vi "Algorithms.vi"(0 "Algo In":T2 {"Measurement ROI.Measurement ROI array"."Multi Threshold Data"."Replace Value" format="%.2f"; "Measurement ROI.Measurement ROI array"."Multi Threshold Data"."Upper value" format="%.2f"; "Measurement ROI.Measurement ROI array"."Multi Threshold Data"."Lower value" format="%.2f"; "Measurement ROI.Measurement ROI array"."Edge Options"."Edge Polarity" items=["All Edges", "Rising Edges", "Falling Edges"]; "Measurement ROI.Measurement ROI array"."Edge Options"."Minimum Edge Strength" format="%.2f"; "Measurement ROI.Measurement ROI array"."Edge Options"."Width" step=2; "Measurement ROI.Measurement ROI array"."Edge Options"."Kernel Size" step=2; "Measurement ROI.Measurement ROI array"."Line Options"."Min. Points (%)" min=0.0 max=100.0; "Measurement ROI.Measurement ROI array"."Line Options"."Min. SNR (db)" min=0.0; "Measurement ROI.Measurement ROI array"."Line Options"."Max. Score" min=0.0 max=1024.0; "Measurement ROI.Measurement ROI array"."Line Options"."Min. Score" min=0.0 max=1024.0 step=1.0; "Measurement ROI.Measurement ROI array"."Shape Detection Settings"."Curve Parameters"."Max Endpoint Gap" min=0; "Measurement ROI.Measurement ROI array"."Shape Detection Settings"."Curve Parameters"."Col Search Step Size" min=1 max=255 step=1; "Measurement ROI.Measurement ROI array"."Shape Detection Settings"."Curve Parameters"."Row Search Step Size" min=1 max=255 step=1; "Measurement ROI.Measurement ROI array"."Shape Detection Settings"."Curve Parameters"."Min Length" min=0; "Measurement ROI.Measurement ROI array"."Shape Detection Settings"."Curve Parameters"."Edge Filter Size" items=["Fine", "Normal", "Controur Tracing"]; "Measurement ROI.Measurement ROI array"."Shape Detection Settings"."Curve Parameters"."Edge Threshold" min=1 max=65535 step=1; "Measurement ROI.Measurement ROI array"."Shape Detection Settings"."Curve Parameters"."Extraction Mode" items=["Normal", "Uniform Regions"]; "Measurement ROI.Measurement ROI array"."Shape Detection Settings"."Match Options"."Range Settings"."Match Constraints" items=["Rotation Angle (degrees)", "Scale Factor (%)", "Occlusion (%)"]}, 5 "AlgoOut array IN":T13 {"CircleArrayOUT"."First Edges"."Distance (Real-World)" format="%.2f"; "CircleArrayOUT"."First Edges"."Location (Real-World)"."Y" format="%.2g"; "CircleArrayOUT"."First Edges"."Location (Real-World)"."X" format="%.2f"; "CircleArrayOUT"."First Edges"."Noise" format="%.2f"; "CircleArrayOUT"."First Edges"."Location (Pixel)"."Y" format="%.2g"; "CircleArrayOUT"."First Edges"."Location (Pixel)"."X" format="%.2f"; "CircleArrayOUT"."First Edges"."Strength" format="%.2f"; "CircleArrayOUT"."First Edges"."Distance (Pixel)" format="%.2f"; "Line Array"."Used Edges"."Edge Information"."Distance (Real-World)" format="%.2f"; "Line Array"."Used Edges"."Edge Information"."Location (Real-World)"."Y" format="%.2g"; "Line Array"."Used Edges"."Edge Information"."Location (Real-World)"."X" format="%.2f"; "Line Array"."Used Edges"."Edge Information"."Noise" format="%.2f"; "Line Array"."Used Edges"."Edge Information"."Location (Pixel)"."Y" format="%.2g"; "Line Array"."Used Edges"."Edge Information"."Location (Pixel)"."X" format="%.2f"; "Line Array"."Used Edges"."Edge Information"."Strength" format="%.2f"; "Line Array"."Used Edges"."Edge Information"."Distance (Pixel)" format="%.2f"; "Line Array"."Straight Edges"."Point2 (Real-World)"."Y" format="%.2f"; "Line Array"."Straight Edges"."Point2 (Real-World)"."X" format="%.2f"; "Line Array"."Straight Edges"."Point1 (Real-World)"."Y" format="%.2f"; "Line Array"."Straight Edges"."Point1 (Real-World)"."X" format="%.2f"; "Line Array"."Straight Edges"."Point2 (Pixels)"."Y" format="%.2f"; "Line Array"."Straight Edges"."Point2 (Pixels)"."X" format="%.2f"; "Line Array"."Straight Edges"."Point1 (Pixels)"."Y" format="%.2f"; "Line Array"."Straight Edges"."Point1 (Pixels)"."X" format="%.2f"; "Line Array"."Line"."Point 2"."Y" format="%.2f"; "Line Array"."Line"."Point 2"."X" format="%.2f"; "Line Array"."Line"."Point 1"."Y" format="%.2f"; "Line Array"."Line"."Point 1"."X" format="%.2f"}, 7 "Captured Image Array In":T16(array[cluster]), 9 "Measurement value":T1(array[cluster]), 11 "error in (no error)":errorcluster) -> (4 "AlgoOut Array out":T14 {"CircleArrayOUT"."First Edges"."Distance (Real-World)" format="%.2f"; "CircleArrayOUT"."First Edges"."Location (Real-World)"."Y" format="%.2g"; "CircleArrayOUT"."First Edges"."Location (Real-World)"."X" format="%.2f"; "CircleArrayOUT"."First Edges"."Noise" format="%.2f"; "CircleArrayOUT"."First Edges"."Location (Pixel)"."Y" format="%.2g"; "CircleArrayOUT"."First Edges"."Location (Pixel)"."X" format="%.2f"; "CircleArrayOUT"."First Edges"."Strength" format="%.2f"; "CircleArrayOUT"."First Edges"."Distance (Pixel)" format="%.2f"; "Line Array"."Used Edges"."Edge Information"."Distance (Real-World)" format="%.2f"; "Line Array"."Used Edges"."Edge Information"."Location (Real-World)"."Y" format="%.2g"; "Line Array"."Used Edges"."Edge Information"."Location (Real-World)"."X" format="%.2f"; "Line Array"."Used Edges"."Edge Information"."Noise" format="%.2f"; "Line Array"."Used Edges"."Edge Information"."Location (Pixel)"."Y" format="%.2g"; "Line Array"."Used Edges"."Edge Information"."Location (Pixel)"."X" format="%.2f"; "Line Array"."Used Edges"."Edge Information"."Strength" format="%.2f"; "Line Array"."Used Edges"."Edge Information"."Distance (Pixel)" format="%.2f"; "Line Array"."Straight Edges"."Point2 (Real-World)"."Y" format="%.2f"; "Line Array"."Straight Edges"."Point2 (Real-World)"."X" format="%.2f"; "Line Array"."Straight Edges"."Point1 (Real-World)"."Y" format="%.2f"; "Line Array"."Straight Edges"."Point1 (Real-World)"."X" format="%.2f"; "Line Array"."Straight Edges"."Point2 (Pixels)"."Y" format="%.2f"; "Line Array"."Straight Edges"."Point2 (Pixels)"."X" format="%.2f"; "Line Array"."Straight Edges"."Point1 (Pixels)"."Y" format="%.2f"; "Line Array"."Straight Edges"."Point1 (Pixels)"."X" format="%.2f"; "Line Array"."Line"."Point 2"."Y" format="%.2f"; "Line Array"."Line"."Point 2"."X" format="%.2f"; "Line Array"."Line"."Point 1"."Y" format="%.2f"; "Line Array"."Line"."Point 1"."X" format="%.2f"}, 6 "overlayDetails Out":T12={"Measurment Name"="", "Measurment Type"="", "Measurment Subtype"="", "Angle of rotation"=0.0, "Color"=16860, "Inspect Overlay Coordinate"=[], "Result"=[], "PointForOverlays"={"Line"=[], "Angle"=[], "Circle"=[], "Points"={"Points"=[]}, "Coordinate System"={"Origin"={"X"=0.0, "Y"=0.0}, "Angle (deg)"=0.0, "Axis Reference"=0}, "True position"={"Measurement details"=[], "XY?"=FALSE}}} {"Inspect Overlay Coordinate"."Y" format="%.2f"; "Inspect Overlay Coordinate"."X" format="%.2f"; "PointForOverlays"."Coordinate System"."Axis Reference" items=["Direct", "Indirect"]; "PointForOverlays"."Coordinate System"."Angle (deg)" format="%.2f"; "PointForOverlays"."Coordinate System"."Origin"."Y" format="%.2f"; "PointForOverlays"."Coordinate System"."Origin"."X" format="%.2f"; "PointForOverlays"."Points"."Points"."Y" format="%.2f"; "PointForOverlays"."Points"."Points"."X" format="%.2f"; "PointForOverlays"."Circle"."Point 2"."Y" format="%.2f"; "PointForOverlays"."Circle"."Point 2"."X" format="%.2f"; "PointForOverlays"."Circle"."Point 1"."Y" format="%.2f"; "PointForOverlays"."Circle"."Point 1"."X" format="%.2f"; "PointForOverlays"."Angle"."line2Point2"."Y" format="%.2f"; "PointForOverlays"."Angle"."line2Point2"."X" format="%.2f"; "PointForOverlays"."Angle"."line2Point1"."Y" format="%.2f"; "PointForOverlays"."Angle"."line2Point1"."X" format="%.2f"; "PointForOverlays"."Angle"."line1Point2"."Y" format="%.2f"; "PointForOverlays"."Angle"."line1Point2"."X" format="%.2f"; "PointForOverlays"."Angle"."line1Point1"."Y" format="%.2f"; "PointForOverlays"."Angle"."line1Point1"."X" format="%.2f"; "PointForOverlays"."Angle"."Point 2a"."Y" format="%.2f"; "PointForOverlays"."Angle"."Point 2a"."X" format="%.2f"; "PointForOverlays"."Angle"."Point 1a"."Y" format="%.2f"; "PointForOverlays"."Angle"."Point 1a"."X" format="%.2f"; "PointForOverlays"."Angle"."vertex"."Y" format="%.2f"; "PointForOverlays"."Angle"."vertex"."X" format="%.2f"; "PointForOverlays"."Angle"."Point 2"."Y" format="%.2f"; "PointForOverlays"."Angle"."Point 2"."X" format="%.2f"; "PointForOverlays"."Angle"."Point 1"."Y" format="%.2f"; "PointForOverlays"."Angle"."Point 1"."X" format="%.2f"; "PointForOverlays"."Line"."Point 2"."Y" format="%.2f"; "PointForOverlays"."Line"."Point 2"."X" format="%.2f"; "PointForOverlays"."Line"."Point 1"."Y" format="%.2f"; "PointForOverlays"."Line"."Point 1"."X" format="%.2f"}, 15 "error out":errorcluster)   [LabVIEW 2018]
uses:
  Controls/AlgoOut.ctl
  <vilib>/vision/Measure.llb/Edge New.ctl
  <vilib>/vision/Image Controls.llb/IMAQ Image.ctl
  Controls/AlgoOutArray.ctl
  Overlays/Controls/overlayWithDetails.ctl
  Controls/Algo In.ctl
  Inspection/Controls/Measurement ROI.ctl
  <vilib>/vision/Measure.llb/Edge Options.ctl
  <vilib>/vision/Measure.llb/Edge Polarity.ctl
  <vilib>/vision/Measure.llb/Straight Edge Options.ctl
  <vilib>/vision/Measure.llb/Straight Edge Process.ctl
  <vilib>/vision/Pattern Matching.llb/IMAQ Curve Parameters.ctl
  <vilib>/vision/Shape Detection.llb/ShapeDetectionMatchOptions.ctl
  <vilib>/vision/Pattern Matching.llb/IMAQ Match Range Setting.ctl
  <vilib>/vision/NI_Vision_Development_Module.lvlib
panel:
  # "Range"
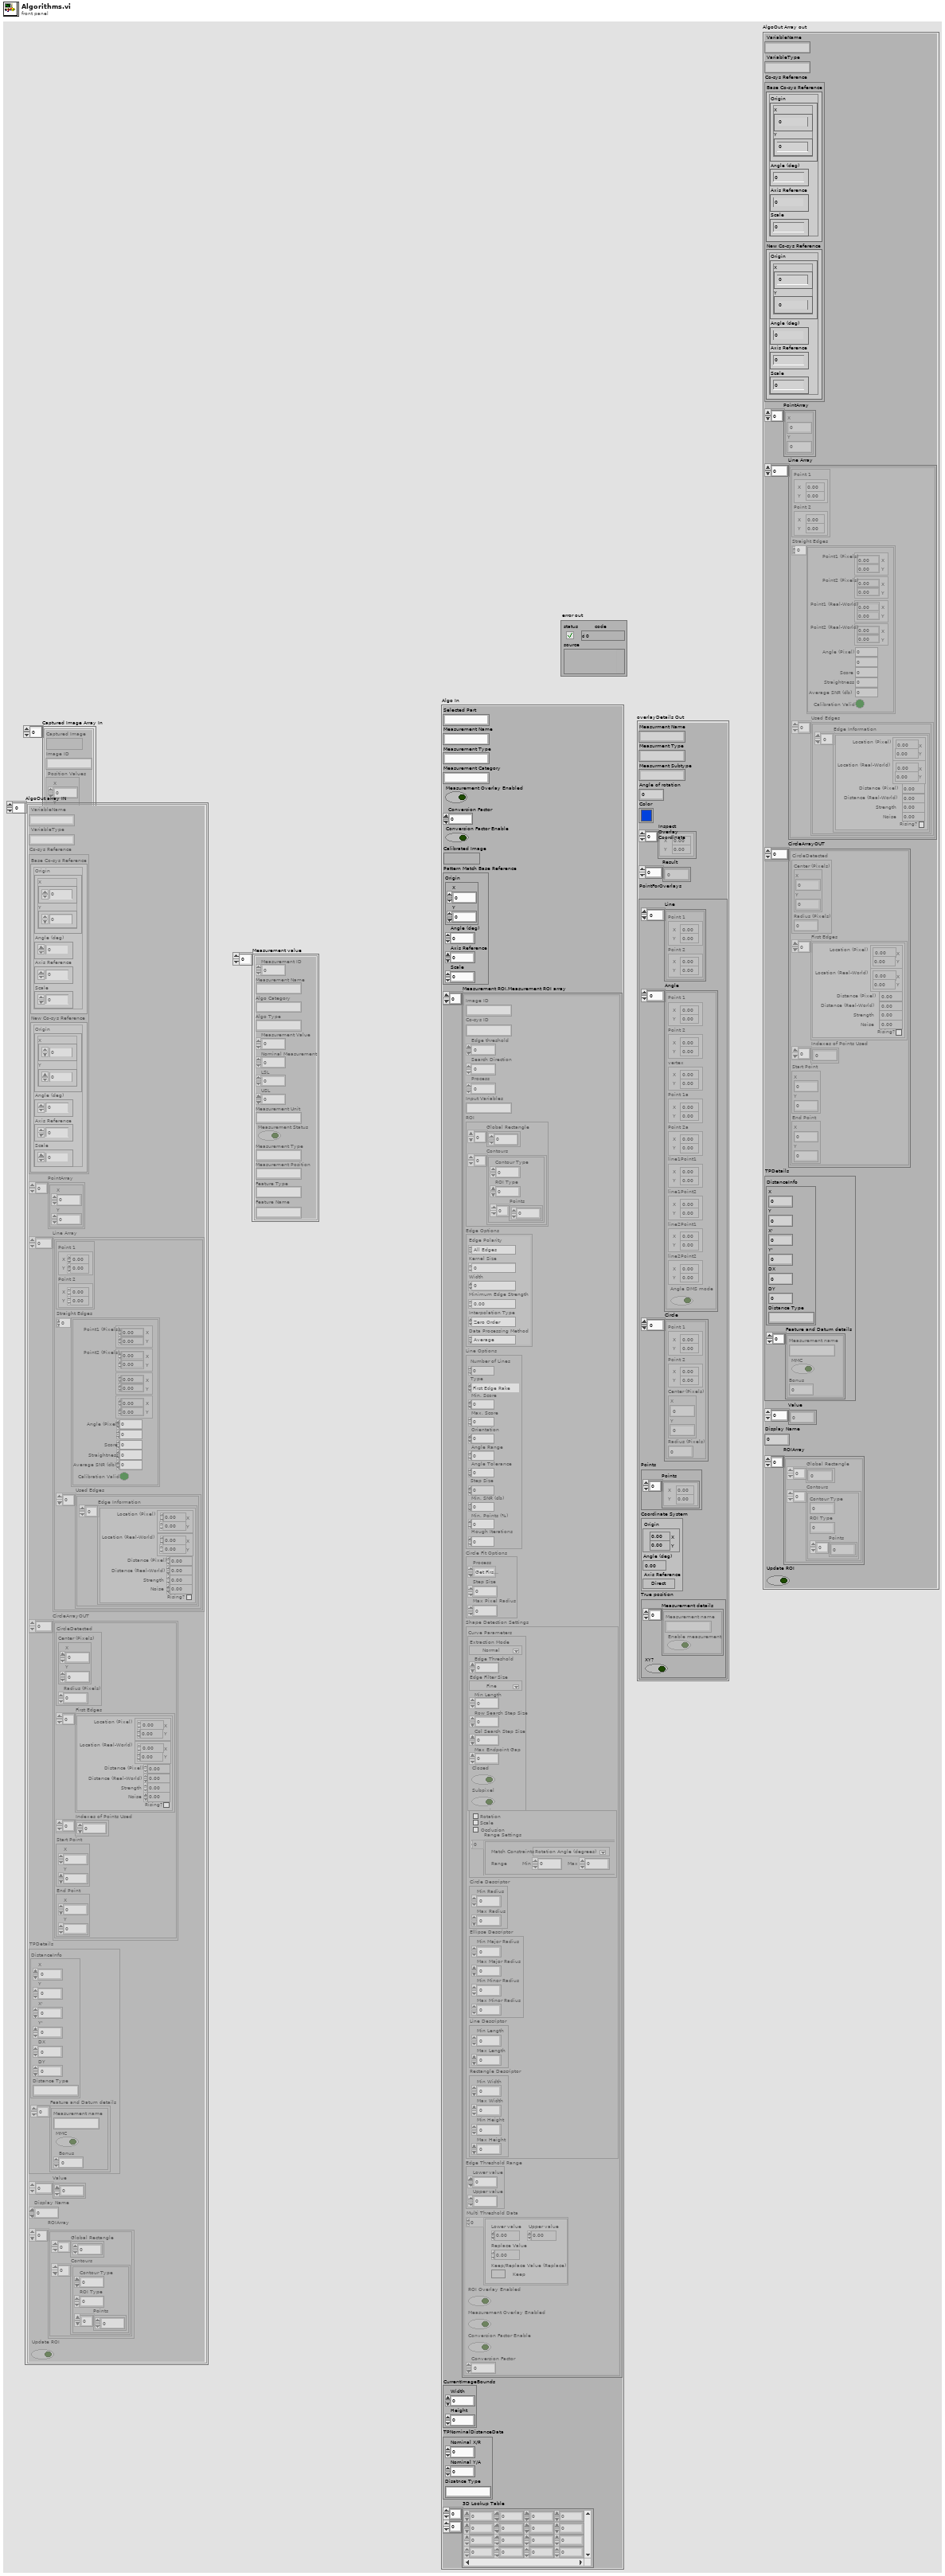
[diagram p1: front panel]
types:
  T1 = cluster{"Measurement ID":u32, "Measurement Name":string, "Algo Category":string, "Algo Type":string, "Measurement Value":dbl, "Nominal Measurement":dbl, "LSL":dbl, "USL":dbl, "Measurement Unit":string, "Measurement Status":bool, "Measurement Type":string, "Measurement Position":string, "Feature Type":string, "Feature Name":string}[]
  T2 = typedef "Algo Sequencer.lvclass/Algo In.ctl" = cluster{"Selected Part":string, "Measurement Name":string, "Measurement Type":string, "Measurement Category":string, "Measurement Overlay Enabled":bool, "Conversion Factor":dbl, "Conversion Factor Enable":bool, "Calibrated Image":T3, "Pattern Match Base Reference":cluster{"Origin":cluster{"X":dbl, "Y":dbl}, "Angle (deg)":dbl, "Axis Reference":dbl, "Scale":dbl}, "Measurement ROI.Measurement ROI array":T4[], "CurrentImageBounds":cluster{"Width":i32, "Height":i32}, "TPNominalDistanceData":cluster{"Nominal X/R":dbl, "Nominal Y/A":dbl, "Disatnce Type":string}, "3D Lookup Table":dbl[][]}
  T3 = typedef "IMAQ Image.ctl" = refnum<image>
  T4 = typedef "Inspection.lvclass/Measurement ROI.ctl" = cluster{"Image ID":string, "Co-sys ID":string, "Edge threshold":dbl, "Search Direction ":u16, "Process":u16, "Input Variables":string, "ROI":cluster{"Global Rectangle":i32[], "Contours":cluster{"Contour Type":u32, "ROI Type":u32, "Points":i32[]}[]}, "Edge Options":T5, "Line Options":T7, "Circle Fit Options ":cluster{"Process":enum16{"Get First Edge", "Get First + Last Edge", "Get All Edges", "Get Best Edge"}, "Step Size":dbl, "Max Pixel Radius":i32}, "Shape Detection Settings":cluster{"Curve Parameters":T9, "Match Options":T10, "Circle Descriptor":cluster{"Min Radius":dbl, "Max Radius":dbl}, "Ellipse Descriptor":cluster{"Min Major Radius":dbl, "Max Major Radius":dbl, "Min Minor Radius":dbl, "Max Minor Radius":dbl}, "Line Descriptor":cluster{"Min Length":dbl, "Max Length":dbl}, "Rectangle Descriptor":cluster{"Min Width":dbl, "Max Width":dbl, "Min Height":dbl, "Max Height":dbl}}, "Edge Threshold Range":cluster{"Lower value":sgl, "Upper value":sgl}, "Multi Threshold Data":cluster{"Lower value":sgl, "Upper value":sgl, "Replace Value":sgl, "Keep/Replace Value (Replace)":bool}[], "ROI Overlay Enabled":bool, "Measurement Overlay Enabled":bool, "Conversion Factor Enable":bool, "Conversion Factor":dbl}
  T5 = typedef "Edge Options.ctl" = cluster{"Edge Polarity":T6, "Kernel Size":u32, "Width":u32, "Minimum Edge Strength":sgl, "Interpolation Type":enum32{"Zero Order", "Bilinear", "Quadratic", "Cubic", "Bilinear Fixed"}, "Data Processing Method":enum32{"Average", "Median"}}
  T6 = typedef "Edge Polarity.ctl" = u32
  T7 = typedef "Straight Edge Options.ctl" = cluster{"Number of Lines":i32, "Type":T8, "Min. Score":dbl, "Max. Score":dbl, "Orientation":dbl, "Angle Range":dbl, "Angle Tolerance":dbl, "Step Size":u32, "Min. SNR (db)":dbl, "Min. Points (%)":dbl, "Hough Iterations":i32}
  T8 = typedef "Straight Edge Process.ctl" = enum32{"First Edge Rake", "Best Edge Rake", "Hough Edge Rake", "First Edge Projection", "Best Edge Projection"}
  T9 = typedef "IMAQ Curve Parameters.ctl" = cluster{"Extraction Mode":u32, "Edge Threshold":i32, "Edge Filter Size":u32, "Min Length":i32, "Row Search Step Size":i32, "Col Search Step Size":i32, "Max Endpoint Gap":i32, "Closed":bool, "Subpixel":bool}
  T10 = typedef "ShapeDetectionMatchOptions.ctl" = cluster{"Rotation":bool, "Scale":bool, "Occlusion":bool, "Range Settings":T11[]}
  T11 = typedef "IMAQ Match Range Setting.ctl" = cluster{"Match Constraints":u32, "Min":dbl, "Max":dbl}
  T12 = typedef "overlayWithDetails.ctl" = cluster{"Measurment Name":string, "Measurment Type":string, "Measurment Subtype":string, "Angle of rotation":dbl, "Color":u32, "Inspect Overlay Coordinate":cluster{"X":sgl, "Y":sgl}[], "Result":sgl[], "PointForOverlays":cluster{"Line":cluster{"Point 1":cluster{"X":sgl, "Y":sgl}, "Point 2":cluster{"X":sgl, "Y":sgl}}[], "Angle":cluster{"Point 1":cluster{"X":sgl, "Y":sgl}, "Point 2":cluster{"X":sgl, "Y":sgl}, "vertex":cluster{"X":sgl, "Y":sgl}, "Point 1a":cluster{"X":sgl, "Y":sgl}, "Point 2a":cluster{"X":sgl, "Y":sgl}, "line1Point1":cluster{"X":sgl, "Y":sgl}, "line1Point2":cluster{"X":sgl, "Y":sgl}, "line2Point1":cluster{"X":sgl, "Y":sgl}, "line2Point2":cluster{"X":sgl, "Y":sgl}, "Angle DMS mode":bool}[], "Circle":cluster{"Point 1":cluster{"X":sgl, "Y":sgl}, "Point 2":cluster{"X":sgl, "Y":sgl}, "Center (Pixels)":cluster{"X":sgl, "Y":sgl}, "Radius (Pixels)":dbl}[], "Points":cluster{"Points":cluster{"X":sgl, "Y":sgl}[]}, "Coordinate System":cluster{"Origin":cluster{"X":sgl, "Y":sgl}, "Angle (deg)":sgl, "Axis Reference":u32}, "True position":cluster{"Measurement details":cluster{"Measurement name":string, "Enable measurement":bool}[], "XY?":bool}}}
  T13 = typedef "Algo Sequencer.lvclass/AlgoOutArray.ctl" = T14[]
  T14 = typedef "Algo Sequencer.lvclass/AlgoOut.ctl" = cluster{"VariableName":string, "VariableType":string, "Co-sys Reference":cluster{"Base Co-sys Reference":cluster{"Origin":cluster{"X":sgl, "Y":sgl}, "Angle (deg)":sgl, "Axis Reference":u32, "Scale":sgl}, "New Co-sys Reference":cluster{"Origin":cluster{"X":sgl, "Y":sgl}, "Angle (deg)":sgl, "Axis Reference":u32, "Scale":sgl}}, "PointArray":cluster{"X":sgl, "Y":sgl}[], "Line Array":cluster{"Line":cluster{"Point 1":cluster{"X":sgl, "Y":sgl}, "Point 2":cluster{"X":sgl, "Y":sgl}}, "Straight Edges":cluster{"Point1 (Pixels)":cluster{"X":sgl, "Y":sgl}, "Point2 (Pixels)":cluster{"X":sgl, "Y":sgl}, "Point1 (Real-World)":cluster{"X":sgl, "Y":sgl}, "Point2 (Real-World)":cluster{"X":sgl, "Y":sgl}, "Angle (Pixel)":dbl, "Angle (Real-World)":dbl, "Score":dbl, "Straightness":dbl, "Average SNR (db)":dbl, "Calibration Valid":bool}[], "Used Edges":cluster{"Edge Information":T15[]}[]}[], "CircleArrayOUT":cluster{"CircleDetected":cluster{"Center (Pixels)":cluster{"X":sgl, "Y":sgl}, "Radius (Pixels)":dbl}, "First Edges":T15[], "Indexes of Points Used":i32[], "Start Point":cluster{"X":sgl, "Y":sgl}, "End Point":cluster{"X":sgl, "Y":sgl}}[], "TPDetails":cluster{"DistanceInfo":cluster{"X":dbl, "Y":dbl, "X'":dbl, "Y'":dbl, "DX":dbl, "DY":dbl, "Distance Type":string}, "Feature and Datum details":cluster{"Measurement name":string, "MMC":bool, "Bonus":dbl}[]}, "Value":sgl[], "Display Name":sgl, "ROIArray":cluster{"Global Rectangle":i32[], "Contours":cluster{"Contour Type":u32, "ROI Type":u32, "Points":i32[]}[]}[], "Update ROI ":bool}
  T15 = typedef "Edge New.ctl" = cluster{"Location (Pixel)":cluster{"X":sgl, "Y":sgl}, "Location (Real-World)":cluster{"X":sgl, "Y":sgl}, "Distance (Pixel)":dbl, "Distance (Real-World)":dbl, "Strength":dbl, "Noise":dbl, "Rising?":bool}
  T16 = cluster{"Captured Image":T3, "Image ID":string, " Position Values":cluster{"X":sgl, "Y":sgl, "Z":sgl}}[]
  T17 = cluster{"Global Rectangle":i32[], "Contours":cluster{"Contour Type":u32, "ROI Type":u32, "Points":i32[]}[]}[]
  T18 = cluster{"Line":cluster{"Point 1":cluster{"X":sgl, "Y":sgl}, "Point 2":cluster{"X":sgl, "Y":sgl}}, "Straight Edges":cluster{"Point1 (Pixels)":cluster{"X":sgl, "Y":sgl}, "Point2 (Pixels)":cluster{"X":sgl, "Y":sgl}, "Point1 (Real-World)":cluster{"X":sgl, "Y":sgl}, "Point2 (Real-World)":cluster{"X":sgl, "Y":sgl}, "Angle (Pixel)":dbl, "Angle (Real-World)":dbl, "Score":dbl, "Straightness":dbl, "Average SNR (db)":dbl, "Calibration Valid":bool}[], "Used Edges":cluster{"Edge Information":T15[]}[]}[]
  T19 = cluster{"CircleDetected":cluster{"Center (Pixels)":cluster{"X":sgl, "Y":sgl}, "Radius (Pixels)":dbl}, "First Edges":T15[], "Indexes of Points Used":i32[], "Start Point":cluster{"X":sgl, "Y":sgl}, "End Point":cluster{"X":sgl, "Y":sgl}}[]
  T20 = cluster{"Base Co-sys Reference":cluster{"Origin":cluster{"X":sgl, "Y":sgl}, "Angle (deg)":sgl, "Axis Reference":u32, "Scale":sgl}, "New Co-sys Reference":cluster{"Origin":cluster{"X":sgl, "Y":sgl}, "Angle (deg)":sgl, "Axis Reference":u32, "Scale":sgl}}
  T21 = cluster{"Origin":cluster{"X":dbl, "Y":dbl}, "Angle (deg)":dbl, "Axis Reference":dbl, "Scale":dbl}
  T22 = cluster{"Nominal X/R":dbl, "Nominal Y/A":dbl, "Disatnce Type":string}
  T23 = cluster{"Line":cluster{"Point 1":cluster{"X":sgl, "Y":sgl}, "Point 2":cluster{"X":sgl, "Y":sgl}}, "Straight Edges":cluster{"Point1 (Pixels)":cluster{"X":sgl, "Y":sgl}, "Point2 (Pixels)":cluster{"X":sgl, "Y":sgl}, "Point1 (Real-World)":cluster{"X":sgl, "Y":sgl}, "Point2 (Real-World)":cluster{"X":sgl, "Y":sgl}, "Angle (Pixel)":dbl, "Angle (Real-World)":dbl, "Score":dbl, "Straightness":dbl, "Average SNR (db)":dbl, "Calibration Valid":bool}[], "Used Edges":cluster{"Edge Information":T15[]}[]}
  T24 = cluster{"Point 1":cluster{"X":sgl, "Y":sgl}, "Point 2":cluster{"X":sgl, "Y":sgl}}
  T25 = cluster{"Point 1":cluster{"Start X":dbl, "Start Y":dbl}, "Point 2":cluster{"End X":dbl, "End Y":dbl}}
  T26 = cluster{"CircleDetected":cluster{"Center (Pixels)":cluster{"X":sgl, "Y":sgl}, "Radius (Pixels)":dbl}, "First Edges":T15[], "Indexes of Points Used":i32[], "Start Point":cluster{"X":sgl, "Y":sgl}, "End Point":cluster{"X":sgl, "Y":sgl}}
  T27 = cluster{"CircleDetected":cluster{"Center (Pixels)":cluster{"X":dbl, "Y":dbl}, "Radius (Pixels)":dbl}, "First Edges":T15[], "Indexes of Points Used":i32[], "Start Point":cluster{"X":sgl, "Y":sgl}, "End Point":cluster{"X":sgl, "Y":sgl}}[]
  T28 = cluster{"Point 1":cluster{"X":sgl, "Y":sgl}, "Point 2":cluster{"X":sgl, "Y":sgl}, "Center (Pixels)":cluster{"X":sgl, "Y":sgl}, "Radius (Pixels)":dbl}[]
  T29 = cluster{"Center":cluster{"X":sgl, "Y":sgl}, "Radius":dbl}
  T30 = cluster{"CircleDetected":cluster{"Center (Pixels)":cluster{"X":dbl, "Y":dbl}, "Radius (Pixels)":dbl}, "First Edges":T15[], "Indexes of Points Used":i32[], "Start Point":cluster{"X":sgl, "Y":sgl}, "End Point":cluster{"X":sgl, "Y":sgl}}
  T31 = cluster{"Point 1":cluster{"X":sgl, "Y":sgl}, "Point 2":cluster{"X":sgl, "Y":sgl}}[]
  T32 = cluster{"Point1 (Pixels)":cluster{"X":sgl, "Y":sgl}, "Point2 (Pixels)":cluster{"X":sgl, "Y":sgl}}
  T33 = cluster{"Point 1 (Pixel)":cluster{"X":sgl, "Y":sgl}, "Point 2 (Pixel)":cluster{"X":sgl, "Y":sgl}}
  T34 = cluster{"Point 1":cluster{"X":sgl, "Y":sgl}, "Point 2":cluster{"X":sgl, "Y":sgl}, "vertex":cluster{"X":sgl, "Y":sgl}, "Point 1a":cluster{"X":sgl, "Y":sgl}, "Point 2a":cluster{"X":sgl, "Y":sgl}, "line1Point1":cluster{"X":sgl, "Y":sgl}, "line1Point2":cluster{"X":sgl, "Y":sgl}, "line2Point1":cluster{"X":sgl, "Y":sgl}, "line2Point2":cluster{"X":sgl, "Y":sgl}, "Angle DMS mode":bool}
  T35 = cluster{"Point 1":cluster{"X":sgl, "Y":sgl}, "Point 2":cluster{"X":sgl, "Y":sgl}, "Center (Pixels)":cluster{"X":sgl, "Y":sgl}, "Radius (Pixels)":dbl}
  T36 = typedef "IMAQ Line" = cluster{"Start X":i32, "Start Y":i32, "End X":i32, "End Y":i32}
  T37 = cluster{"Search Direction":u32, "Edge Options":T5, "Line Options":T7}
  T38 = typedef "IMAQ Rectangle" = cluster{"Left":i32, "Top":i32, "Right":i32, "Bottom":i32, "Rotation":dbl}
  T39 = cluster{"Options":cluster{"Search Direction":u32, "Edge Options":T5, "Show Search Area":bool, "Show Search Lines":bool, "Show Edges Found":bool, "Show Result":bool, "Search Area Color":u32, "Search Lines Color":u32, "Edge Locations Color":u32, "Result Color":u32, "Overlay Group Name":string}, "Line Fit Options":T7}
  T40 = cluster{"Measurement name":string, "MMC":bool, "Bonus":dbl}
  T41 = cluster{"Measurement name":string, "Enable measurement":bool}
  T42 = cluster{"Captured Image":T3, "Image ID":string, " Position Values":cluster{"X":sgl, "Y":sgl, "Z":sgl}}
  T43 = cluster{"Origin":cluster{"X":sgl, "Y":sgl}, "Angle (deg)":sgl, "Axis Reference":u32}
  T44 = cluster{"Origin":cluster{"X":sgl, "Y":sgl}, "Angle (deg)":sgl, "Axis Reference":u32, "Angle (deg) 2":sgl}
  T45 = cluster{"Origin":cluster{"X":sgl, "Y":sgl}, "Angle (deg)":sgl, "Axis Reference":u32, "Scale":sgl}
  T46 = cluster{"Edge Options":T5, "Process":enum16{"Get First Edge", "Get First + Last Edge", "Get All Edges", "Get Best Edge"}}
  T47 = cluster{"Global Rectangle":i32[], "Contours":cluster{"Contour Type":u32, "ROI Type":u32, "Points":i32[]}[]}
  T48 = cluster{"Center (Pixels)":cluster{"X":sgl, "Y":sgl}, "Radius (Pixels)":dbl}
  T49 = cluster{"Point 1":cluster{"X":bool, "Y":bool}, "Point 2":cluster{"X":bool, "Y":bool}}
  T50 = cluster{"Center (Pixels)":cluster{"X":bool, "Y":bool}, "Radius (Pixels)":bool}
  T51 = typedef "ROI Descriptor" = cluster{"Global Rectangle":i32[], "Contours":cluster{"ID":enum32{"External", "Internal"}, "Type":u32, "Coordinates":i32[]}[]}
  T52 = cluster{"Point1 (Pixels)":cluster{"X":sgl, "Y":sgl}, "Point2 (Pixels)":cluster{"X":sgl, "Y":sgl}, "Point1 (Real-World)":cluster{"X":sgl, "Y":sgl}, "Point2 (Real-World)":cluster{"X":sgl, "Y":sgl}, "Angle (Pixel)":dbl, "Angle (Real-World)":dbl, "Score":dbl, "Straightness":dbl, "Average SNR (db)":dbl, "Calibration Valid":bool}[]
  T53 = cluster{"s? t:f":cluster{"X":dbl, "Y":dbl}, "s? t:f":cluster{"X":dbl, "Y":dbl}}
  T54 = cluster{cluster{"s? t:f":cluster{"X":dbl, "Y":dbl}, "s? t:f":cluster{"X":dbl, "Y":dbl}}, "Straight Edges":cluster{"Point1 (Pixels)":cluster{"X":sgl, "Y":sgl}, "Point2 (Pixels)":cluster{"X":sgl, "Y":sgl}, "Point1 (Real-World)":cluster{"X":sgl, "Y":sgl}, "Point2 (Real-World)":cluster{"X":sgl, "Y":sgl}, "Angle (Pixel)":dbl, "Angle (Real-World)":dbl, "Score":dbl, "Straightness":dbl, "Average SNR (db)":dbl, "Calibration Valid":bool}[], "Used Edges":cluster{"Edge Information":T15[]}[]}
  T55 = cluster{cluster{"s? t:f":cluster{"X":dbl, "Y":dbl}, "s? t:f":cluster{"X":dbl, "Y":dbl}}, "Straight Edges":cluster{"Point1 (Pixels)":cluster{"X":sgl, "Y":sgl}, "Point2 (Pixels)":cluster{"X":sgl, "Y":sgl}, "Point1 (Real-World)":cluster{"X":sgl, "Y":sgl}, "Point2 (Real-World)":cluster{"X":sgl, "Y":sgl}, "Angle (Pixel)":dbl, "Angle (Real-World)":dbl, "Score":dbl, "Straightness":dbl, "Average SNR (db)":dbl, "Calibration Valid":bool}[], "Used Edges":cluster{"Edge Information":T15[]}[]}[]
  T56 = cluster{"s? t:f":cluster{"X":dbl, "Y":dbl}, "s? t:f":cluster{"X":dbl, "Y":dbl}}[]
  T57 = cluster{"Point 1":cluster{"Start X":i32, "Start Y":i32}, "Point 2":cluster{"End X":i32, "End Y":i32}}
  T58 = cluster{"Point 1":cluster{"Start X":dbl, "Start Y":dbl}, "Point 2":cluster{"End X":dbl, "End Y":dbl}}[]
  T59 = cluster{"Options":cluster{"Search  Direction":u32, "Edge Options":T5, "Show Search Area":bool, "Show Search Lines":bool, "Show Edges Found":bool, "Show Result":bool, "Search Area Color":u32, "Search Lines Color":u32, "Edge Locations Color":u32, "Result Color":u32, "Overlay Group Name":string}, "Circle Fit Options":cluster{"Process":enum16{"Get First Edge", "Get First + Last Edge", "Get All Edges", "Get Best Edge"}, "Step Size":dbl, "Max Pixel Radius":i32}}
  T60 = cluster{"Process":enum16{"Get First Edge", "Get First + Last Edge", "Get All Edges", "Get Best Edge"}, "Step Size":dbl, "Max Pixel Radius":i32}
  T61 = cluster{"CircleDetected":cluster{"Center (Pixels)":cluster{"X":sgl, "Y":sgl}, "Radius (Pixels)":dbl}, "First Edges":T15[], "Indexes of Points Used":i32[]}[]
  T62 = cluster{"Edge Options":T5, "Scan Direction":u16, "Process":enum16{"Get First Edge", "Get First + Last Edge", "Get All Edges", "Get Best Edge"}, "Step Size":dbl}
  T63 = cluster{"Curve Parameters":T9, "Match Options":T10, "Circle Descriptor":cluster{"Min Radius":dbl, "Max Radius":dbl}, "Ellipse Descriptor":cluster{"Min Major Radius":dbl, "Max Major Radius":dbl, "Min Minor Radius":dbl, "Max Minor Radius":dbl}, "Line Descriptor":cluster{"Min Length":dbl, "Max Length":dbl}, "Rectangle Descriptor":cluster{"Min Width":dbl, "Max Width":dbl, "Min Height":dbl, "Max Height":dbl}}
  T64 = cluster{"Point1 (Pixels)":cluster{"X":sgl, "Y":sgl}, "Point2 (Pixels)":cluster{"X":sgl, "Y":sgl}}[]
  T65 = cluster{"Point 1":cluster{"X":sgl, "Y":sgl}, "Point 2":cluster{"X":sgl, "Y":sgl}, "vertex":cluster{"X":sgl, "Y":sgl}, "Point 1a":cluster{"X":sgl, "Y":sgl}, "Point 2a":cluster{"X":sgl, "Y":sgl}, "line1Point1":cluster{"X":sgl, "Y":sgl}, "line1Point2":cluster{"X":sgl, "Y":sgl}, "line2Point1":cluster{"X":sgl, "Y":sgl}, "line2Point2":cluster{"X":sgl, "Y":sgl}, "Angle DMS mode":bool}[]
  T66 = cluster{"XL":dbl, "YL":dbl, "Xmi":dbl, "Ymi":dbl}
  T67 = cluster{"Line":cluster{"Point 1":cluster{"X":bool, "Y":bool}, "Point 2":cluster{"X":bool, "Y":bool}}, "Straight Edges":cluster{"Point1 (Pixels)":cluster{"X":bool, "Y":bool}, "Point2 (Pixels)":cluster{"X":bool, "Y":bool}, "Point1 (Real-World)":cluster{"X":bool, "Y":bool}, "Point2 (Real-World)":cluster{"X":bool, "Y":bool}, "Angle (Pixel)":bool, "Angle (Real-World)":bool, "Score":bool, "Straightness":bool, "Average SNR (db)":bool, "Calibration Valid":bool}[], "Used Edges":cluster{"Edge Information":cluster{"Location (Pixel)":cluster{"X":bool, "Y":bool}, "Location (Real-World)":cluster{"X":bool, "Y":bool}, "Distance (Pixel)":bool, "Distance (Real-World)":bool, "Strength":bool, "Noise":bool, "Rising?":bool}[]}[]}
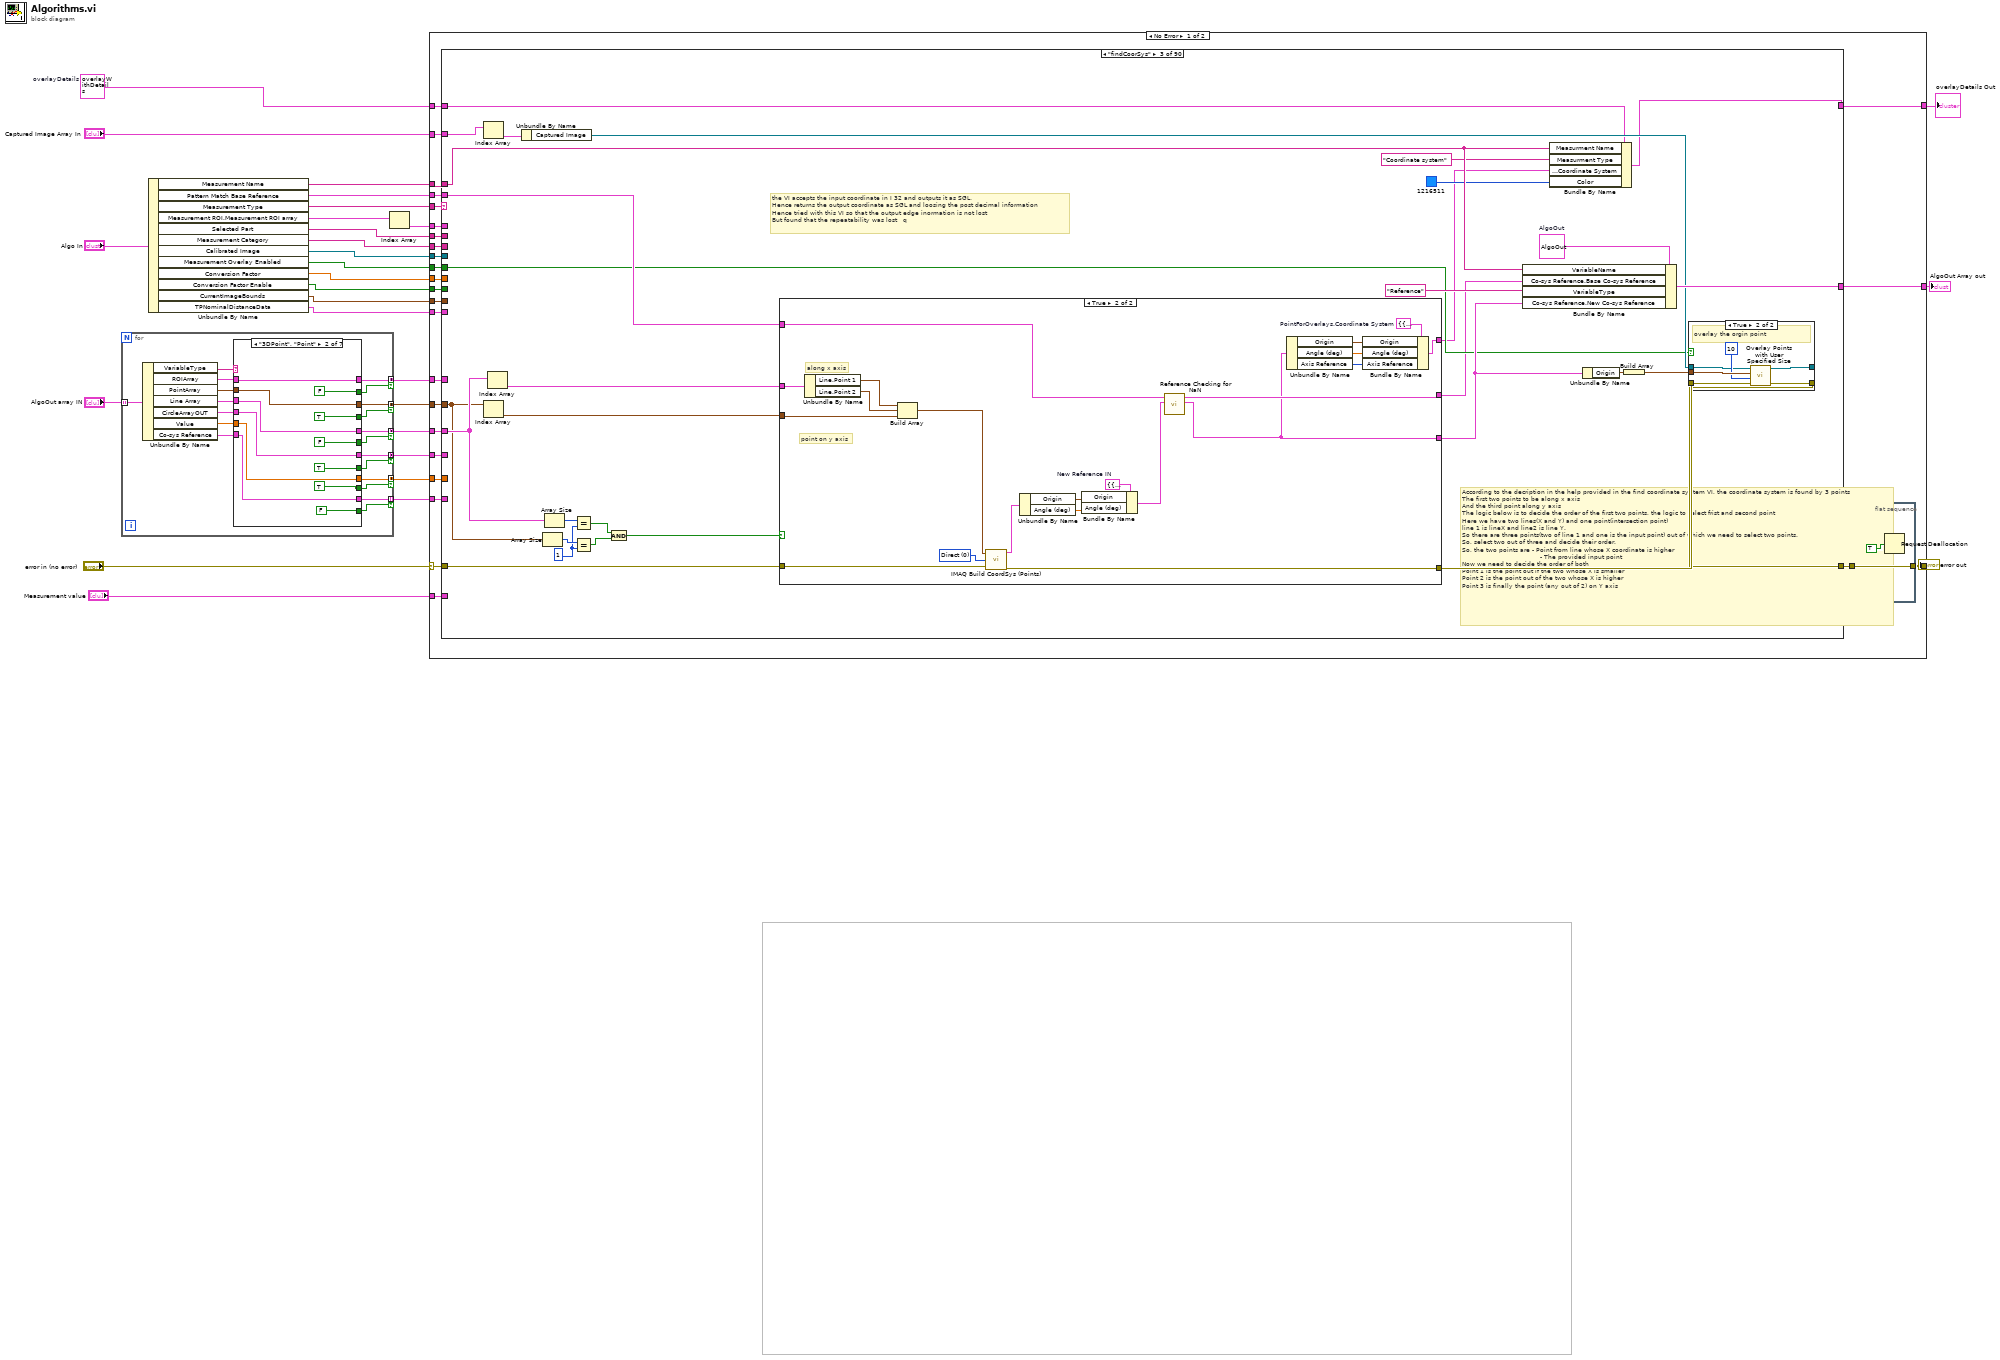
[diagram p0: block diagram]
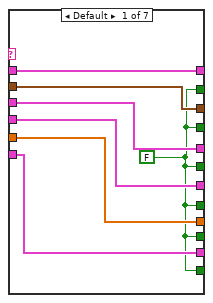
[diagram p2: hidden frame]
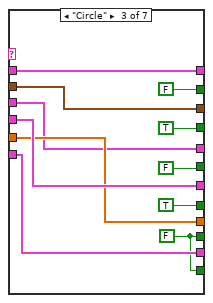
[diagram p3: hidden frame]
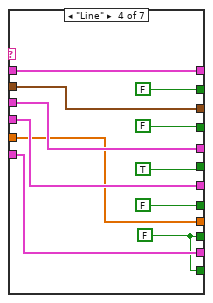
[diagram p4: hidden frame]
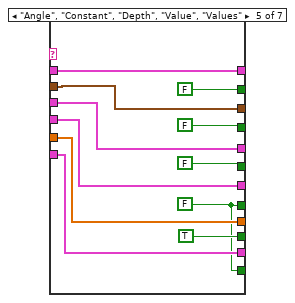
[diagram p5: hidden frame]
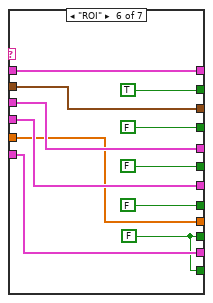
[diagram p6: hidden frame]
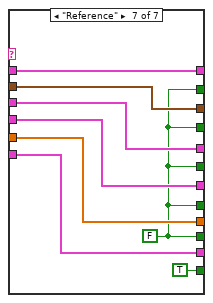
[diagram p7: hidden frame]
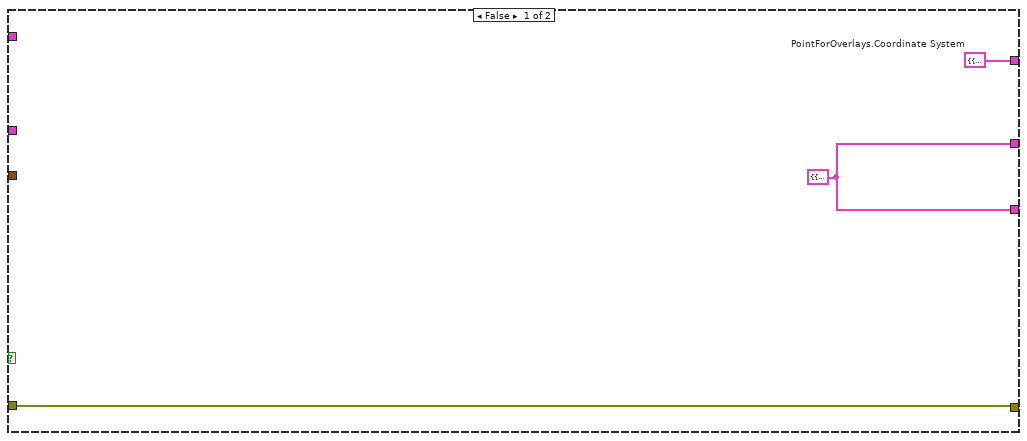
[diagram p10: hidden frame]
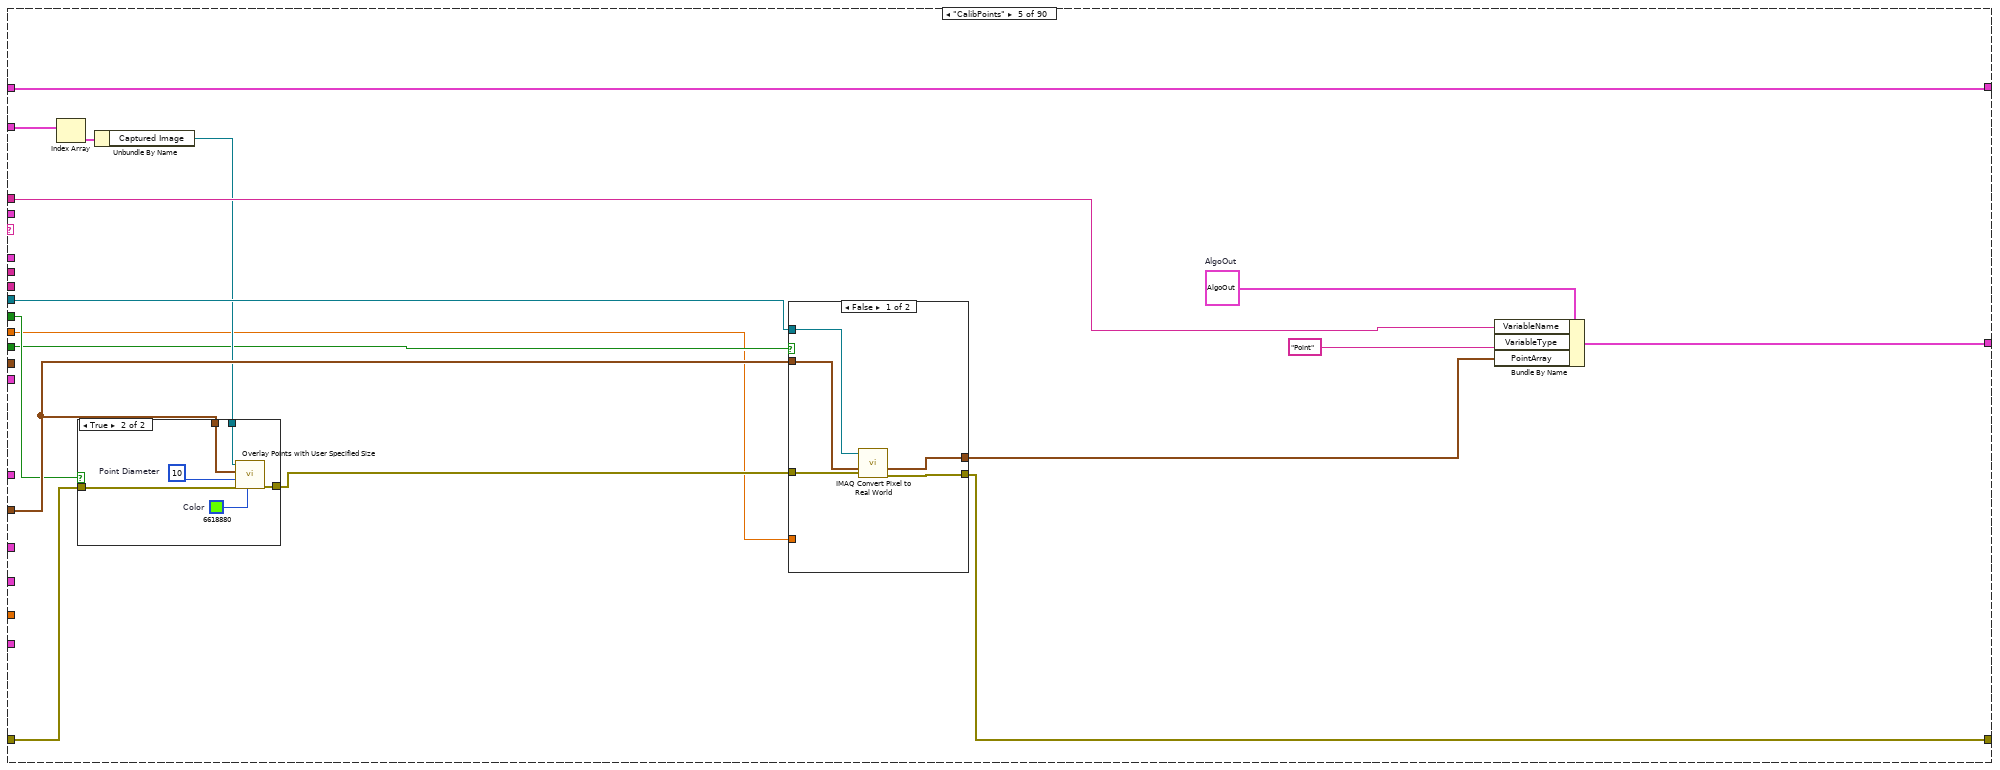
[diagram p13: hidden frame]
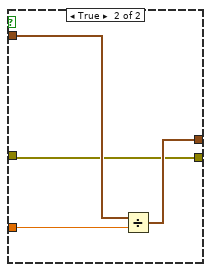
[diagram p14: hidden frame]
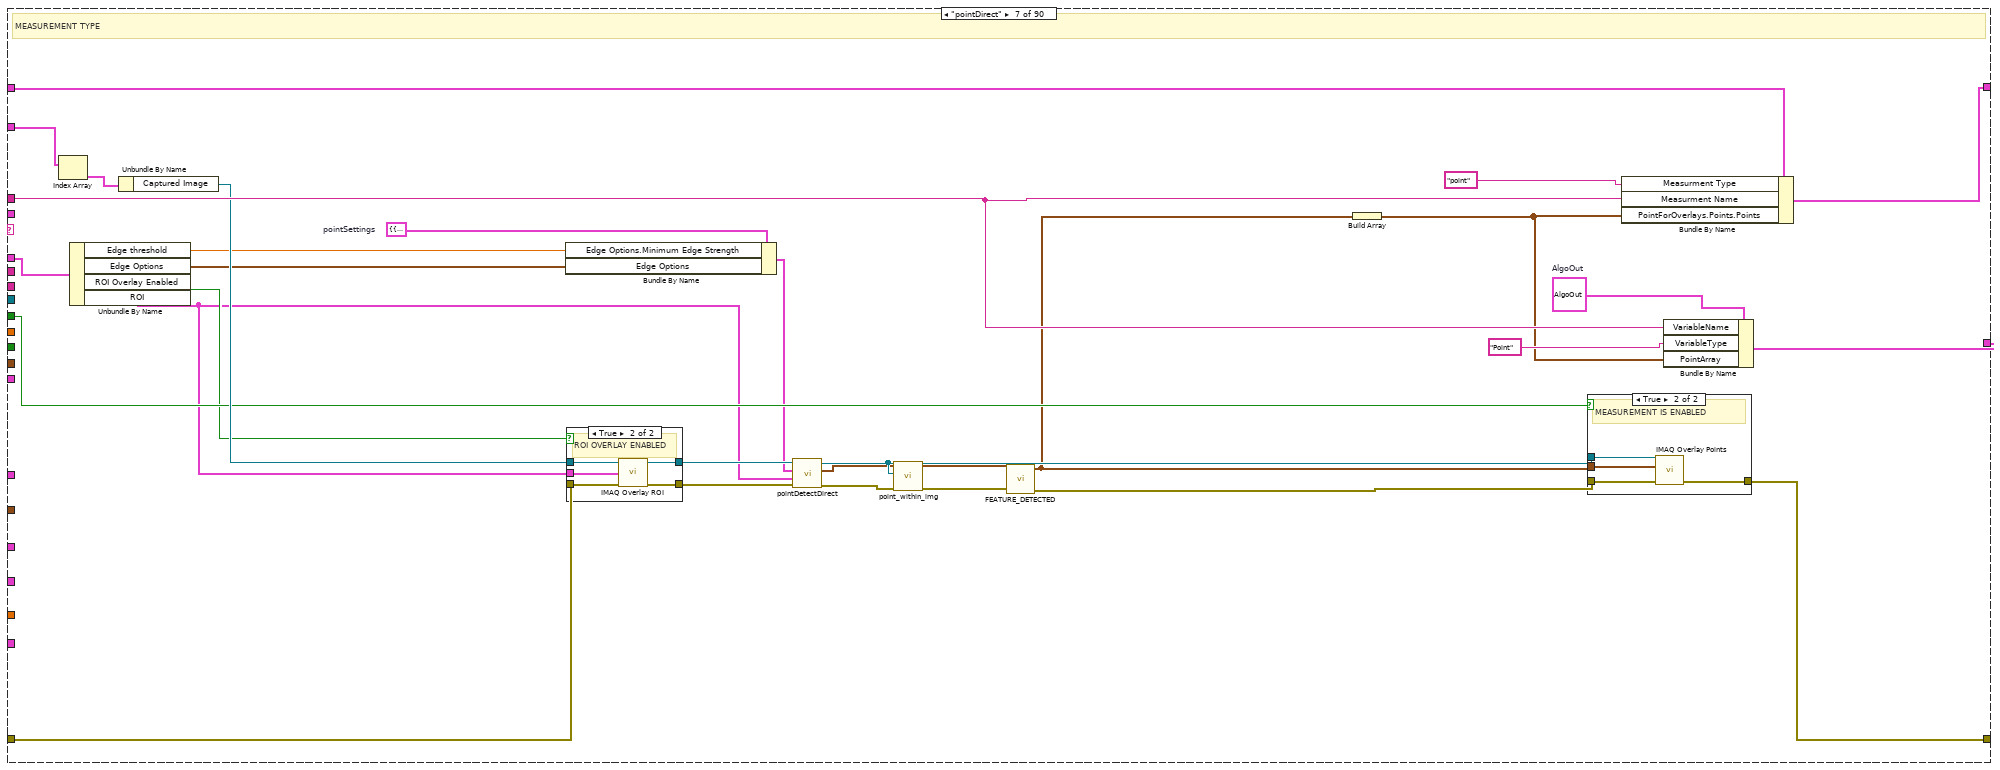
[diagram p17: hidden frame]
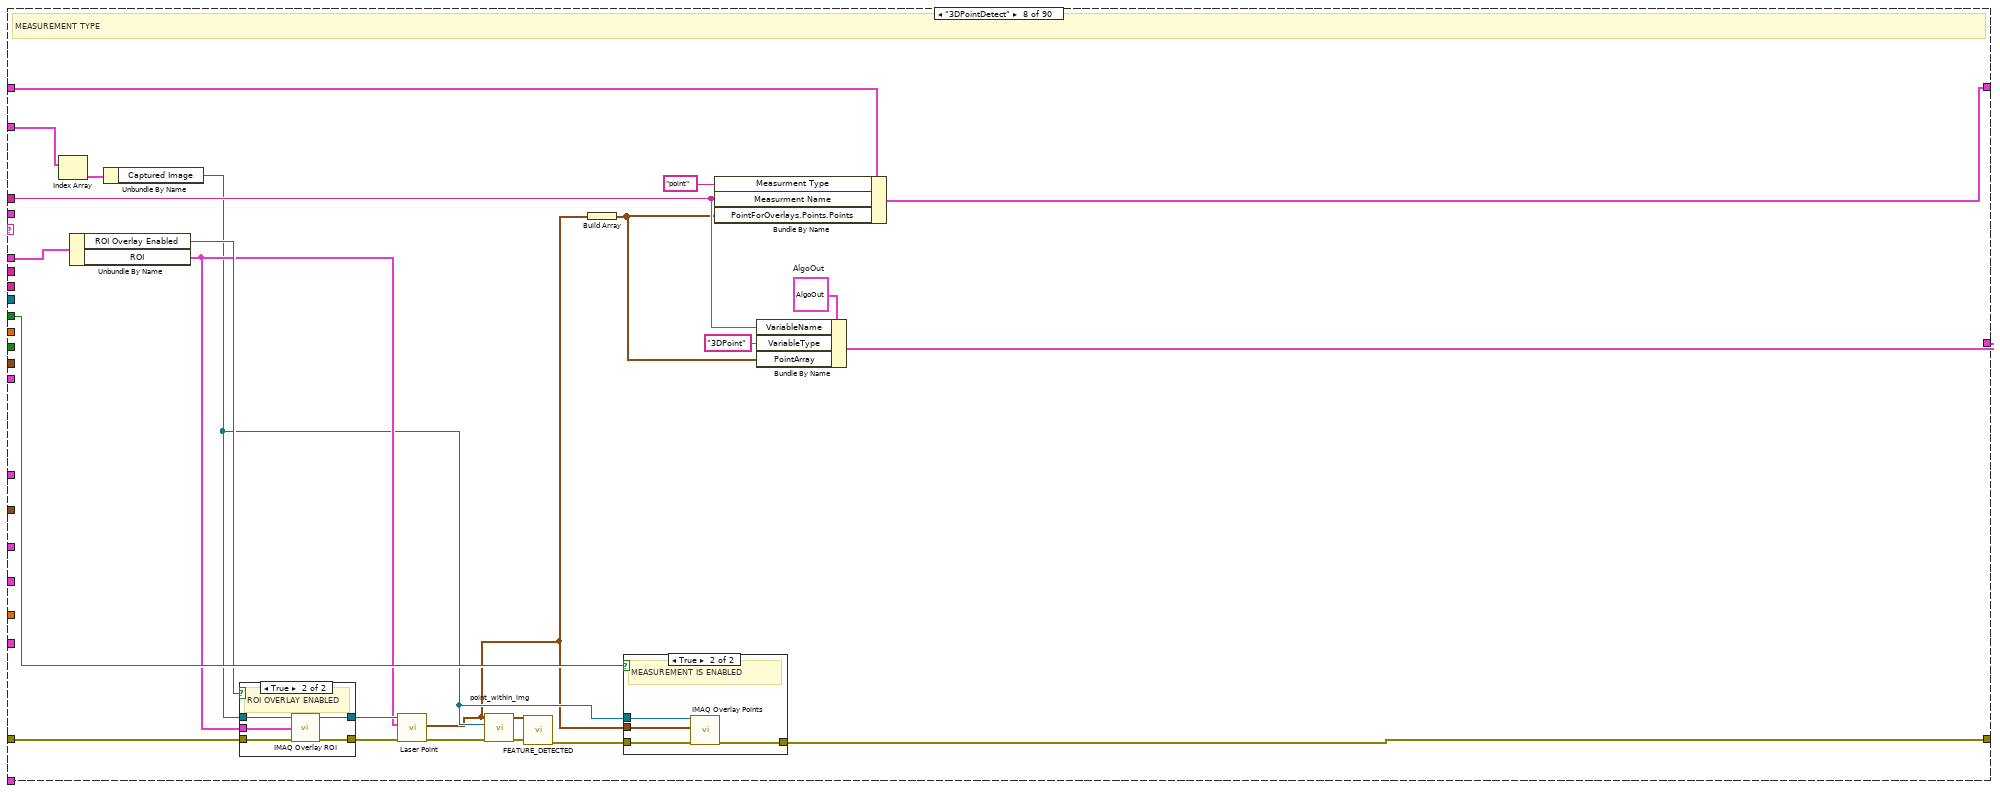
[diagram p20: hidden frame]
diagram:
  w17 = T12 {"Measurment Name"="", "Measurment Type"="", "Measurment Subtype"="", "Angle of rotation"=0.0, "Color"=16748288, "Inspect Overlay Coordinate"=[], "Result"=[], "PointForOverlays"={"Line"=[], "Angle"=[], "Circle"=[], "Points"={"Points"=[]}, "Coordinate System"={"Origin"={"X"=0.0, "Y"=0.0}, "Angle (deg)"=0.0, "Axis Reference"=0}, "True position"={"Measurement details"=[], "XY?"=FALSE}}}  # overlayDetails
  n1 = for {
    tunnel: "AlgoOut array IN" -> [w48] mode=indexing
    tunnel: [w45] -> w21 mode=concatenating if=w41
    tunnel: [w44] -> w20 mode=concatenating if=w42
    tunnel: [w35] -> w19 mode=concatenating if=w43
    tunnel: [w39] -> w22 mode=concatenating if=w38
    tunnel: [w33] -> w18 mode=concatenating if=w32
    tunnel: [w31] -> w15 mode=indexing if=w29
    n2 = Unbundle By Name(w48) -> ("VariableType"=w37:string, "ROIArray"=w40:T17, "PointArray"=w47:cluster{"X":sgl, "Y":sgl}[], "Line Array"=w36:T18, "CircleArrayOUT"=w46:T19, "Value"=w34:sgl[], "Co-sys Reference"=w30:T20)
    n3 = case shown="\"3DPoint\", \"Point\"" w37 {
      tunnel: w47 -> [w54 w56 w78 w82 w99 w108 w118]
      tunnel: w36 -> [w53 w67 w70 w86 w98 w107 w117]
      tunnel: w46 -> [w52 w66 w72 w85 w97 w106 w116]
      tunnel: [w54 w56 w78 w82 w99 w108 w118] -> w45
      tunnel: [w53 w67 w70 w86 w98 w107 w117] -> w44
      tunnel: [w52 w66 w72 w85 w97 w106 w116] -> w35
      tunnel: [w49 TRUE TRUE FALSE w90 FALSE w112] -> w43
      tunnel: [w49 FALSE FALSE TRUE FALSE FALSE w112] -> w42
      tunnel: [w49 TRUE TRUE FALSE FALSE FALSE w112] -> w41
      tunnel: [w51 w60 w71 w81 w93 w103 w115] -> w33
      tunnel: w40 -> [w55 w61 w73 w83 w96 w105 w119]
      tunnel: [w55 w61 w73 w83 w96 w105 w119] -> w39
      tunnel: [w49 FALSE FALSE FALSE FALSE TRUE w112] -> w38
      tunnel: w34 -> [w51 w60 w71 w81 w93 w103 w115]
      tunnel: [w49 TRUE w68 w79 TRUE w101 w112] -> w32
      tunnel: [w50 w58 w69 w80 w91 w102 w114] -> w31
      tunnel: w30 -> [w50 w58 w69 w80 w91 w102 w114]
      tunnel: [w49 FALSE w68 w79 w90 w101 TRUE] -> w29
      frame Default {
        w49 = FALSE
      }
      frame "3DPoint", "Point" {
      }
      frame "Circle" {
        w68 = FALSE
      }
      frame "Line" {
        w79 = FALSE
      }
      frame "Angle", "Constant", "Depth", "Value", "Values" {
        w90 = FALSE
      }
      frame "ROI" {
        w101 = FALSE
      }
      frame "Reference" {
        w112 = FALSE
      }
    }
  }
  n4 = Unbundle By Name("Algo In") -> ("Measurement Name"=w13:string, "Pattern Match Base Reference"=w12:T21, "Measurement Type"=w8:string, "Measurement ROI.Measurement ROI array"=w11:T4[], "Selected Part"=w9:string, "Measurement Category"=w7:string, "Calibrated Image"=w10:T3, "Measurement Overlay Enabled"=w6:bool, "Conversion Factor"=w5:dbl, "Conversion Factor Enable"=w4:bool, "CurrentImageBounds"=w3:cluster{"Width":i32, "Height":i32}, "TPNominalDistanceData"=w2:T22)
  n5 = Index Array(array=w11) -> (element=w25:T4)  [unwired: 1 in]
  n6 = case shown="No Error" "error in (no error)" {
    selector: "error in (no error)" -> [w144 w3440]
    tunnel: w8 -> [w145 _]
    tunnel: [w124 w3440] -> w27
    tunnel: w20 -> [w143 _]
    tunnel: w21 -> [w142 _]
    tunnel: w19 -> [w141 _]
    tunnel: w18 -> [w140 _]
    tunnel: [w139 _] -> w26
    tunnel: w17 -> [w137 w3439]
    tunnel: w13 -> [w138 _]
    tunnel: [w136 w3439] -> w16
    tunnel: w25 -> [w135 _]
    tunnel: w10 -> [w134 _]
    tunnel: "Captured Image Array In" -> [w133 w3437]
    tunnel: w12 -> [w132 _]
    tunnel: w6 -> [w131 _]
    tunnel: w22 -> [w130 _]
    tunnel: w4 -> [w129 _]
    tunnel: w5 -> [w128 _]
    tunnel: w7 -> [w127 _]
    tunnel: w9 -> [w126 _]
    tunnel: w15 -> [w125 _]
    tunnel: w3 -> [w122 _]
    tunnel: w2 -> [w121 _]
    tunnel: "Measurement value" -> [w120 _]
    frame No Error {
      n7 = case shown="\"findCoorSys\"" w145 {
        selector: w145 -> [_ _ _ _ _ _ _ _ _ _ _ _ _ _ _ _ _ _ _ _ _ _ _ _ _ _ _ _ _ _ _ _ _ _ _ w1301 w1378 _ _ _ _ _ _ _ _ _ _ _ _ _ _ _ _ _ _ _ _ _ _ _ _ _ _ _ _ _ _ _ _ _ _ _ _ _ _ _ _ _ _ _ _ _ _ _ _ _ _ _ _ _]
        tunnel: w144 -> [w149 w151 w172 w216 w223 w250 w274 w313 w361 w404 w441 w493 w534 w570 w603 w620 w648 w667 w685 w711 w748 w785 w835 w867 w906 w951 w988 w1026 w1059 w1105 w1146 w1181 w1185 w1226 w1269 w1337 w1374 w1419 w1448 w1486 w1530 w1538 w1582 w1611 w1646 w1674 w1759 w1859 w1963 w2050 w2083 w2225 w2316 w2378 w2406 w2428 w2440 w2462 w2487 w2517 w2551 w2613 w2635 w2670 w2720 w2735 w2744 w2757 w2771 w2808 w2846 w2882 w2939 w2942 w2957 w2977 w3000 w3012 w3026 w3035 w3042 w3051 w3121 w3156 w3210 w3265 w3307 w3377 w3422 w3435]
        tunnel: [w149 w151 w179 w216 w227 w250 w269 w309 w356 w393 w437 w484 w510 w542 w578 w625 w645 w666 w692 w711 w721 w766 w827 w861 w898 w942 w967 w998 w1039 w1074 w1131 w1163 w1185 w1186 w1265 w1322 w1373 w1413 w1444 w1479 w1515 w1539 w1581 w1608 w1646 w1651 w1785 w1851 w1953 w2038 w2117 w2199 w2290 w2365 w2405 w2427 w2437 w2462 w2473 w2517 w2544 w2604 w2635 w2663 w2711 w2735 w2746 w2755 w2775 w2810 w2849 w2887 w2923 w2942 w2960 w2976 w2994 w3002 w3026 w3035 w3042 w3071 w3120 w3157 w3211 w3264 w3309 w3355 w3422 w3434] -> w123
        tunnel: w143 -> [_ _ w169 _ _ _ _ _ _ _ w447 _ w524 w559 _ _ _ _ _ _ _ _ w819 w852 _ w926 _ w1011 w1047 _ _ w1180 _ _ _ _ _ _ _ _ _ _ w1586 _ _ _ _ w1841 w1936 w2020 _ w2206 w2297 _ _ _ _ _ _ _ w2539 _ _ _ _ _ w2736 _ _ _ _ _ _ _ _ _ _ _ _ _ _ _ w3114 w3139 _ w3257 w3306 _ _ _]
        tunnel: w142 -> [_ _ w168 _ w224 _ _ _ _ _ _ w475 _ _ _ _ _ _ _ _ _ _ _ w866 w885 w927 _ _ w1048 w1092 w1144 _ _ _ _ w1300 _ _ _ _ w1513 _ _ _ _ w1659 w1774 _ _ w2025 _ w2205 w2296 _ _ _ _ _ _ _ _ w2601 _ _ _ _ _ _ _ _ _ _ _ _ w2950 w2983 w3001 w3006 _ _ _ _ _ _ _ _ _ _ _ w3436]
        tunnel: w141 -> [_ _ _ _ _ _ _ _ _ _ _ _ w523 _ w593 _ _ _ _ _ _ _ _ _ _ _ w977 _ _ w1091 _ _ _ _ _ w1299 w1385 _ _ w1469 _ w1553 _ w1630 _ _ w1773 _ w1935 _ w2106 w2197 w2288 w2377 _ _ w2449 _ _ _ _ _ _ w2653 w2694 _ _ w2758 _ _ _ _ _ _ _ _ _ _ _ _ _ w3061 _ _ w3181 _ _ w3366 _ _]
        tunnel: w140 -> [_ _ _ _ _ _ _ _ _ _ _ w472 _ _ _ _ _ _ _ _ _ _ _ w855 _ _ _ _ w1038 _ w1143 w1162 _ _ _ _ _ _ _ _ w1506 w1535 _ w1605 _ _ w1757 _ w1925 _ w2091 w2196 w2286 _ _ _ _ _ _ _ w2526 w2576 _ _ _ _ _ _ _ _ _ _ _ _ _ w2986 w2992 w3016 w3025 w3034 _ _ _ _ _ _ _ _ _ _]
        tunnel: [_ _ w181 _ w230 _ w279 w315 w364 w398 w455 w491 w531 w567 w600 w633 w656 w674 w698 _ w754 w786 w832 w853 w903 w947 w985 w1023 w1063 w1102 w1129 w1165 _ w1234 w1257 w1336 w1394 w1424 w1454 w1492 w1516 w1568 w1596 w1637 _ w1673 w1782 w1856 w1960 w2047 w2121 w2218 w2309 w2359 w2407 w2429 w2455 _ w2490 _ w2548 w2610 _ w2667 w2717 _ w2751 w2763 w2794 w2832 w2870 w2908 w2918 _ w2966 w2988 w2995 w3008 w3028 w3037 _ w3066 w3115 w3160 w3203 w3259 w3311 w3339 _ w3423] -> w139
        tunnel: w138 -> [_ _ w161 _ w229 _ w273 w312 w360 w390 w451 w478 w528 w561 w594 w617 w651 w669 w693 _ w738 w770 w831 w862 w902 w946 w978 w1013 w1050 w1097 w1127 w1166 _ w1203 w1273 w1313 w1362 w1407 w1436 w1489 w1503 w1564 w1592 w1633 _ w1661 w1767 w1844 w1945 w2030 w2109 w2216 w2307 w2369 w2409 w2431 w2457 _ w2492 _ w2546 w2608 _ w2659 w2703 _ w2752 w2764 w2795 w2833 w2871 w2909 w2919 _ w2964 w2989 w2993 w3004 w3027 w3036 _ w3052 w3098 w3140 w3184 w3244 w3293 w3336 _ w3425]
        tunnel: w137 -> [w148 w150 w159 w215 w228 w251 w260 w304 w350 w387 w449 w479 w530 w565 w598 w632 w655 w673 w697 w712 w740 w780 w821 w860 w891 w936 w983 w1020 w1057 w1101 w1133 w1169 w1184 w1217 w1259 w1326 w1389 w1406 w1438 w1477 w1531 w1567 w1595 w1636 w1647 w1667 w1778 w1845 w1946 w2031 w2111 w2217 w2308 w2371 w2410 w2432 w2458 w2463 w2479 w2518 w2542 w2602 w2634 w2654 w2697 w2734 w2750 w2762 w2793 w2831 w2869 w2907 w2917 w2941 w2943 w2987 w2996 w3007 w3029 w3038 w3041 w3057 w3100 w3144 w3183 w3243 w3292 w3381 w3421 w3430]
        tunnel: [w148 w150 w158 w215 w228 w251 w259 w303 w349 w386 w450 w480 w529 w564 w597 w629 w652 w670 w694 w712 w739 w779 w820 w860 w892 w935 w982 w1019 w1056 w1099 w1130 w1164 w1184 w1218 w1258 w1327 w1390 w1406 w1437 w1476 w1532 w1565 w1593 w1634 w1647 w1666 w1777 w1846 w1947 w2032 w2110 w2213 w2304 w2360 w2408 w2430 w2456 w2463 w2480 w2518 w2543 w2603 w2634 w2655 w2698 w2734 w2750 w2762 w2793 w2831 w2869 w2907 w2917 w2941 w2944 w2987 w2996 w3007 w3029 w3038 w3041 w3056 w3099 w3143 w3182 w3242 w3291 w3370 w3421 w3424] -> w136
        tunnel: w135 -> [_ _ _ _ _ _ w277 w314 w363 w405 _ _ _ _ _ w638 w661 w679 w703 _ w744 w781 _ _ _ _ _ _ _ _ _ _ _ w1230 w1270 _ _ w1417 w1449 _ _ w1572 w1600 w1641 _ _ _ _ _ _ _ _ _ _ w2401 w2423 w2452 _ w2489 _ _ _ _ _ _ _ _ _ w2765 w2826 w2864 w2902 w2940 _ w2959 _ _ _ _ _ _ _ _ _ _ _ _ _ _ _]
        tunnel: w134 -> [_ _ _ _ w221 _ _ _ _ _ _ _ _ _ _ _ _ _ w688 _ _ _ _ _ _ _ _ _ _ _ _ _ _ _ _ _ w1388 _ _ _ _ w1555 _ _ _ w1671 w1789 w1855 w1957 w2042 w2120 w2221 w2312 _ _ _ w2442 _ w2478 _ _ _ _ w2664 w2712 _ _ _ _ _ _ _ _ _ _ _ _ _ _ _ _ w3070 w3109 w3159 w3209 w3263 w3308 w3367 _ _]
        tunnel: w133 -> [_ _ w176 _ w225 _ w271 w310 w358 w396 _ w486 _ _ _ w637 w660 w678 w702 _ w746 w783 w829 _ w900 w944 _ _ _ _ _ _ _ w1223 w1271 w1334 _ w1422 w1452 w1487 _ w1571 w1599 w1640 _ _ w1787 w1852 w1955 w2040 w2118 _ _ _ w2404 w2426 w2454 _ w2495 _ _ w2606 _ _ _ _ _ _ w2791 w2829 w2867 w2905 w2937 _ w2961 _ _ _ _ _ _ _ w3111 w3142 w3208 w3254 w3303 _ _ _]
        tunnel: w132 -> [_ _ w155 _ _ _ _ _ _ _ _ _ _ _ _ _ _ _ _ _ _ _ _ _ _ _ _ _ _ _ _ _ _ _ _ _ _ _ _ _ _ _ _ _ _ _ _ _ _ _ _ _ _ _ _ _ _ _ _ _ _ _ _ _ _ _ _ _ _ _ _ _ _ _ _ _ _ _ _ _ _ _ _ _ _ _ _ w3376 _ _]
        tunnel: w131 -> [_ _ w154 _ w219 _ w267 w307 w354 w388 _ w483 _ _ _ w615 _ _ w680 _ w725 w768 w826 _ w897 w939 _ _ _ _ _ _ _ w1205 w1261 w1330 _ _ _ w1483 _ w1562 w1590 w1631 _ _ w1784 w1854 w1951 w2014 w2116 _ _ _ _ _ _ _ _ _ _ _ _ _ _ _ _ _ _ _ _ _ _ _ w2963 _ _ _ _ _ _ _ _ _ _ _ _ _ _ _]
        tunnel: w130 -> [_ _ _ _ _ _ _ _ _ w395 _ _ _ _ _ _ _ _ _ _ _ _ _ _ _ _ _ _ _ _ _ _ _ _ _ _ _ _ _ _ _ _ _ _ _ _ _ _ _ _ _ _ _ _ _ _ _ _ _ _ _ _ _ _ _ _ _ _ _ _ _ _ _ _ _ _ _ _ _ _ _ _ _ _ _ _ _ _ _ _]
        tunnel: w129 -> [_ _ _ _ w218 _ _ _ _ _ _ _ _ _ _ _ _ _ w686 _ _ _ _ _ _ _ _ _ _ _ _ _ _ _ _ _ w1380 _ _ _ _ w1556 _ _ _ w1669 w1780 w1848 w1948 w2034 w2113 w2223 w2287 _ _ _ w2436 _ _ _ _ _ _ w2657 w2700 _ _ _ _ _ _ _ _ _ _ _ _ _ _ _ _ w3062 w3108 w3151 w3197 w3252 w3300 w3368 _ _]
        tunnel: w128 -> [_ _ _ _ w217 _ _ _ _ _ _ _ _ _ _ _ w647 _ w687 _ _ _ _ _ _ _ _ _ _ _ _ w1176 _ _ _ _ w1381 _ _ _ w1529 w1557 _ w1612 _ w1668 w1779 w1847 w1949 w2033 w2112 w2222 w2313 w2361 w2397 w2414 w2441 _ _ _ _ _ _ w2656 w2699 _ _ _ _ _ _ _ _ _ _ _ _ _ _ _ _ w3063 w3107 w3152 w3196 w3251 w3301 w3375 _ _]
        tunnel: w127 -> [_ _ _ _ _ _ _ _ _ _ _ _ _ _ _ _ _ _ _ _ _ _ _ _ _ _ _ _ _ _ _ _ _ _ _ _ _ _ _ _ _ _ _ _ _ w1665 _ _ _ _ _ _ _ _ _ _ _ _ _ _ _ _ _ _ _ _ _ _ _ _ _ _ _ _ _ _ _ _ _ _ _ _ _ _ _ _ _ _ _ _]
        tunnel: w126 -> [_ _ _ _ _ _ _ _ _ _ _ _ _ _ _ _ _ _ _ _ _ _ _ _ _ _ _ _ _ _ _ _ _ _ _ _ _ _ _ _ _ _ _ _ _ _ _ _ _ _ _ _ _ _ _ _ _ _ _ _ _ _ _ _ _ _ _ _ _ _ _ _ _ _ _ _ _ _ _ _ _ _ _ _ _ _ _ _ _ _]
        tunnel: w125 -> [_ _ _ _ _ _ _ _ w337 _ _ _ _ _ _ _ _ _ _ _ _ _ _ _ _ _ _ _ _ _ _ _ _ _ _ _ _ _ _ _ _ _ _ _ _ _ _ _ _ _ _ _ _ _ _ _ _ _ _ _ _ _ _ _ _ _ _ _ _ _ _ _ _ _ _ _ _ _ _ _ _ _ _ _ _ _ _ _ _ _]
        tunnel: w122 -> [_ _ _ _ _ _ _ _ _ _ _ _ _ _ _ _ _ _ _ _ _ _ _ _ _ _ _ _ _ _ _ w1175 _ _ _ _ _ _ _ _ w1527 _ _ _ _ _ _ _ _ _ _ _ _ _ _ _ _ _ _ _ _ _ _ _ _ _ _ _ _ _ _ _ _ _ _ _ _ _ _ _ _ _ _ _ _ _ _ _ _ _]
        tunnel: w121 -> [_ _ _ _ _ _ _ _ _ _ _ _ _ _ _ _ _ _ _ _ _ _ _ _ _ _ _ _ _ _ _ _ _ _ _ _ _ _ _ _ _ _ _ _ _ _ _ _ _ _ _ _ _ _ _ _ _ _ _ _ _ _ _ _ _ _ _ _ _ _ _ _ _ _ _ _ _ _ _ _ _ _ _ _ _ _ _ w3380 _ _]
        tunnel: w120 -> [_ _ _ _ _ _ _ _ _ _ _ _ _ _ _ _ _ _ _ _ _ _ _ _ _ _ _ _ _ _ _ _ _ _ _ _ _ _ _ _ _ _ _ _ _ _ _ _ _ _ _ _ _ _ _ _ _ _ _ _ _ _ _ _ _ _ _ _ _ _ _ _ _ _ _ _ _ _ _ _ _ _ _ _ _ _ _ w3327 _ _]
        frame Default {
        }
        frame "----coordinate system----" {
        }
        frame "findCoorSys" {
          w165 = 1
          w182 = T14 {"VariableName"="", "VariableType"="", "Co-sys Reference"={"Base Co-sys Reference"={"Origin"={"X"=0.0, "Y"=0.0}, "Angle (deg)"=0.0, "Axis Reference"=0, "Scale"=0.0}, "New Co-sys Reference"={"Origin"={"X"=0.0, "Y"=0.0}, "Angle (deg)"=0.0, "Axis Reference"=0, "Scale"=0.0}}, "PointArray"=[], "Line Array"=[], "CircleArrayOUT"=[], "TPDetails"={"DistanceInfo"={"X"=0.0, "Y"=0.0, "X'"=0.0, "Y'"=0.0, "DX"=0.0, "DY"=0.0, "Distance Type"=""}, "Feature and Datum details"=[]}, "Value"=[], "Display Name"=0.0, "ROIArray"=[], "Update ROI "=FALSE}  # AlgoOut
          # "According to the decription in the help provided in the find coordinate syatem VI, the coordinate system is found by 3 points\nThe first two points to be along x axis\nAnd the third point along y axis\nThe logic below is to decide the order of the first two points, the logic to select frist and second point\nHere we have two lines(X and Y) and one point(intersection point)\nline 1 is lineX and line2 is line Y.\nSo there are three points(two of line 1 and one is the input point) out of which we need to select two points.\nSo, select two out of three and decide their order.\nSo, the two points are - Point from line whose X coordinate is higher\n                                       - The provided input point\nNow we need to decide the order of both\nPoint 1 is the point out if the two whose X is smaller\nPoint 2 is the point out of the two whose X is higher\nPoint 3 is finally the point (any out of 2) on Y axis"
          # "the VI accepts the input coordinate in I 32 and outputs it as SGL. \nHence returns the output coordinate as SGL and loosing the post decimal information\nHence tried with this VI so that the output edge inormation is not lost\nBut found that the repeatability was lost   q"
          n8 = Index Array(array=w176) -> (element=w177:T42)  [unwired: 1 in]
          n9 = Index Array(array=w168) -> (element=w170:cluster{"X":sgl, "Y":sgl})  [unwired: 1 in]
          n10 = Index Array(array=w169) -> (element=w174:T23)  [unwired: 1 in]
          n11 = Unbundle By Name(w177) -> ("Captured Image"=w175:T3)
          n12 = Array Size(array=w168) -> (size(s)=w167:i32)
          n13 = Array Size(array=w169) -> (size(s)=w166:i32)
          n14 = Equal?(x=w166, y=w165) -> (x = y?=w164:bool)
          n15 = Equal?(x=w167, y=w165) -> (x = y?=w163:bool)
          n16 = And(x=w164, y=w163) -> (x .and. y?=w162:bool)
          n17 = case shown="True" w162 {
            tunnel: [w185 w205] -> w180
            tunnel: w174 -> [_ w204]
            tunnel: w172 -> [w185 w202]
            tunnel: w170 -> [_ w201]
            tunnel: w155 -> [_ w198]
            tunnel: [w184 w190] -> w160
            tunnel: [w184 w197] -> w153
            tunnel: [w183 w186] -> w152
            frame False {
              w183 = T43 {"Origin"={"X"=nan, "Y"=nan}, "Angle (deg)"=nan, "Axis Reference"=0}  # PointForOverlays.Coordinate System
              w184 = T44 {"Origin"={"X"=nan, "Y"=nan}, "Angle (deg)"=nan, "Axis Reference"=0, "Angle (deg) 2"=nan} ("Coordinate System")
            }
            frame True {
              w191 = T43 {"Origin"={"X"=0.0, "Y"=0.0}, "Angle (deg)"=0.0, "Axis Reference"=0}  # PointForOverlays.Coordinate System
              w196 = T45 {"Origin"={"X"=0.0, "Y"=0.0}, "Angle (deg)"=0.0, "Axis Reference"=0, "Scale"=1.0}  # New Reference IN
              w206 = u32 0 items=["Direct", "Indirect"] ("Axis Reference")
              # "point on y axis"
              # "along x axis"
              n18 = Unbundle By Name(w204) -> ("Line.Point 1"=w200:cluster{"X":sgl, "Y":sgl}, "Line.Point 2"=w199:cluster{"X":sgl, "Y":sgl})
              n19 = Build Array(w200, w199, w201) -> (w203:cluster{"X":sgl, "Y":sgl}[])
              n20 = call "IMAQ Build CoordSys (Points)"("Reference Points"=w203, "Axis Reference"=w206, "error in (no error)"=w202) -> ("Coordinate System"=w195:T43, "error out"=w205:errorcluster)  [unwired: 2 in]
              n21 = Unbundle By Name(w195) -> ("Origin"=w193:cluster{"X":sgl, "Y":sgl}, "Angle (deg)"=w192:sgl)
              n22 = Bundle By Name(cluster=w196, "Origin"=w193, "Angle (deg)"=w192) -> (w194:T45)
              n23 = call "Reference Checking for NaN.vi"("New Reference IN"=w194, "Base Reference IN"=w198) -> ("New Reference Out"=w190:T45, "Base Reference Out"=w197:T45)  [unwired: 7 in, 1 out]
              n24 = Unbundle By Name(w190) -> ("Origin"=w189:cluster{"X":sgl, "Y":sgl}, "Angle (deg)"=w188:sgl, "Axis Reference"=w187:u32)
              n25 = Bundle By Name(cluster=w191, "Origin"=w189, "Angle (deg)"=w188, "Axis Reference"=w187) -> (w186:T43)
            }
          }
          n26 = Bundle By Name(cluster=w182, "VariableName"=w161, "Co-sys Reference.Base Co-sys Reference"=w153, "VariableType"="Reference", "Co-sys Reference.New Co-sys Reference"=w160) -> (w181:T14)
          n27 = Bundle By Name(cluster=w159, "Measurment Name"=w161, "Measurment Type"="Coordinate system", "PointForOverlays.Coordinate System"=w152, "Color"=u32 1216511) -> (w158:T12)
          n28 = Unbundle By Name(w160) -> ("Origin"=w173:cluster{"X":sgl, "Y":sgl})
          n29 = Build Array(w173) -> (w178:cluster{"X":sgl, "Y":sgl}[])
          n30 = case shown="True" w154 {
            tunnel: w180 -> [w208 w214]
            tunnel: [w208 w213] -> w179
            tunnel: w178 -> [_ w212]
            tunnel: [w207 w211] -> _
            tunnel: w175 -> [w207 w209]
            frame False {
              # "Measurement overlay disabled"
            }
            frame True {
              # "overlay the orgin point"
              n31 = call "Overlay Points with User Specified Size.vi"("error in"=w214, "Point Diameter (5)"=u32 10, "Points"=w212, "Image In"=w209) -> ("error out"=w213:errorcluster, "Image Out"=w211:T3)  [unwired: 6 in]
            }
          }
        }
        frame "----calibration----" {
        }
        frame "CalibPoints" {
          w232 = T14 {"VariableName"="", "VariableType"="", "Co-sys Reference"={"Base Co-sys Reference"={"Origin"={"X"=0.0, "Y"=0.0}, "Angle (deg)"=0.0, "Axis Reference"=0, "Scale"=0.0}, "New Co-sys Reference"={"Origin"={"X"=0.0, "Y"=0.0}, "Angle (deg)"=0.0, "Axis Reference"=0, "Scale"=0.0}}, "PointArray"=[], "Line Array"=[], "CircleArrayOUT"=[], "TPDetails"={"DistanceInfo"={"X"=0.0, "Y"=0.0, "X'"=0.0, "Y'"=0.0, "DX"=0.0, "DY"=0.0, "Distance Type"=""}, "Feature and Datum details"=[]}, "Value"=[], "Display Name"=0.0, "ROIArray"=[], "Update ROI "=FALSE}  # AlgoOut
          n32 = Index Array(array=w225) -> (element=w226:T42)  [unwired: 1 in]
          n33 = Unbundle By Name(w226) -> ("Captured Image"=w220:T3)
          n34 = case shown="True" w219 {
            tunnel: w224 -> [_ w249]
            tunnel: w223 -> [w243 w248]
            tunnel: [w243 w247] -> w222
            tunnel: w220 -> [_ w244]
            frame False {
            }
            frame True {
              w245 = u32 10  # Point Diameter
              w246 = u32 6618880  # Color
              n35 = call "Overlay Points with User Specified Size.vi"("Color"=w246, "error in"=w248, "Point Diameter (5)"=w245, "Points"=w249, "Image In"=w244) -> ("error out"=w247:errorcluster)  [unwired: 5 in, 1 out]
            }
          }
          n36 = case shown="False" w218 {
            tunnel: [w238 w240] -> w231
            tunnel: [w237 w239] -> w227
            tunnel: w224 -> [w236 w242]
            tunnel: w222 -> [w235 w239]
            tunnel: w221 -> [w234 _]
            tunnel: w217 -> [_ w241]
            frame False {
              n37 = call "IMAQ Convert Pixel to Real World"("error in (no error)"=w235, "Array of Pixel Coordinates"=w236, "Calibrated Image"=w234) -> ("error out"=w237:errorcluster, "Array of Real World Coordinates"=w238:cluster{"X":sgl, "Y":sgl}[])  [unwired: 3 in, 4 out]
            }
            frame True {
              n38 = Divide(x=w242, y=w241) -> (x/y=w240:cluster{"X":dbl, "Y":dbl}[])
            }
          }
          n39 = Bundle By Name(cluster=w232, "VariableName"=w229, "VariableType"="Point", "PointArray"=w231) -> (w230:T14)
        }
        frame "----point detection method----" {
        }
        frame "pointDirect" {
          w278 = T46 {"Edge Options"={"Edge Polarity"=0, "Kernel Size"=3, "Width"=3, "Minimum Edge Strength"=10.0, "Interpolation Type"=enum."Bilinear Fixed", "Data Processing Method"=enum."Average"}, "Process"=enum."Get All Edges"}  # pointSettings
          w281 = T14 {"VariableName"="", "VariableType"="", "Co-sys Reference"={"Base Co-sys Reference"={"Origin"={"X"=0.0, "Y"=0.0}, "Angle (deg)"=0.0, "Axis Reference"=0, "Scale"=0.0}, "New Co-sys Reference"={"Origin"={"X"=0.0, "Y"=0.0}, "Angle (deg)"=0.0, "Axis Reference"=0, "Scale"=0.0}}, "PointArray"=[], "Line Array"=[], "CircleArrayOUT"=[], "TPDetails"={"DistanceInfo"={"X"=0.0, "Y"=0.0, "X'"=0.0, "Y'"=0.0, "DX"=0.0, "DY"=0.0, "Distance Type"=""}, "Feature and Datum details"=[]}, "Value"=[], "Display Name"=0.0, "ROIArray"=[], "Update ROI "=FALSE}  # AlgoOut
          # "MEASUREMENT TYPE"
          n40 = Index Array(array=w271) -> (element=w272:T42)  [unwired: 1 in]
          n41 = Unbundle By Name(w277) -> ("Edge threshold"=w265:dbl, "Edge Options"=w266:T5, "ROI Overlay Enabled"=w263:bool, "ROI"=w261:T47)
          n42 = Unbundle By Name(w272) -> ("Captured Image"=w270:T3)
          n43 = Bundle By Name(cluster=w278, "Edge Options.Minimum Edge Strength"=w265, "Edge Options"=w266) -> (w262:T46)
          n44 = case shown="True" w263 {
            tunnel: w274 -> [w287 w290]
            tunnel: [w287 w293] -> w276
            tunnel: w270 -> [w288 w292]
            tunnel: [w288 w289] -> w275
            tunnel: w261 -> [_ w291]
            frame False {
              # "ROI OVERLAY DISABLED"
            }
            frame True {
              # "ROI OVERLAY ENABLED"
              n45 = call "IMAQ Overlay ROI"("error in (no error)"=w290, "ROI Descriptor"=w291, "Image"=w292) -> ("error out"=w293:errorcluster, "Image Out"=w289:T3)  [unwired: 7 in]
            }
          }
          n46 = call "pointDetectDirect.vi"("error in (no error)"=w276, "ROI Descriptor"=w261, "pointSettings"=w262, "Image"=w275) -> ("error out"=w254:errorcluster, "Location (Pixel)"=w257:cluster{"X":sgl, "Y":sgl}, "Image Out"=w258:T3)  [unwired: 5 in]
          n47 = call "point_within_img.vi"("error in (no error)"=w254, "Image"=w258, "Point"=w257) -> ("error out"=w253:errorcluster, "Point"=w255:cluster{"Point X":dbl, "Point Y":dbl})  [unwired: 6 in, 1 out]
          n48 = call "FEATURE_DETECTED.vi"("error in (no error)"=w253, "Point"=w255) -> ("error out"=w252:errorcluster, "s? t:f"=w256:cluster{"X":dbl, "Y":dbl})  [unwired: 7 in, 1 out]
          n49 = Build Array(w256) -> (w264:cluster{"X":dbl, "Y":dbl}[])
          n50 = case shown="True" w267 {
            tunnel: w258 -> [_ w284]
            tunnel: w252 -> [w282 w285]
            tunnel: [w282 w286] -> w269
            tunnel: w256 -> [_ w283]
            frame False {
              # "MEASUREMENT IS DISABLED"
            }
            frame True {
              # "MEASUREMENT IS ENABLED"
              n51 = call "IMAQ Overlay Points"("error in (no error)"=w285, "Point"=w283, "Image"=w284) -> ("error out"=w286:errorcluster)  [unwired: 7 in, 1 out]
            }
          }
          n52 = Bundle By Name(cluster=w260, "Measurment Type"="point", "Measurment Name"=w273, "PointForOverlays.Points.Points"=w264) -> (w259:T12)
          n53 = Bundle By Name(cluster=w281, "VariableName"=w273, "VariableType"="Point", "PointArray"=w264) -> (w279:T14)
        }
        frame "3DPointDetect" {
          w317 = T14 {"VariableName"="", "VariableType"="", "Co-sys Reference"={"Base Co-sys Reference"={"Origin"={"X"=0.0, "Y"=0.0}, "Angle (deg)"=0.0, "Axis Reference"=0, "Scale"=0.0}, "New Co-sys Reference"={"Origin"={"X"=0.0, "Y"=0.0}, "Angle (deg)"=0.0, "Axis Reference"=0, "Scale"=0.0}}, "PointArray"=[], "Line Array"=[], "CircleArrayOUT"=[], "TPDetails"={"DistanceInfo"={"X"=0.0, "Y"=0.0, "X'"=0.0, "Y'"=0.0, "DX"=0.0, "DY"=0.0, "Distance Type"=""}, "Feature and Datum details"=[]}, "Value"=[], "Display Name"=0.0, "ROIArray"=[], "Update ROI "=FALSE}  # AlgoOut
          # "MEASUREMENT TYPE"
          n54 = Index Array(array=w310) -> (element=w311:T42)  [unwired: 1 in]
          n55 = Unbundle By Name(w314) -> ("ROI Overlay Enabled"=w305:bool, "ROI"=w298:T47)
          n56 = Unbundle By Name(w311) -> ("Captured Image"=w295:T3)
          n57 = case shown="True" w305 {
            tunnel: w313 -> [w323 w326]
            tunnel: [w323 w329] -> w297
            tunnel: w295 -> [w324 w328]
            tunnel: [w324 w325] -> w299
            tunnel: w298 -> [_ w327]
            frame False {
              # "ROI OVERLAY DISABLED"
            }
            frame True {
              # "ROI OVERLAY ENABLED"
              n58 = call "IMAQ Overlay ROI"("error in (no error)"=w326, "ROI Descriptor"=w327, "Image"=w328) -> ("error out"=w329:errorcluster, "Image Out"=w325:T3)  [unwired: 7 in]
            }
          }
          n59 = call "Laser Point.vi"("error in (no error)"=w297, "ROI Descriptor"=w298, "Image Out"=w299) -> ("error out"=w296:errorcluster, "point"=w294:cluster{"x":dbl, "y":dbl})  [unwired: 6 in, 1 out]
          n60 = call "point_within_img.vi"("error in (no error)"=w296, "Image"=w295, "Point"=w294) -> ("error out"=w301:errorcluster, "Point"=w302:cluster{"Point X":dbl, "Point Y":dbl})  [unwired: 6 in, 1 out]
          n61 = call "FEATURE_DETECTED.vi"("error in (no error)"=w301, "Point"=w302) -> ("error out"=w300:errorcluster)  [unwired: 7 in, 2 out]
          n62 = Build Array(w294) -> (w306:cluster{"x":dbl, "y":dbl}[])
          n63 = case shown="True" w307 {
            tunnel: w295 -> [_ w320]
            tunnel: w300 -> [w318 w321]
            tunnel: [w318 w322] -> w309
            tunnel: w294 -> [_ w319]
            frame False {
              # "MEASUREMENT IS DISABLED"
            }
            frame True {
              # "MEASUREMENT IS ENABLED"
              n64 = call "IMAQ Overlay Points"("error in (no error)"=w321, "Point"=w319, "Image"=w320) -> ("error out"=w322:errorcluster)  [unwired: 7 in, 1 out]
            }
          }
          n65 = Bundle By Name(cluster=w304, "Measurment Type"="point", "Measurment Name"=w312, "PointForOverlays.Points.Points"=w306) -> (w303:T12)
          n66 = Bundle By Name(cluster=w317, "VariableName"=w312, "VariableType"="3DPoint", "PointArray"=w306) -> (w315:T14)
        }
        frame "ObjectCenter" {
          w366 = T14 {"VariableName"="", "VariableType"="", "Co-sys Reference"={"Base Co-sys Reference"={"Origin"={"X"=0.0, "Y"=0.0}, "Angle (deg)"=0.0, "Axis Reference"=0, "Scale"=0.0}, "New Co-sys Reference"={"Origin"={"X"=0.0, "Y"=0.0}, "Angle (deg)"=0.0, "Axis Reference"=0, "Scale"=0.0}}, "PointArray"=[], "Line Array"=[], "CircleArrayOUT"=[], "TPDetails"={"DistanceInfo"={"X"=0.0, "Y"=0.0, "X'"=0.0, "Y'"=0.0, "DX"=0.0, "DY"=0.0, "Distance Type"=""}, "Feature and Datum details"=[]}, "Value"=[], "Display Name"=0.0, "ROIArray"=[], "Update ROI "=FALSE}  # AlgoOut
          # "MEASUREMENT TYPE"
          n67 = Index Array(array=w358) -> (element=w359:T42)  [unwired: 1 in]
          n68 = Unbundle By Name(w363) -> ("ROI Overlay Enabled"=w352:bool, "ROI"=w351:T47)
          n69 = Unbundle By Name(w359) -> ("Captured Image"=w357:T3)
          n70 = Index Array(array=w337) -> (element=w336:T20)  [unwired: 1 in]
          n71 = Unbundle By Name(w336) -> ("New Co-sys Reference.Angle (deg)"=w335:sgl, "Base Co-sys Reference.Angle (deg)"=w334:sgl)
          n72 = Subtract(x=w335, y=w334) -> (x-y=w332:sgl)
          n73 = case shown="True" w352 {
            tunnel: w361 -> [w372 w375]
            tunnel: [w372 w378] -> w362
            tunnel: w357 -> [w373 w377]
            tunnel: [w373 w374] -> w343
            tunnel: w351 -> [_ w376]
            frame False {
              # "ROI OVERLAY DISABLED"
            }
            frame True {
              # "ROI OVERLAY ENABLED"
              n74 = call "IMAQ Overlay ROI"("error in (no error)"=w375, "ROI Descriptor"=w376, "Image"=w377) -> ("error out"=w378:errorcluster, "Image Out"=w374:T3)  [unwired: 7 in]
            }
          }
          n75 = call "ObjectCenter.vi"("error in (no error)"=w362, "ROI Descriptor"=w351, "Image in"=w343) -> ("error out"=w346:errorcluster, "Distance"=w341:dbl, "Centroid"=w342:cluster{"X Centroid":sgl, "Y Centroid":sgl})  [unwired: 6 in]
          n76 = call "point_within_img.vi"("error in (no error)"=w346, "Image"=w343, "Point"=w342) -> ("error out"=w345:errorcluster, "Point"=w347:cluster{"Point X":dbl, "Point Y":dbl})  [unwired: 6 in, 1 out]
          n77 = call "FEATURE_DETECTED.vi"("error in (no error)"=w345, "Point"=w347) -> ("error out"=w344:errorcluster, "s? t:f"=w348:cluster{"X":dbl, "Y":dbl}, "x .and. y?"=w331:bool)  [unwired: 7 in]
          n78 = Select(t=nan, s=w331, f=w332) -> (s? t:f=w330:dbl)
          n79 = Select(t=nan, s=w331, f=w341) -> (s? t:f=w339:dbl)
          n80 = Build Array(w348) -> (w353:cluster{"X":dbl, "Y":dbl}[])
          n81 = Build Array(w339, w330) -> (w338:dbl[])
          n82 = case shown="True" w354 {
            tunnel: w343 -> [_ w369]
            tunnel: w344 -> [w367 w370]
            tunnel: [w367 w371] -> w356
            tunnel: w348 -> [_ w368]
            frame False {
              # "MEASUREMENT IS DISABLED"
            }
            frame True {
              # "MEASUREMENT IS ENABLED"
              n83 = call "IMAQ Overlay Points"("error in (no error)"=w370, "Point"=w368, "Image"=w369) -> ("error out"=w371:errorcluster)  [unwired: 7 in, 1 out]
            }
          }
          n84 = Bundle By Name(cluster=w350, "Measurment Type"="point", "Measurment Name"=w360, "PointForOverlays.Points.Points"=w353) -> (w349:T12)
          n85 = Bundle By Name(cluster=w366, "VariableName"=w360, "VariableType"="Point", "PointArray"=w353, "Value"=w338) -> (w364:T14)
        }
        frame "detectAllEdgePoints" {
          w400 = T14 {"VariableName"="", "VariableType"="", "Co-sys Reference"={"Base Co-sys Reference"={"Origin"={"X"=0.0, "Y"=0.0}, "Angle (deg)"=0.0, "Axis Reference"=0, "Scale"=0.0}, "New Co-sys Reference"={"Origin"={"X"=0.0, "Y"=0.0}, "Angle (deg)"=0.0, "Axis Reference"=0, "Scale"=0.0}}, "PointArray"=[], "Line Array"=[], "CircleArrayOUT"=[], "TPDetails"={"DistanceInfo"={"X"=0.0, "Y"=0.0, "X'"=0.0, "Y'"=0.0, "DX"=0.0, "DY"=0.0, "Distance Type"=""}, "Feature and Datum details"=[]}, "Value"=[], "Display Name"=0.0, "ROIArray"=[], "Update ROI "=FALSE}  # AlgoOut
          # "measurement type"
          n86 = Index Array(array=w396) -> (element=w397:T42)  [unwired: 1 in]
          n87 = Unbundle By Name(w405) -> ("Edge Options"=w391:T5, "ROI Overlay Enabled"=w401:bool)
          n88 = Unbundle By Name(w397) -> ("Captured Image"=w385:T3)  [unwired: 1 out]
          n89 = Index Array(array=w395) -> (element=w392:T47)  [unwired: 1 in]
          n90 = case shown="True" w401 {
            tunnel: w404 -> [w420 w430]
            tunnel: [w420 w434] -> w403
            tunnel: w385 -> [w421 w433]
            tunnel: [w421 w432] -> w402
            tunnel: w392 -> [_ w431]
            frame False {
              # "ROI OVERLAY DISABLED"
            }
            frame True {
              w426 = cluster{"X":i32, "Y":i32} {"X"=0, "Y"=0}  # Start Point
              # "ROI OVELAY ENABLED"
              n91 = Unbundle By Name(w431) -> ("Global Rectangle"=w429:i32[])
              n92 = Index Array(array=w429) -> (element #1=w428:i32, element #2=w427:i32, element #3=w425:i32, element #4=w424:i32)  [unwired: 4 in]
              n93 = Bundle By Name(cluster=w426, "X"=w425, "Y"=w424) -> (w422:cluster{"X":i32, "Y":i32})
              n94 = Bundle By Name(cluster=w426, "X"=w428, "Y"=w427) -> (w423:cluster{"X":i32, "Y":i32})
              n95 = call "IMAQ Overlay Line"("error in (no error)"=w430, "End Point"=w422, "Start Point"=w423, "Image"=w433) -> ("error out"=w434:errorcluster, "Image Out"=w432:T3)  [unwired: 6 in]
            }
          }
          n96 = call "detectEdgePoints.vi"("error in (no error)"=w403, "ROI"=w392, "Edge Options"=w391, "Image"=w402) -> ("error out"=w381:errorcluster, "edgePoints"=w384:cluster{"X":sgl, "Y":sgl}[], "ImageOUT"=w394:T3)  [unwired: 4 in, 1 out]
          n97 = for {
            tunnel: [w412] -> w383 mode=indexing
            tunnel: w385 -> [w414]
            tunnel: w384 -> [w413] mode=indexing
            tunnel: w381 -> [w411]
            tunnel: [w410] -> w380
            n98 = call "point_within_img.vi"("error in (no error)"=w411, "Image"=w414, "Point"=w413) -> ("error out"=w410:errorcluster, "Point"=w412:cluster{"Point X":dbl, "Point Y":dbl})  [unwired: 6 in, 1 out]
          }
          n99 = for {
            tunnel: w383 -> [w409] mode=indexing
            tunnel: [w408] -> w382 mode=indexing
            tunnel: w380 -> [w407]
            tunnel: [w406] -> w379
            n100 = call "FEATURE_DETECTED.vi"("error in (no error)"=w407, "Point"=w409) -> ("error out"=w406:errorcluster, "s? t:f"=w408:cluster{"X":dbl, "Y":dbl})  [unwired: 7 in, 1 out]
          }
          n101 = case shown="True" w388 {
            tunnel: w394 -> [_ w419]
            tunnel: w379 -> [w415 w416]
            tunnel: [w415 w417] -> w393
            tunnel: w382 -> [_ w418]
            frame False {
              # "measurement overlay disabled"
            }
            frame True {
              # "measurement overlay enabled"
              n102 = call "IMAQ Overlay Points"("error in (no error)"=w416, "Array of Points"=w418, "Image"=w419) -> ("error out"=w417:errorcluster)  [unwired: 7 in, 1 out]
            }
          }
          n103 = Bundle By Name(cluster=w387, "Measurment Type"="point", "Measurment Name"=w390, "PointForOverlays.Points.Points"=w382) -> (w386:T12)
          n104 = Bundle By Name(cluster=w400, "VariableName"=w390, "VariableType"="Point", "PointArray"=w382) -> (w398:T14)
        }
        frame "midpointOfLine" {
          w457 = T14 {"VariableName"="", "VariableType"="", "Co-sys Reference"={"Base Co-sys Reference"={"Origin"={"X"=0.0, "Y"=0.0}, "Angle (deg)"=0.0, "Axis Reference"=0, "Scale"=0.0}, "New Co-sys Reference"={"Origin"={"X"=0.0, "Y"=0.0}, "Angle (deg)"=0.0, "Axis Reference"=0, "Scale"=0.0}}, "PointArray"=[], "Line Array"=[], "CircleArrayOUT"=[], "TPDetails"={"DistanceInfo"={"X"=0.0, "Y"=0.0, "X'"=0.0, "Y'"=0.0, "DX"=0.0, "DY"=0.0, "Distance Type"=""}, "Feature and Datum details"=[]}, "Value"=[], "Display Name"=0.0, "ROIArray"=[], "Update ROI "=FALSE}  # AlgoOut
          n105 = Index Array(array=w447) -> (element=w454:T23)  [unwired: 1 in]
          n106 = Array Size(array=w447) -> (size(s)=w446:i32)
          n107 = Unbundle By Name(w454) -> ("Line.Point 1"=w436:cluster{"X":sgl, "Y":sgl}, "Line.Point 2"=w435:cluster{"X":sgl, "Y":sgl})
          n108 = Equal?(x=w446, y=1) -> (x = y?=w443:bool)
          n109 = Equal?(x=w436, y=w435) -> (x = y?=w444:cluster{"X":bool, "Y":bool})
          n110 = Unbundle By Name(w444) -> ("X"=w440:bool, "Y"=w439:bool)
          n111 = Not And(1:w439, 2:w440) -> (0:w438:bool)
          n112 = Or(x=w438, y=w443) -> (x .or. y?=w442:bool)
          n113 = case shown="True" w442 {
            tunnel: w441 -> [w459 w464]
            tunnel: [cluster{"X":sgl, "Y":sgl} {"X"=nan, "Y"=nan} ("midpoint") w463] -> w448
            tunnel: [w459 w462] -> w437
            tunnel: w436 -> [_ w461]
            tunnel: w435 -> [_ w460]
            frame False {
            }
            frame True {
              n114 = call "midpointOfLine.vi"("error in (no error)"=w464, "Point2 (Pixels)"=w460, "Point1 (Pixels)"=w461) -> ("error out"=w462:errorcluster, "midpoint"=w463:cluster{"X":sgl, "Y":sgl})  [unwired: 7 in]
            }
          }
          n115 = Build Array(w448) -> (w452:cluster{"X":sgl, "Y":sgl}[])
          n116 = Bundle By Name(cluster=w449, "Measurment Type"="point", "Measurment Name"=w451, "PointForOverlays.Points.Points"=w452) -> (w450:T12)
          n117 = Bundle By Name(cluster=w457, "VariableName"=w451, "VariableType"="Point", "PointArray"=w452) -> (w455:T14)
        }
        frame "pointAtAnAngleAndDistance" {
          w490 = T14 {"VariableName"="", "VariableType"="", "Co-sys Reference"={"Base Co-sys Reference"={"Origin"={"X"=0.0, "Y"=0.0}, "Angle (deg)"=0.0, "Axis Reference"=0, "Scale"=0.0}, "New Co-sys Reference"={"Origin"={"X"=0.0, "Y"=0.0}, "Angle (deg)"=0.0, "Axis Reference"=0, "Scale"=0.0}}, "PointArray"=[], "Line Array"=[], "CircleArrayOUT"=[], "TPDetails"={"DistanceInfo"={"X"=0.0, "Y"=0.0, "X'"=0.0, "Y'"=0.0, "DX"=0.0, "DY"=0.0, "Distance Type"=""}, "Feature and Datum details"=[]}, "Value"=[], "Display Name"=0.0, "ROIArray"=[], "Update ROI "=FALSE}  # AlgoOut
          n118 = Array Size(array=w475) -> (size(s)=w474:i32)
          n119 = Array Size(array=w472) -> (size(s)=w467:i32)
          n120 = Index Array(array=w486) -> (element=w487:T42)  [unwired: 1 in]
          n121 = Index Array(array=w475) -> (element=w494:cluster{"X":sgl, "Y":sgl})  [unwired: 1 in]
          n122 = Equal?(x=w474, y=1) -> (x = y?=w469:bool)
          n123 = Decrement(x=w467) -> (x-1=w466:i32)
          n124 = Unbundle By Name(w487) -> ("Captured Image"=w477:T3)
          n125 = Greater Or Equal?(x=w467, y=2) -> (x >= y?=w470:bool)
          n126 = Decrement(x=w466) -> (x-1=w465:i32)
          n127 = Index Array(array=w472, index #1=w465, index #2=w466) -> (element #1=w489:sgl, element #2=w488:sgl)
          n128 = And(x=w470, y=w469) -> (x .and. y?=w468:bool)
          n129 = case shown="True" w468 {
            tunnel: w494 -> [_ w502]
            tunnel: w493 -> [w495 w501]
            tunnel: w489 -> [_ w500]
            tunnel: w488 -> [_ w499]
            tunnel: [w495 w498] -> w485
            tunnel: [cluster{"X":sgl, "Y":sgl} {"X"=nan, "Y"=nan} ("distantPointAtAngle") w497] -> w476
            frame False {
            }
            frame True {
              n130 = call "distantPointAtAnAngleFromPoint.vi"("error in (no error)"=w501, "distance"=w499, "Angle (deg)"=w500, "Point"=w502) -> ("error out"=w498:errorcluster, "distantPointAtAngle"=w497:cluster{"X":sgl, "Y":sgl})  [unwired: 6 in]
            }
          }
          n131 = Build Array(w476) -> (w481:cluster{"X":sgl, "Y":sgl}[])
          n132 = Bundle By Name(cluster=w479, "Measurment Type"="point", "PointForOverlays.Points.Points"=w481, "Measurment Name"=w478) -> (w480:T12)
          n133 = Bundle By Name(cluster=w490, "VariableName"=w478, "VariableType"="Point", "PointArray"=w481) -> (w491:T14)
          n134 = case shown="True" w483 {
            tunnel: w477 -> [_ w508]
            tunnel: w485 -> [w503 w507]
            tunnel: [w503 w506] -> w484
            tunnel: w476 -> [_ w505]
            tunnel: w478 -> [_ w504]
            frame False {
            }
            frame True {
              # "measurement overlay"
              n135 = call "IMAQ Overlay Points"("Group"=w504, "error in (no error)"=w507, "Point"=w505, "Image"=w508) -> ("error out"=w506:errorcluster)  [unwired: 6 in, 1 out]
            }
          }
        }
        frame "intersectionOfCircleAndLine" {
          w533 = T14 {"VariableName"="", "VariableType"="", "Co-sys Reference"={"Base Co-sys Reference"={"Origin"={"X"=0.0, "Y"=0.0}, "Angle (deg)"=0.0, "Axis Reference"=0, "Scale"=0.0}, "New Co-sys Reference"={"Origin"={"X"=0.0, "Y"=0.0}, "Angle (deg)"=0.0, "Axis Reference"=0, "Scale"=0.0}}, "PointArray"=[], "Line Array"=[], "CircleArrayOUT"=[], "TPDetails"={"DistanceInfo"={"X"=0.0, "Y"=0.0, "X'"=0.0, "Y'"=0.0, "DX"=0.0, "DY"=0.0, "Distance Type"=""}, "Feature and Datum details"=[]}, "Value"=[], "Display Name"=0.0, "ROIArray"=[], "Update ROI "=FALSE}  # AlgoOut
          # "Overlay(Done)"
          n136 = Array Size(array=w523) -> (size(s)=w520:i32)
          n137 = Index Array(array=w524) -> (element=w527:T23)  [unwired: 1 in]
          n138 = Index Array(array=w523) -> (element=w526:T26)  [unwired: 1 in]
          n139 = Array Size(array=w524) -> (size(s)=w509:i32)
          n140 = Equal?(x=w509, y=1) -> (x = y?=w519:bool)
          n141 = Equal?(x=w520, y=1) -> (x = y?=w518:bool)
          n142 = Unbundle By Name(w527) -> ("Line"=w517:T24)
          n143 = Unbundle By Name(w526) -> ("CircleDetected"=w525:T48)
          n144 = And(x=w519, y=w518) -> (x .and. y?=w512:bool)
          n145 = case shown="True" w512 {
            tunnel: w534 -> [w535 w541]
            tunnel: [w535 w540] -> w510
            tunnel: w525 -> [_ w539]
            tunnel: [cluster{"X":sgl, "Y":sgl}[] [{"X"=nan, "Y"=nan}] ("Intersection Points Array") w538] -> w513
            tunnel: w517 -> [_ w537]
            frame False {
            }
            frame True {
              n146 = call "interCircLineMaths.vi"("error in (no error)"=w541, "linePt1Pt2"=w537, "circCentRad"=w539) -> ("error out"=w540:errorcluster, "Intersection Points Array"=w538:cluster{"X":sgl, "Y":sgl}[])  [unwired: 6 in, 1 out]
            }
          }
          n147 = Empty Array?(array=w513) -> (empty?=w511:bool)
          n148 = Select(t=cluster{"X":sgl, "Y":sgl}[] [{"X"=nan, "Y"=nan}] ("Intersection Points Array"), s=w511, f=w513) -> (s? t:f=w515:cluster{"X":sgl, "Y":sgl}[])
          n149 = Bundle By Name(cluster=w530, "Measurment Type"="point", "Measurment Name"=w528, "PointForOverlays.Points.Points"=w515) -> (w529:T12)
          n150 = Bundle By Name(cluster=w533, "VariableName"=w528, "VariableType"="Point", "PointArray"=w515) -> (w531:T14)
        }
        frame "intersectionOf2Lines" {
          w569 = T14 {"VariableName"="", "VariableType"="", "Co-sys Reference"={"Base Co-sys Reference"={"Origin"={"X"=0.0, "Y"=0.0}, "Angle (deg)"=0.0, "Axis Reference"=0, "Scale"=0.0}, "New Co-sys Reference"={"Origin"={"X"=0.0, "Y"=0.0}, "Angle (deg)"=0.0, "Axis Reference"=0, "Scale"=0.0}}, "PointArray"=[], "Line Array"=[], "CircleArrayOUT"=[], "TPDetails"={"DistanceInfo"={"X"=0.0, "Y"=0.0, "X'"=0.0, "Y'"=0.0, "DX"=0.0, "DY"=0.0, "Distance Type"=""}, "Feature and Datum details"=[]}, "Value"=[], "Display Name"=0.0, "ROIArray"=[], "Update ROI "=FALSE}  # AlgoOut
          # "Overlay(Done)"
          n151 = Index Array(array=w559) -> (element #1=w563:T23, element #2=w562:T23)  [unwired: 2 in]
          n152 = Array Size(array=w559) -> (size(s)=w558:i32)
          n153 = Unbundle By Name(w562) -> ("Line"=w554:T24)
          n154 = Unbundle By Name(w563) -> ("Line"=w555:T24)
          n155 = Equal?(x=w558, y=2) -> (x = y?=w545:bool)
          n156 = Not Equal?(x=w555, y=w554) -> (x != y?=w556:T49)
          n157 = Unbundle By Name(w556) -> ("Point 1.X"=w553:bool, "Point 1.Y"=w550:bool, "Point 2.X"=w551:bool, "Point 2.Y"=w552:bool)
          n158 = Compound Arithmetic op=OR(w553, w550, w551, w552) -> (w546:bool)
          n159 = And(x=w546, y=w545) -> (x .and. y?=w543:bool)
          n160 = case shown="True" w543 {
            tunnel: w570 -> [w572 w577]
            tunnel: [w572 w576] -> w542
            tunnel: [cluster{"X":sgl, "Y":sgl} {"X"=nan, "Y"=nan} ("Intersection Point") w575] -> w560
            tunnel: w555 -> [_ w574]
            tunnel: w554 -> [_ w573]
            frame False {
            }
            frame True {
              n161 = call "intersectionOfLines.vi"("error in (no error)"=w577, "Line 2"=w573, "Line 1"=w574) -> ("error out"=w576:errorcluster, "Intersection Point"=w575:cluster{"X":sgl, "Y":sgl})  [unwired: 7 in]
            }
          }
          n162 = Build Array(w560) -> (w549:cluster{"X":sgl, "Y":sgl}[])
          n163 = Empty Array?(array=w549) -> (empty?=w544:bool)
          n164 = Select(t=cluster{"X":sgl, "Y":sgl}[] [{"X"=nan, "Y"=nan}] ("Intersection Points Array"), s=w544, f=w549) -> (s? t:f=w547:cluster{"X":sgl, "Y":sgl}[])
          n165 = Bundle By Name(cluster=w565, "Measurment Type"="point", "Measurment Name"=w561, "PointForOverlays.Points.Points"=w547) -> (w564:T12)
          n166 = Bundle By Name(cluster=w569, "VariableName"=w561, "VariableType"="Point", "PointArray"=w547) -> (w567:T14)
        }
        frame "intersectionOf2Circles" {
          w602 = T14 {"VariableName"="", "VariableType"="", "Co-sys Reference"={"Base Co-sys Reference"={"Origin"={"X"=0.0, "Y"=0.0}, "Angle (deg)"=0.0, "Axis Reference"=0, "Scale"=0.0}, "New Co-sys Reference"={"Origin"={"X"=0.0, "Y"=0.0}, "Angle (deg)"=0.0, "Axis Reference"=0, "Scale"=0.0}}, "PointArray"=[], "Line Array"=[], "CircleArrayOUT"=[], "TPDetails"={"DistanceInfo"={"X"=0.0, "Y"=0.0, "X'"=0.0, "Y'"=0.0, "DX"=0.0, "DY"=0.0, "Distance Type"=""}, "Feature and Datum details"=[]}, "Value"=[], "Display Name"=0.0, "ROIArray"=[], "Update ROI "=FALSE}  # AlgoOut
          # "Overlay(Done)"
          n167 = Index Array(array=w593) -> (element #1=w596:T26, element #2=w595:T26)  [unwired: 2 in]
          n168 = Array Size(array=w593) -> (size(s)=w592:i32)
          n169 = Unbundle By Name(w595) -> ("CircleDetected"=w589:T48)
          n170 = Unbundle By Name(w596) -> ("CircleDetected"=w590:T48)
          n171 = Equal?(x=w592, y=2) -> (x = y?=w581:bool)
          n172 = Not Equal?(x=w590, y=w589) -> (x != y?=w588:T50)
          n173 = Unbundle By Name(w588) -> ("Center (Pixels).X"=w587:bool, "Center (Pixels).Y"=w586:bool)
          n174 = Compound Arithmetic op=OR(w587, w586) -> (w582:bool)
          n175 = And(x=w582, y=w581) -> (x .and. y?=w579:bool)
          n176 = case shown="True" w579 {
            tunnel: w603 -> [w604 w614]
            tunnel: [w604 w613] -> w578
            tunnel: [cluster{"X":sgl, "Y":sgl}[] [{"X"=nan, "Y"=nan}, {"X"=nan, "Y"=nan}] w612] -> w585
            tunnel: w590 -> [_ w611]
            tunnel: w589 -> [_ w610]
            frame False {
            }
            frame True {
              n177 = call "intersectionOf2CircMaths.vi"("error in (no error)"=w614, "centerRad2"=w610, "centerRad1"=w611) -> ("error out"=w613:errorcluster, "Point2"=w607:cluster{"X":sgl, "Y":sgl}, "Point1"=w609:cluster{"X":sgl, "Y":sgl})  [unwired: 5 in, 1 out]
              n178 = call "FEATURE_DETECTED.vi"("Point"=w609) -> ("s? t:f"=w608:cluster{"X":dbl, "Y":dbl})  [unwired: 8 in, 2 out]
              n179 = call "FEATURE_DETECTED.vi"("Point"=w607) -> ("s? t:f"=w606:cluster{"X":dbl, "Y":dbl})  [unwired: 8 in, 2 out]
              n180 = Build Array(w608, w606) -> (w612:cluster{"X":dbl, "Y":dbl}[])
            }
          }
          n181 = Empty Array?(array=w585) -> (empty?=w580:bool)
          n182 = Select(t=cluster{"X":sgl, "Y":sgl}[] [{"X"=nan, "Y"=nan}] ("Intersection Points Array"), s=w580, f=w585) -> (s? t:f=w583:cluster{"X":dbl, "Y":dbl}[])
          n183 = Bundle By Name(cluster=w602, "VariableName"=w594, "VariableType"="Point", "PointArray"=w583) -> (w600:T14)
          n184 = Bundle By Name(cluster=w598, "Measurment Type"="point", "Measurment Name"=w594, "PointForOverlays.Points.Points"=w583) -> (w597:T12)
        }
        frame "Teeth MidPoint" {
          w630 = "Point" ("VariableType")
          w635 = T14 {"VariableName"="", "VariableType"="", "Co-sys Reference"={"Base Co-sys Reference"={"Origin"={"X"=0.0, "Y"=0.0}, "Angle (deg)"=0.0, "Axis Reference"=0, "Scale"=0.0}, "New Co-sys Reference"={"Origin"={"X"=0.0, "Y"=0.0}, "Angle (deg)"=0.0, "Axis Reference"=0, "Scale"=0.0}}, "PointArray"=[], "Line Array"=[], "CircleArrayOUT"=[], "TPDetails"={"DistanceInfo"={"X"=0.0, "Y"=0.0, "X'"=0.0, "Y'"=0.0, "DX"=0.0, "DY"=0.0, "Distance Type"=""}, "Feature and Datum details"=[]}, "Value"=[], "Display Name"=0.0, "ROIArray"=[], "Update ROI "=FALSE}  # AlgoOut
          n185 = Unbundle By Name(w638) -> ("ROI"=w623:T47, "Edge Options"=w622:T5, "Circle Fit Options.Step Size"=w621:dbl, "ROI Overlay Enabled"=w616:bool)
          n186 = Index Array(array=w637) -> (element=w636:T42)  [unwired: 1 in]
          n187 = Unbundle By Name(w636) -> ("Captured Image"=w624:T3)
          n188 = call "teeth mid point.vi"("Image In"=w624, "group name"=w617, "ROI Descriptor"=w623, "Edge Options"=w622, "Step Size"=w621, "error in (no error)"=w620, "ROI Enable"=w616, "Measurement Overlay enabled"=w615) -> ("Mid Point of Teeth"=w619:cluster{sgl, sgl}, "error out"=w618:errorcluster)  [unwired: 6 in]
          n189 = call "point_within_img.vi"("error in (no error)"=w618, "Image"=w624, "Point"=w619) -> ("error out"=w627:errorcluster, "Point"=w628:cluster{"Point X":dbl, "Point Y":dbl})  [unwired: 6 in, 1 out]
          n190 = call "FEATURE_DETECTED.vi"("error in (no error)"=w627, "Point"=w628) -> ("error out"=w625:errorcluster, "s? t:f"=w626:cluster{"X":dbl, "Y":dbl})  [unwired: 7 in, 1 out]
          n191 = Build Array(w626) -> (w631:cluster{"X":dbl, "Y":dbl}[])
          n192 = Build Array(w626) -> (w634:cluster{"X":dbl, "Y":dbl}[])
          n193 = Bundle By Name(cluster=w632, "Measurment Name"=w617, "PointForOverlays.Points.Points"=w631, "Measurment Type"=w630) -> (w629:T12)
          n194 = Bundle By Name(cluster=w635, "VariableName"=w617, "VariableType"=w630, "PointArray"=w634) -> (w633:T14)
        }
        frame "BlobCentre" {
          w642 = T51 {"Global Rectangle"=[], "Contours"=[]}  # ROI Descriptor
          w653 = "Point" ("VariableType")
          w658 = T14 {"VariableName"="", "VariableType"="", "Co-sys Reference"={"Base Co-sys Reference"={"Origin"={"X"=0.0, "Y"=0.0}, "Angle (deg)"=0.0, "Axis Reference"=0, "Scale"=0.0}, "New Co-sys Reference"={"Origin"={"X"=0.0, "Y"=0.0}, "Angle (deg)"=0.0, "Axis Reference"=0, "Scale"=0.0}}, "PointArray"=[], "Line Array"=[], "CircleArrayOUT"=[], "TPDetails"={"DistanceInfo"={"X"=0.0, "Y"=0.0, "X'"=0.0, "Y'"=0.0, "DX"=0.0, "DY"=0.0, "Distance Type"=""}, "Feature and Datum details"=[]}, "Value"=[], "Display Name"=0.0, "ROIArray"=[], "Update ROI "=FALSE}  # AlgoOut
          n195 = Unbundle By Name(w661) -> ("ROI"=w649:T47, "Edge Options.Minimum Edge Strength"=w646:sgl)
          n196 = Index Array(array=w660) -> (element=w659:T42)  [unwired: 1 in]
          n197 = Unbundle By Name(w659) -> ("Captured Image"=w650:T3)  [unwired: 1 out]
          n198 = call "BlobCentre.vi"("Image In"=w650, "ROI"=w649, "Edge Strength"=w646, "Conversion Factor"=w647, "error in (no error)"=w648) -> ("Centre Point(Pixels)"=w644:cluster{"X":dbl, "Y":dbl}, "ROI Transformed"=w641:bool, "error out"=w645:errorcluster)  [unwired: 8 in]
          n199 = call "IMAQ Convert Point to ROI"("Point"=w644) -> ("ROI Descriptor"=w643:T51)  [unwired: 8 in, 1 out]
          n200 = Build Array(w644) -> (w654:cluster{"X":dbl, "Y":dbl}[])
          n201 = Select(t=w643, s=w641, f=w642) -> (s? t:f=w640:T51)
          n202 = Build Array(w640) -> (w639:T51[])
          n203 = Build Array(w644) -> (w657:cluster{"X":dbl, "Y":dbl}[])
          n204 = Bundle By Name(cluster=w655, "Measurment Name"=w651, "PointForOverlays.Points.Points"=w654, "Measurment Type"=w653) -> (w652:T12)
          n205 = Bundle By Name(cluster=w658, "VariableName"=w651, "VariableType"=w653, "PointArray"=w657, "Update ROI"=w641, "ROIArray"=w639) -> (w656:T14)
        }
        frame "RootPoint" {
          w671 = "Point" ("VariableType")
          w676 = T14 {"VariableName"="", "VariableType"="", "Co-sys Reference"={"Base Co-sys Reference"={"Origin"={"X"=0.0, "Y"=0.0}, "Angle (deg)"=0.0, "Axis Reference"=0, "Scale"=0.0}, "New Co-sys Reference"={"Origin"={"X"=0.0, "Y"=0.0}, "Angle (deg)"=0.0, "Axis Reference"=0, "Scale"=0.0}}, "PointArray"=[], "Line Array"=[], "CircleArrayOUT"=[], "TPDetails"={"DistanceInfo"={"X"=0.0, "Y"=0.0, "X'"=0.0, "Y'"=0.0, "DX"=0.0, "DY"=0.0, "Distance Type"=""}, "Feature and Datum details"=[]}, "Value"=[], "Display Name"=0.0, "ROIArray"=[], "Update ROI "=FALSE}  # AlgoOut
          # "Coertion Dot because of Enum to Integer Difference"
          n206 = Unbundle By Name(w679) -> ("ROI"=w664:T47, "Edge Options"=w663:T5, "Line Options.Step Size"=w662:u32)
          n207 = Index Array(array=w678) -> (element=w677:T42)  [unwired: 1 in]
          n208 = Unbundle By Name(w677) -> ("Captured Image"=w668:T3)
          n209 = call "root point.vi"("Image In"=w668, "Annulus ROI"=w664, "Edge Options"=w663, "Step Size"=w662, "error in"=w667) -> ("Location (Pixel)"=w665:cluster{"X":sgl, "Y":sgl}, "error out"=w666:errorcluster)  [unwired: 11 in, 2 out]
          n210 = Build Array(w665) -> (w672:cluster{"X":sgl, "Y":sgl}[])
          n211 = Build Array(w665) -> (w675:cluster{"X":sgl, "Y":sgl}[])
          n212 = Bundle By Name(cluster=w673, "Measurment Name"=w669, "PointForOverlays.Points.Points"=w672, "Measurment Type"=w671) -> (w670:T12)
          n213 = Bundle By Name(cluster=w676, "VariableName"=w669, "VariableType"=w671, "PointArray"=w675) -> (w674:T14)
        }
        frame "CrestPoint" {
          w695 = "Point" ("VariableType")
          w700 = T14 {"VariableName"="", "VariableType"="", "Co-sys Reference"={"Base Co-sys Reference"={"Origin"={"X"=0.0, "Y"=0.0}, "Angle (deg)"=0.0, "Axis Reference"=0, "Scale"=0.0}, "New Co-sys Reference"={"Origin"={"X"=0.0, "Y"=0.0}, "Angle (deg)"=0.0, "Axis Reference"=0, "Scale"=0.0}}, "PointArray"=[], "Line Array"=[], "CircleArrayOUT"=[], "TPDetails"={"DistanceInfo"={"X"=0.0, "Y"=0.0, "X'"=0.0, "Y'"=0.0, "DX"=0.0, "DY"=0.0, "Distance Type"=""}, "Feature and Datum details"=[]}, "Value"=[], "Display Name"=0.0, "ROIArray"=[], "Update ROI "=FALSE}  # AlgoOut
          # "Coertion Dot because of Enum to Integer Difference"
          n214 = Index Array(array=w702) -> (element=w701:T42)  [unwired: 1 in]
          n215 = Unbundle By Name(w703) -> ("ROI"=w684:T47, "Edge Options"=w690:T5, "Line Options.Step Size"=w689:u32)
          n216 = Unbundle By Name(w701) -> ("Captured Image"=w683:T3)
          n217 = case shown="True" w680 {
            tunnel: w685 -> [w705 w710]
            tunnel: w684 -> [_ w709]
            tunnel: w683 -> [w704 w708]
            tunnel: [w704 w707] -> w682
            tunnel: [w705 w706] -> w681
            frame False {
            }
            frame True {
              n218 = call "IMAQ Overlay ROI"("error in (no error)"=w710, "ROI Descriptor"=w709, "Image"=w708) -> ("error out"=w706:errorcluster, "Image Out"=w707:T3)  [unwired: 7 in]
            }
          }
          n219 = call "crest point.vi"("Image In"=w682, "Annular ROI"=w684, "Edge Options"=w690, "Step Size"=w689, "calib image"=w688, "Conversion Factor"=w687, "Conversion Factor Y/N"=w686, "error in"=w681) -> ("Location (Pixel)"=w691:cluster{"X":sgl, "Y":sgl}, "error out"=w692:errorcluster)  [unwired: 16 in, 2 out]
          n220 = Build Array(w691) -> (w696:cluster{"X":sgl, "Y":sgl}[])
          n221 = Build Array(w691) -> (w699:cluster{"X":sgl, "Y":sgl}[])
          n222 = Bundle By Name(cluster=w697, "Measurment Name"=w693, "PointForOverlays.Points.Points"=w696, "Measurment Type"=w695) -> (w694:T12)
          n223 = Bundle By Name(cluster=w700, "VariableName"=w693, "VariableType"=w695, "PointArray"=w699) -> (w698:T14)
        }
        frame "---- line detection method----" {
        }
        frame "lineDirect" {
          w753 = T39 {"Options"={"Search Direction"=0, "Edge Options"={"Edge Polarity"=0, "Kernel Size"=3, "Width"=3, "Minimum Edge Strength"=10.0, "Interpolation Type"=enum."Bilinear Fixed", "Data Processing Method"=enum."Average"}, "Show Search Area"=FALSE, "Show Search Lines"=FALSE, "Show Edges Found"=FALSE, "Show Result"=TRUE, "Search Area Color"=65280, "Search Lines Color"=255, "Edge Locations Color"=16776960, "Result Color"=16711680, "Overlay Group Name"=""}, "Line Fit Options"={"Number of Lines"=1, "Type"=enum."First Edge Rake", "Min. Score"=10.0, "Max. Score"=1000.0, "Orientation"=0.0, "Angle Range"=45.0, "Angle Tolerance"=1.0, "Step Size"=7, "Min. SNR (db)"=0.0, "Min. Points (%)"=25.0, "Hough Iterations"=5}}  # LineSettings
          w756 = T14 {"VariableName"="", "VariableType"="", "Co-sys Reference"={"Base Co-sys Reference"={"Origin"={"X"=0.0, "Y"=0.0}, "Angle (deg)"=0.0, "Axis Reference"=0, "Scale"=0.0}, "New Co-sys Reference"={"Origin"={"X"=0.0, "Y"=0.0}, "Angle (deg)"=0.0, "Axis Reference"=0, "Scale"=0.0}}, "PointArray"=[], "Line Array"=[], "CircleArrayOUT"=[], "TPDetails"={"DistanceInfo"={"X"=0.0, "Y"=0.0, "X'"=0.0, "Y'"=0.0, "DX"=0.0, "DY"=0.0, "Distance Type"=""}, "Feature and Datum details"=[]}, "Value"=[], "Display Name"=0.0, "ROIArray"=[], "Update ROI "=FALSE}  # AlgoOut
          # "Overlay(Done)"
          n224 = Unbundle By Name(w744) -> ("Search Direction"=w752:u16, "Edge threshold"=w751:dbl, "Edge Options"=w750:T5, "Line Options"=w749:T7, "ROI Overlay Enabled"=w724:bool, "ROI"=w741:T47)
          n225 = Index Array(array=w746) -> (element=w747:T42)  [unwired: 1 in]
          n226 = Unbundle By Name(w747) -> ("Captured Image"=w728:T3)
          n227 = case shown="True" w724 {
            tunnel: w748 -> [w757 w763]
            tunnel: [w757 w762] -> w743
            tunnel: w728 -> [w758 w761]
            tunnel: [w758 w760] -> w715
            tunnel: w741 -> [_ w759]
            frame False {
            }
            frame True {
              # "ROI overlay"
              n228 = call "IMAQ Overlay ROI"("error in (no error)"=w763, "ROI Descriptor"=w759, "Image"=w761) -> ("error out"=w762:errorcluster, "Image Out"=w760:T3)  [unwired: 7 in]
            }
          }
          n229 = Bundle By Name(cluster=w753, "Options.Search Direction"=w752, "Options.Edge Options.Minimum Edge Strength"=w751, "Options.Edge Options"=w750, "Line Fit Options"=w749, "Options.Show Result"=w725, "Options.Overlay Group Name"=w738) -> (w742:T39)
          n230 = call "lineDetectDirect.vi"("Image"=w715, "Settings"=w742, "ROI Descriptor"=w741, "error in (no error)"=w743) -> ("lineDetected"=w732:T32, "Straight Edges"=w737:T52, "Used Edges"=w736:cluster{"Edge Information":T15[]}[], "error out"=w722:errorcluster)  [unwired: 6 in, 2 out]
          n231 = Unbundle(w732) -> ("Point1 (Pixels)"=w731:cluster{"X":sgl, "Y":sgl}, "Point2 (Pixels)"=w729:cluster{"X":sgl, "Y":sgl})
          n232 = call "point_within_img.vi"("error in (no error)"=w722, "Image"=w728, "Point"=w731) -> ("error out"=w719:errorcluster, "Point"=w727:cluster{"Point X":dbl, "Point Y":dbl})  [unwired: 6 in, 1 out]
          n233 = call "point_within_img.vi"("error in (no error)"=w722, "Image"=w728, "Point"=w729) -> ("error out"=w718:errorcluster, "Point"=w726:cluster{"Point X":dbl, "Point Y":dbl})  [unwired: 6 in, 1 out]
          n234 = call "FEATURE_DETECTED.vi"("error in (no error)"=w718, "Point"=w726) -> ("error out"=w716:errorcluster, "s? t:f"=w720:cluster{"X":dbl, "Y":dbl})  [unwired: 7 in, 1 out]
          n235 = call "FEATURE_DETECTED.vi"("error in (no error)"=w719, "Point"=w727) -> ("error out"=w717:errorcluster, "s? t:f"=w723:cluster{"X":dbl, "Y":dbl}, "x .and. y?"=w714:bool)  [unwired: 7 in]
          n236 = Bundle("s? t:f"=w723, "s? t:f"=w720) -> (w730:T53)  [unwired: 1 in]
          n237 = Not(x=w714) -> ()  [unwired: 1 out]
          n238 = Merge Errors(w717, w716) -> (w721:errorcluster)
          n239 = Bundle(w730, "Straight Edges"=w737, "Used Edges"=w736) -> (w735:T54)  [unwired: 1 in]
          n240 = Build Array(w735) -> (w734:T55)
          n241 = Build Array(w730) -> (w733:T56)
          n242 = Bundle By Name(cluster=w740, "Measurment Type"="Line", "PointForOverlays.Line"=w733, "Measurment Name"=w738) -> (w739:T12)
          n243 = Bundle By Name(cluster=w756, "VariableName"=w738, "VariableType"="Line", "Line Array"=w734, "Update ROI"=FALSE) -> (w754:T14)
        }
        frame "MultipleLineDetect" {
          w788 = T14 {"VariableName"="", "VariableType"="", "Co-sys Reference"={"Base Co-sys Reference"={"Origin"={"X"=0.0, "Y"=0.0}, "Angle (deg)"=0.0, "Axis Reference"=0, "Scale"=0.0}, "New Co-sys Reference"={"Origin"={"X"=0.0, "Y"=0.0}, "Angle (deg)"=0.0, "Axis Reference"=0, "Scale"=0.0}}, "PointArray"=[], "Line Array"=[], "CircleArrayOUT"=[], "TPDetails"={"DistanceInfo"={"X"=0.0, "Y"=0.0, "X'"=0.0, "Y'"=0.0, "DX"=0.0, "DY"=0.0, "Distance Type"=""}, "Feature and Datum details"=[]}, "Value"=[], "Display Name"=0.0, "ROIArray"=[], "Update ROI "=FALSE}  # AlgoOut
          n244 = Unbundle By Name(w781) -> ("Edge Options"=w774:T5, "Search Direction"=w773:u16, "Line Options.Step Size"=w772:u32, "ROI Overlay Enabled"=w777:bool, "ROI"=w775:T47)
          n245 = Index Array(array=w783) -> (element=w784:T42)  [unwired: 1 in]
          n246 = Unbundle By Name(w784) -> ("Captured Image"=w778:T3)
          n247 = case shown="True" w777 {
            tunnel: w785 -> [w803 w809]
            tunnel: [w803 w808] -> w771
            tunnel: w778 -> [w804 w807]
            tunnel: [w804 w806] -> w776
            tunnel: w775 -> [_ w805]
            frame False {
            }
            frame True {
              # "ROI overlay"
              n248 = call "IMAQ Overlay ROI"("error in (no error)"=w809, "ROI Descriptor"=w805, "Image"=w807) -> ("error out"=w808:errorcluster, "Image Out"=w806:T3)  [unwired: 7 in]
            }
          }
          n249 = call "Multiple Line Edge Detection.vi"("Image Out"=w776, "ROI Descriptor"=w775, "Edge Options"=w774, "Scan Direction"=w773, "Step Size"=w772, "error in (no error)"=w771) -> ("Image Out"=w765:T3, "Line"=w769:T18, "error out"=w767:errorcluster)  [unwired: 19 in]
          n250 = for {
            tunnel: w769 -> [w802] mode=indexing
            tunnel: [w801] -> w764 mode=indexing
            n251 = Unbundle By Name(w802) -> ("Line"=w801:T24)
          }
          n252 = case shown="False" w768 {
            tunnel: w767 -> [w789 w793]
            tunnel: [w789 w792] -> w766
            tunnel: w765 -> [_ w791]
            tunnel: w764 -> [_ w790]
            frame False {
            }
            frame True {
              # "Measurement Overlay enabled"
              n253 = for {
                shift-right: [w799] -> w792
                shift-left: w793 -> [w800]
                tunnel: w790 -> [w797] mode=indexing
                shift-right: [w794] -> _
                shift-left: w791 -> [w798]
                n254 = Unbundle By Name(w797) -> ("Point 1"=w795:cluster{"X":sgl, "Y":sgl}, "Point 2"=w796:cluster{"X":sgl, "Y":sgl})
                n255 = call "IMAQ Overlay Line"("error in (no error)"=w800, "End Point"=w796, "Start Point"=w795, "Image"=w798) -> ("error out"=w799:errorcluster, "Image Out"=w794:T3)  [unwired: 6 in]
              }
            }
          }
          n256 = Bundle By Name(cluster=w780, "Measurment Name"=w770, "Measurment Type"="Line", "PointForOverlays.Line"=w764) -> (w779:T12)
          n257 = Bundle By Name(cluster=w788, "VariableName"=w770, "VariableType"="Line", "Line Array"=w769) -> (w786:T14)
        }
        frame "connectDividedLines" {
          w834 = T14 {"VariableName"="", "VariableType"="", "Co-sys Reference"={"Base Co-sys Reference"={"Origin"={"X"=0.0, "Y"=0.0}, "Angle (deg)"=0.0, "Axis Reference"=0, "Scale"=0.0}, "New Co-sys Reference"={"Origin"={"X"=0.0, "Y"=0.0}, "Angle (deg)"=0.0, "Axis Reference"=0, "Scale"=0.0}}, "PointArray"=[], "Line Array"=[], "CircleArrayOUT"=[], "TPDetails"={"DistanceInfo"={"X"=0.0, "Y"=0.0, "X'"=0.0, "Y'"=0.0, "DX"=0.0, "DY"=0.0, "Distance Type"=""}, "Feature and Datum details"=[]}, "Value"=[], "Display Name"=0.0, "ROIArray"=[], "Update ROI "=FALSE}  # AlgoOut
          n258 = for {
            tunnel: w819 -> [w843] mode=indexing
            tunnel: [w842] -> w813 mode=indexing
            n259 = Unbundle By Name(w843) -> ("Line"=w842:T24)
          }
          n260 = Index Array(array=w829) -> (element=w830:T42)  [unwired: 1 in]
          n261 = Unbundle By Name(w830) -> ("Captured Image"=w815:T3)
          n262 = Array Size(array=w813) -> (size(s)=w812:i32)
          n263 = Greater Or Equal?(x=w812, y=1) -> (x >= y?=w810:bool)
          n264 = case shown="True" w810 {
            tunnel: w835 -> [w837 w841]
            tunnel: [w837 w840] -> w828
            tunnel: [T24 {"Point 1"={"X"=nan, "Y"=nan}, "Point 2"={"X"=nan, "Y"=nan}} ("LineJoining") w839] -> w814
            tunnel: w813 -> [_ w838]
            frame False {
            }
            frame True {
              n265 = call "connectDividedLines.vi"("error in (no error)"=w841, "LineArray"=w838) -> ("error out"=w840:errorcluster, "LineJoining"=w839:T24)  [unwired: 8 in]
            }
          }
          n266 = Unbundle(w814) -> ("Point 1"=w823:cluster{"X":sgl, "Y":sgl}, "Point 2"=w822:cluster{"X":sgl, "Y":sgl})
          n267 = Build Array(w814) -> (w824:T31)
          n268 = Bundle By Name(cluster=T23 {"Line"={"Point 1"={"X"=0.0, "Y"=0.0}, "Point 2"={"X"=0.0, "Y"=0.0}}, "Straight Edges"=[], "Used Edges"=[]} ("Line"), "Line"=w814) -> (w817:T23)
          n269 = Build Array(w817) -> (w816:T18)
          n270 = case shown="True" w826 {
            tunnel: w815 -> [_ w847]
            tunnel: w828 -> [w844 w848]
            tunnel: [w844 w849] -> w827
            tunnel: w823 -> [_ w846]
            tunnel: w822 -> [_ w845]
            frame False {
              # "Measurement overlay disabled"
            }
            frame True {
              # "Measurement overlay enabled"
              n271 = call "IMAQ Overlay Line"("error in (no error)"=w848, "End Point"=w845, "Start Point"=w846, "Image"=w847) -> ("error out"=w849:errorcluster)  [unwired: 6 in, 1 out]
            }
          }
          n272 = Bundle By Name(cluster=w821, "Measurment Type"="Line", "Measurment Name"=w831, "PointForOverlays.Line"=w824) -> (w820:T12)
          n273 = Bundle By Name(cluster=w834, "VariableName"=w831, "VariableType"="Line", "Line Array"=w816) -> (w832:T14)
        }
        frame "shiftPointsAndLines" {
          w859 = cluster{"dx":dbl, "dy":dbl} {"dx"=0.0, "dy"=0.0}  # shift
          n274 = Index Array(array=w855, index #1=1 ("index")) -> (element #1=w858:sgl, element #2=w857:sgl)  [unwired: 1 in]
          n275 = Bundle By Name(cluster=w859, "dx"=w858, "dy"=w857) -> (w856:cluster{"dx":dbl, "dy":dbl})
          n276 = for {
            tunnel: w852 -> [w869] mode=indexing
            tunnel: [w868] -> w851 mode=indexing
            n277 = Unbundle By Name(w869) -> ("Line"=w868:T24)
          }
          n278 = call "Shift Points  Lines.vi"("error in (no error)"=w867, "shift"=w856, "Array of Points"=w866, "Array of Lines"=w851) -> ("error out"=w863:errorcluster, "line/point"=w865:u32, "Array of Shifted Points"=w850:cluster{"X":dbl, "Y":dbl}[], "Array"=w864:T18)  [unwired: 4 in]
          n279 = case shown="2" w865 {
            tunnel: w864 -> [_ w876]
            tunnel: w850 -> [w871 _]
            tunnel: w863 -> [w875 w881]
            tunnel: [w875 w881] -> w861
            tunnel: w862 -> [w872 w879]
            tunnel: [w870 w877] -> w853
            frame 1, Default {
              w874 = T14 {"VariableName"="", "VariableType"="", "Co-sys Reference"={"Base Co-sys Reference"={"Origin"={"X"=0.0, "Y"=0.0}, "Angle (deg)"=0.0, "Axis Reference"=0, "Scale"=0.0}, "New Co-sys Reference"={"Origin"={"X"=0.0, "Y"=0.0}, "Angle (deg)"=0.0, "Axis Reference"=0, "Scale"=0.0}}, "PointArray"=[], "Line Array"=[], "CircleArrayOUT"=[], "TPDetails"={"DistanceInfo"={"X"=0.0, "Y"=0.0, "X'"=0.0, "Y'"=0.0, "DX"=0.0, "DY"=0.0, "Distance Type"=""}, "Feature and Datum details"=[]}, "Value"=[], "Display Name"=0.0, "ROIArray"=[], "Update ROI "=FALSE}  # AlgoOut
              n280 = Bundle By Name(cluster=w874, "VariableName"=w872, "VariableType"="Point", "PointArray"=w871) -> (w870:T14)
            }
            frame 2 {
              n281 = Bundle By Name(cluster=T14 {"VariableName"="", "VariableType"="", "Co-sys Reference"={"Base Co-sys Reference"={"Origin"={"X"=0.0, "Y"=0.0}, "Angle (deg)"=0.0, "Axis Reference"=0, "Scale"=0.0}, "New Co-sys Reference"={"Origin"={"X"=0.0, "Y"=0.0}, "Angle (deg)"=0.0, "Axis Reference"=0, "Scale"=0.0}}, "PointArray"=[], "Line Array"=[], "CircleArrayOUT"=[], "TPDetails"={"DistanceInfo"={"X"=0.0, "Y"=0.0, "X'"=0.0, "Y'"=0.0, "DX"=0.0, "DY"=0.0, "Distance Type"=""}, "Feature and Datum details"=[]}, "Value"=[], "Display Name"=0.0, "ROIArray"=[], "Update ROI "=FALSE} ("AlgoOut"), "VariableName"=w879, "VariableType"="Line", "Line Array"=w876) -> (w877:T14)
            }
          }
        }
        frame "approximateLineByPoints" {
          w905 = T14 {"VariableName"="", "VariableType"="", "Co-sys Reference"={"Base Co-sys Reference"={"Origin"={"X"=0.0, "Y"=0.0}, "Angle (deg)"=0.0, "Axis Reference"=0, "Scale"=0.0}, "New Co-sys Reference"={"Origin"={"X"=0.0, "Y"=0.0}, "Angle (deg)"=0.0, "Axis Reference"=0, "Scale"=0.0}}, "PointArray"=[], "Line Array"=[], "CircleArrayOUT"=[], "TPDetails"={"DistanceInfo"={"X"=0.0, "Y"=0.0, "X'"=0.0, "Y'"=0.0, "DX"=0.0, "DY"=0.0, "Distance Type"=""}, "Feature and Datum details"=[]}, "Value"=[], "Display Name"=0.0, "ROIArray"=[], "Update ROI "=FALSE}  # AlgoOut
          n282 = Index Array(array=w900) -> (element=w901:T42)  [unwired: 1 in]
          n283 = Unbundle By Name(w901) -> ("Captured Image"=w887:T3)
          n284 = Array Size(array=w885) -> (size(s)=w884:i32)
          n285 = Greater Or Equal?(x=w884, y=2) -> (x >= y?=w882:bool)
          n286 = case shown="True" w882 {
            tunnel: w906 -> [w908 w912]
            tunnel: [w908 w911] -> w899
            tunnel: [T24 {"Point 1"={"X"=nan, "Y"=nan}, "Point 2"={"X"=nan, "Y"=nan}} ("Line Segment") w910] -> w886
            tunnel: w885 -> [_ w909]
            frame False {
            }
            frame True {
              n287 = call "aprroximateLineByPoints.vi"("error in (no error)"=w912, "PointArray"=w909) -> ("error out"=w911:errorcluster, "Line Segment"=w910:T24)  [unwired: 8 in]
            }
          }
          n288 = Unbundle(w886) -> ("Point 1"=w894:cluster{"X":sgl, "Y":sgl}, "Point 2"=w895:cluster{"X":sgl, "Y":sgl})
          n289 = Build Array(w886) -> (w893:T31)
          n290 = Bundle By Name(cluster=T23 {"Line"={"Point 1"={"X"=0.0, "Y"=0.0}, "Point 2"={"X"=0.0, "Y"=0.0}}, "Straight Edges"=[], "Used Edges"=[]} ("Line"), "Line"=w886) -> (w889:T23)
          n291 = case shown="True" w897 {
            tunnel: w887 -> [_ w916]
            tunnel: w899 -> [w913 w918]
            tunnel: [w913 w917] -> w898
            tunnel: w895 -> [_ w915]
            tunnel: w894 -> [_ w914]
            frame False {
              # "Measurement overlay disabled"
            }
            frame True {
              # "Measurement overlay enabled"
              n292 = call "IMAQ Overlay Line"("error in (no error)"=w918, "End Point"=w915, "Start Point"=w914, "Image"=w916) -> ("error out"=w917:errorcluster)  [unwired: 6 in, 1 out]
            }
          }
          n293 = Bundle By Name(cluster=w891, "Measurment Type"="Line", "Measurment Name"=w902, "PointForOverlays.Line"=w893) -> (w892:T12)
          n294 = Build Array(w889) -> (w888:T18)
          n295 = Bundle By Name(cluster=w905, "VariableName"=w902, "VariableType"="Line", "Line Array"=w888) -> (w903:T14)
        }
        frame "parallelLinePassingThroughPoint" {
          w949 = T14 {"VariableName"="", "VariableType"="", "Co-sys Reference"={"Base Co-sys Reference"={"Origin"={"X"=0.0, "Y"=0.0}, "Angle (deg)"=0.0, "Axis Reference"=0, "Scale"=0.0}, "New Co-sys Reference"={"Origin"={"X"=0.0, "Y"=0.0}, "Angle (deg)"=0.0, "Axis Reference"=0, "Scale"=0.0}}, "PointArray"=[], "Line Array"=[], "CircleArrayOUT"=[], "TPDetails"={"DistanceInfo"={"X"=0.0, "Y"=0.0, "X'"=0.0, "Y'"=0.0, "DX"=0.0, "DY"=0.0, "Distance Type"=""}, "Feature and Datum details"=[]}, "Value"=[], "Display Name"=0.0, "ROIArray"=[], "Update ROI "=FALSE}  # AlgoOut
          n296 = Index Array(array=w926) -> (element=w934:T23)  [unwired: 1 in]
          n297 = Index Array(array=w944) -> (element=w945:T42)  [unwired: 1 in]
          n298 = Unbundle By Name(w934) -> ("Line"=w933:T24)
          n299 = Index Array(array=w927) -> (element=w950:cluster{"X":sgl, "Y":sgl})  [unwired: 1 in]
          n300 = Unbundle By Name(w945) -> ("Captured Image"=w929:T3)
          n301 = Array Size(array=w926) -> (size(s)=w922:i32)
          n302 = Array Size(array=w927) -> (size(s)=w925:i32)
          n303 = Greater Or Equal?(x=w922, y=1) -> (x >= y?=w920:bool)
          n304 = Greater Or Equal?(x=w925, y=1) -> (x >= y?=w921:bool)
          n305 = And(x=w921, y=w920) -> (x .and. y?=w919:bool)
          n306 = case shown="True" w919 {
            tunnel: w951 -> [w953 w958]
            tunnel: w950 -> [_ w957]
            tunnel: [w953 w956] -> w943
            tunnel: w933 -> [_ w955]
            tunnel: [T24 {"Point 1"={"X"=nan, "Y"=nan}, "Point 2"={"X"=nan, "Y"=nan}} ("Bisecting Line") w954] -> w928
            frame False {
            }
            frame True {
              n307 = call "ParallelLinePassingThroughPoint.vi"("error in (no error)"=w958, "Location (Pixel)"=w957, "Line"=w955) -> ("error out"=w956:errorcluster, "Bisecting Line"=w954:T24)  [unwired: 7 in]
            }
          }
          n308 = Unbundle(w928) -> ("Point 1"=w938:cluster{"X":sgl, "Y":sgl}, "Point 2"=w937:cluster{"X":sgl, "Y":sgl})
          n309 = Bundle By Name(cluster=T23 {"Line"={"Point 1"={"X"=0.0, "Y"=0.0}, "Point 2"={"X"=0.0, "Y"=0.0}}, "Straight Edges"=[], "Used Edges"=[]} ("Line"), "Line"=w928) -> (w931:T23)
          n310 = Build Array(w928) -> (w940:T31)
          n311 = Build Array(w931) -> (w930:T18)
          n312 = case shown="False" w939 {
            tunnel: w929 -> [w959 w963]
            tunnel: [w959 w964] -> _
            tunnel: w943 -> [w960 w966]
            tunnel: [w960 w965] -> w942
            tunnel: w938 -> [_ w962]
            tunnel: w937 -> [_ w961]
            frame False {
              # "Measurement overlay disabled"
            }
            frame True {
              # "Measurement overlay enabled"
              n313 = call "IMAQ Overlay Line"("error in (no error)"=w966, "End Point"=w961, "Start Point"=w962, "Image"=w963) -> ("error out"=w965:errorcluster, "Image Out"=w964:T3)  [unwired: 6 in]
            }
          }
          n314 = Bundle By Name(cluster=w936, "Measurment Type"="Line", "Measurment Name"=w946, "PointForOverlays.Line"=w940) -> (w935:T12)
          n315 = Bundle By Name(cluster=w949, "VariableName"=w946, "VariableType"="Line", "Line Array"=w930) -> (w947:T14)
        }
        frame "tangentLines2Circle" {
          w987 = T14 {"VariableName"="", "VariableType"="", "Co-sys Reference"={"Base Co-sys Reference"={"Origin"={"X"=0.0, "Y"=0.0}, "Angle (deg)"=0.0, "Axis Reference"=0, "Scale"=0.0}, "New Co-sys Reference"={"Origin"={"X"=0.0, "Y"=0.0}, "Angle (deg)"=0.0, "Axis Reference"=0, "Scale"=0.0}}, "PointArray"=[], "Line Array"=[], "CircleArrayOUT"=[], "TPDetails"={"DistanceInfo"={"X"=0.0, "Y"=0.0, "X'"=0.0, "Y'"=0.0, "DX"=0.0, "DY"=0.0, "Distance Type"=""}, "Feature and Datum details"=[]}, "Value"=[], "Display Name"=0.0, "ROIArray"=[], "Update ROI "=FALSE}  # AlgoOut
          # "Overlay(Done)"
          n316 = Array Size(array=w977) -> (size(s)=w976:i32)
          n317 = Index Array(array=w977) -> (element #1=w981:T26, element #2=w980:T26)  [unwired: 2 in]
          n318 = Equal?(x=w976, y=2) -> (x = y?=w968:bool)
          n319 = Unbundle By Name(w980) -> ("CircleDetected"=w974:T48)
          n320 = Unbundle By Name(w981) -> ("CircleDetected"=w973:T48)
          n321 = case shown="True" w968 {
            tunnel: w988 -> [w990 w995]
            tunnel: [w990 w994] -> w967
            tunnel: [T18 [{"Line"={"Point 1"={"X"=nan, "Y"=nan}, "Point 2"={"X"=nan, "Y"=nan}}, "Straight Edges"=[], "Used Edges"=[]}, {"Line"={"Point 1"={"X"=nan, "Y"=nan}, "Point 2"={"X"=nan, "Y"=nan}}, "Straight Edges"=[], "Used Edges"=[]}] w993] -> w970
            tunnel: w974 -> [_ w992]
            tunnel: w973 -> [_ w991]
            frame False {
            }
            frame True {
              n322 = call "tangentLinesMaths.vi"("error in (no error)"=w995, "centRad2"=w992, "centRad1"=w991) -> ("error out"=w994:errorcluster, "tangentLinesArray"=w993:T18)  [unwired: 7 in]
            }
          }
          n323 = Empty Array?(array=w970) -> (empty?=w972:bool)
          n324 = Select(t=T18 [{"Line"={"Point 1"={"X"=nan, "Y"=nan}, "Point 2"={"X"=nan, "Y"=nan}}, "Straight Edges"=[], "Used Edges"=[]}, {"Line"={"Point 1"={"X"=nan, "Y"=nan}, "Point 2"={"X"=nan, "Y"=nan}}, "Straight Edges"=[], "Used Edges"=[]}], s=w972, f=w970) -> (s? t:f=w969:T18)
          n325 = for {
            tunnel: w969 -> [w997] mode=indexing
            tunnel: [w996] -> w979 mode=indexing
            n326 = Unbundle By Name(w997) -> ("Line"=w996:T24)
          }
          n327 = Bundle By Name(cluster=w983, "Measurment Type"="Line", "Measurment Name"=w978, "PointForOverlays.Line"=w979) -> (w982:T12)
          n328 = Bundle By Name(cluster=w987, "VariableName"=w978, "VariableType"="Line", "Line Array"=w969) -> (w985:T14)
        }
        frame "angleBisectingLineOf2Lines" {
          w1025 = T14 {"VariableName"="", "VariableType"="", "Co-sys Reference"={"Base Co-sys Reference"={"Origin"={"X"=0.0, "Y"=0.0}, "Angle (deg)"=0.0, "Axis Reference"=0, "Scale"=0.0}, "New Co-sys Reference"={"Origin"={"X"=0.0, "Y"=0.0}, "Angle (deg)"=0.0, "Axis Reference"=0, "Scale"=0.0}}, "PointArray"=[], "Line Array"=[], "CircleArrayOUT"=[], "TPDetails"={"DistanceInfo"={"X"=0.0, "Y"=0.0, "X'"=0.0, "Y'"=0.0, "DX"=0.0, "DY"=0.0, "Distance Type"=""}, "Feature and Datum details"=[]}, "Value"=[], "Display Name"=0.0, "ROIArray"=[], "Update ROI "=FALSE}  # AlgoOut
          # "Overlay(Done)"
          n329 = Index Array(array=w1011) -> (element #1=w1018:T23, element #2=w1017:T23)  [unwired: 2 in]
          n330 = Array Size(array=w1011) -> (size(s)=w1010:i32)
          n331 = Unbundle By Name(w1018) -> ("Line"=w1008:T24)
          n332 = Unbundle By Name(w1017) -> ("Line"=w1007:T24)
          n333 = Equal?(x=w1010, y=2) -> (x = y?=w1000:bool)
          n334 = Not Equal?(x=w1008, y=w1007) -> (x != y?=w1006:T49)
          n335 = Unbundle By Name(w1006) -> ("Point 1.X"=w1002:bool, "Point 1.Y"=w1003:bool, "Point 2.X"=w1004:bool, "Point 2.Y"=w1005:bool)
          n336 = Compound Arithmetic op=OR(w1002, w1003, w1004, w1005) -> (w1001:bool)
          n337 = And(x=w1001, y=w1000) -> (x .and. y?=w999:bool)
          n338 = case shown="True" w999 {
            tunnel: w1026 -> [w1027 w1033]
            tunnel: [T24 {"Point 1"={"X"=nan, "Y"=nan}, "Point 2"={"X"=nan, "Y"=nan}} ("Bisecting Line") w1032] -> w1012
            tunnel: w1008 -> [_ w1031]
            tunnel: w1007 -> [_ w1030]
            tunnel: [w1027 w1029] -> w998
            frame False {
            }
            frame True {
              n339 = call "angleBisectingLineOfTwoLines.vi"("error in (no error)"=w1033, "Line 2"=w1030, "Line 1"=w1031) -> ("error out"=w1029:errorcluster, "Bisecting Line"=w1032:T24)  [unwired: 7 in]
            }
          }
          n340 = Build Array(w1012) -> (w1021:T31)
          n341 = Bundle By Name(cluster=T23 {"Line"={"Point 1"={"X"=0.0, "Y"=0.0}, "Point 2"={"X"=0.0, "Y"=0.0}}, "Straight Edges"=[], "Used Edges"=[]} ("Line"), "Line"=w1012) -> (w1015:T23)
          n342 = Build Array(w1015) -> (w1014:T18)
          n343 = Bundle By Name(cluster=w1020, "Measurment Type"="Line", "Measurment Name"=w1013, "PointForOverlays.Line"=w1021) -> (w1019:T12)
          n344 = Bundle By Name(cluster=w1025, "VariableName"=w1013, "VariableType"="Line", "Line Array"=w1014) -> (w1023:T14)
        }
        frame "Line4mPoint2LineatAngle" {
          w1065 = T14 {"VariableName"="", "VariableType"="", "Co-sys Reference"={"Base Co-sys Reference"={"Origin"={"X"=0.0, "Y"=0.0}, "Angle (deg)"=0.0, "Axis Reference"=0, "Scale"=0.0}, "New Co-sys Reference"={"Origin"={"X"=0.0, "Y"=0.0}, "Angle (deg)"=0.0, "Axis Reference"=0, "Scale"=0.0}}, "PointArray"=[], "Line Array"=[], "CircleArrayOUT"=[], "TPDetails"={"DistanceInfo"={"X"=0.0, "Y"=0.0, "X'"=0.0, "Y'"=0.0, "DX"=0.0, "DY"=0.0, "Distance Type"=""}, "Feature and Datum details"=[]}, "Value"=[], "Display Name"=0.0, "ROIArray"=[], "Update ROI "=FALSE}  # AlgoOut
          # "Overlay(Done)"
          # "finds the perpendicular distance from the point to the line"
          n345 = Array Size(array=w1038) -> (size(s)=w1035:i32)
          n346 = Array Size(array=w1047) -> (size(s)=w1043:i32)
          n347 = Index Array(array=w1047) -> (element=w1052:T23)  [unwired: 1 in]
          n348 = Index Array(array=w1048) -> (element=w1060:cluster{"X":sgl, "Y":sgl})  [unwired: 1 in]
          n349 = Array Size(array=w1048) -> (size(s)=w1046:i32)
          n350 = Decrement(x=w1035) -> (x-1=w1034:i32)
          n351 = Unbundle By Name(w1052) -> ("Line"=w1051:T24)
          n352 = Greater Or Equal?(x=w1046, y=1) -> (x >= y?=w1037:bool)
          n353 = Index Array(array=w1038, index=w1034) -> (element=w1058:sgl)
          n354 = Greater Or Equal?(x=w1035, y=1) -> (x >= y?=w1036:bool)
          n355 = Greater Or Equal?(x=w1043, y=1) -> (x >= y?=w1041:bool)
          n356 = Compound Arithmetic op=AND(w1036, w1041, w1037) -> (w1040:bool)
          n357 = case shown="True" w1040 {
            tunnel: w1060 -> [_ w1073]
            tunnel: w1059 -> [w1067 w1072]
            tunnel: w1058 -> [_ w1071]
            tunnel: w1051 -> [_ w1070]
            tunnel: [w1067 w1069] -> w1039
            tunnel: [T25 {"Point 1"={"Start X"=nan, "Start Y"=nan}, "Point 2"={"End X"=nan, "End Y"=nan}} ("output line") w1068] -> w1049
            frame False {
            }
            frame True {
              n358 = call "Line_Passing_Through_Point_at_defined_angle.vi"("error in (no error)"=w1072, "Angle"=w1071, "Input Point"=w1073, "Input Line"=w1070) -> ("error out"=w1069:errorcluster, "output line"=w1068:T57)  [unwired: 6 in]
            }
          }
          n359 = Build Array(w1049) -> (w1061:T58)
          n360 = Bundle By Name(cluster=T23 {"Line"={"Point 1"={"X"=0.0, "Y"=0.0}, "Point 2"={"X"=0.0, "Y"=0.0}}, "Straight Edges"=[], "Used Edges"=[]} ("Line"), "Line"=w1049) -> (w1054:T23)
          n361 = Build Array(w1054) -> (w1053:T18)
          n362 = Bundle By Name(cluster=w1057, "Measurment Type"="Line", "Measurment Name"=w1050, "PointForOverlays.Line"=w1061) -> (w1056:T12)
          n363 = Bundle By Name(cluster=w1065, "VariableName"=w1050, "VariableType"="Line", "Line Array"=w1053) -> (w1063:T14)
        }
        frame "TangentLinesfromExternalPoints" {
          w1089 = T18 [{"Line"={"Point 1"={"X"=nan, "Y"=nan}, "Point 2"={"X"=nan, "Y"=nan}}, "Straight Edges"=[], "Used Edges"=[]}]  # NaN
          w1095 = 1 ("y")
          w1100 = "Line" ("VariableType")
          w1103 = T14 {"VariableName"="", "VariableType"="", "Co-sys Reference"={"Base Co-sys Reference"={"Origin"={"X"=0.0, "Y"=0.0}, "Angle (deg)"=0.0, "Axis Reference"=0, "Scale"=0.0}, "New Co-sys Reference"={"Origin"={"X"=0.0, "Y"=0.0}, "Angle (deg)"=0.0, "Axis Reference"=0, "Scale"=0.0}}, "PointArray"=[], "Line Array"=[], "CircleArrayOUT"=[], "TPDetails"={"DistanceInfo"={"X"=0.0, "Y"=0.0, "X'"=0.0, "Y'"=0.0, "DX"=0.0, "DY"=0.0, "Distance Type"=""}, "Feature and Datum details"=[]}, "Value"=[], "Display Name"=0.0, "ROIArray"=[], "Update ROI "=FALSE}  # AlgoOut
          # "Given Point should be outside the Circle Selected"
          n364 = Array Size(array=w1091) -> (size(s)=w1076:i32)
          n365 = Decrement(x=w1076) -> (x-1=w1077:i32)
          n366 = Array Size(array=w1092) -> (size(s)=w1096:i32)
          n367 = Index Array(array=w1092) -> (element=w1078:cluster{"X":sgl, "Y":sgl})  [unwired: 1 in]
          n368 = Index Array(array=w1091, index=w1077) -> (element=w1104:T26)
          n369 = Unbundle By Name(w1104) -> ("CircleDetected.Center (Pixels)"=w1079:cluster{"X":sgl, "Y":sgl}, "CircleDetected.Radius (Pixels)"=w1080:dbl, "CircleDetected"=w1087:T48)
          n370 = Greater Or Equal?(x=w1096, y=w1095) -> (x >= y?=w1094:bool)
          n371 = Greater Or Equal?(x=w1076, y=w1095) -> (x >= y?=w1093:bool)
          n372 = And(x=w1094, y=w1093) -> (x .and. y?=w1083:bool)
          n373 = Build Array(w1078, w1079) -> (w1086:cluster{"X":sgl, "Y":sgl}[])
          n374 = call "IMAQ Point Distances"("Points"=w1086) -> ("Distances"=w1085:sgl[])  [unwired: 4 in, 1 out]
          n375 = Index Array(array=w1085) -> (element=w1084:sgl)  [unwired: 1 in]
          n376 = Greater?(x=w1084, y=w1080) -> (0:w1082:bool)
          n377 = And(x=w1083, y=w1082) -> (x .and. y?=w1081:bool)
          n378 = case shown="True" w1081 {
            tunnel: w1105 -> [w1107 w1112]
            tunnel: w1087 -> [_ w1111]
            tunnel: [w1106 w1110] -> w1075
            tunnel: [w1107 w1109] -> w1074
            tunnel: w1078 -> [_ w1108]
            frame False {
              w1106 = T18 [{"Line"={"Point 1"={"X"=nan, "Y"=nan}, "Point 2"={"X"=nan, "Y"=nan}}, "Straight Edges"=[], "Used Edges"=[]}]  # NaN
            }
            frame True {
              n379 = call "Tangent from external Points.vi"("error in (no error)"=w1112, "Circle"=w1111, "External Point"=w1108) -> ("error out"=w1109:errorcluster, "Tangent Lines"=w1110:T18)  [unwired: 7 in]
            }
          }
          n380 = Empty Array?(array=w1075) -> (empty?=w1090:bool)
          n381 = Select(t=w1089, s=w1090, f=w1075) -> (s? t:f=w1088:T18)
          n382 = for {
            tunnel: w1088 -> [w1114] mode=indexing
            tunnel: [w1113] -> w1098 mode=indexing
            n383 = Unbundle By Name(w1114) -> ("Line"=w1113:T24)
          }
          n384 = Bundle By Name(cluster=w1103, "VariableName"=w1097, "VariableType"=w1100, "Line Array"=w1088) -> (w1102:T14)
          n385 = Bundle By Name(cluster=w1101, "PointForOverlays.Line"=w1098, "Measurment Name"=w1097, "Measurment Type"=w1100) -> (w1099:T12)
        }
        frame "LinefromPointatanAngleDist" {
          w1125 = T18 [{"Line"={"Point 1"={"X"=nan, "Y"=nan}, "Point 2"={"X"=nan, "Y"=nan}}, "Straight Edges"=[], "Used Edges"=[]}]  # NaN
          w1135 = T14 {"VariableName"="", "VariableType"="", "Co-sys Reference"={"Base Co-sys Reference"={"Origin"={"X"=0.0, "Y"=0.0}, "Angle (deg)"=0.0, "Axis Reference"=0, "Scale"=0.0}, "New Co-sys Reference"={"Origin"={"X"=0.0, "Y"=0.0}, "Angle (deg)"=0.0, "Axis Reference"=0, "Scale"=0.0}}, "PointArray"=[], "Line Array"=[], "CircleArrayOUT"=[], "TPDetails"={"DistanceInfo"={"X"=0.0, "Y"=0.0, "X'"=0.0, "Y'"=0.0, "DX"=0.0, "DY"=0.0, "Distance Type"=""}, "Feature and Datum details"=[]}, "Value"=[], "Display Name"=0.0, "ROIArray"=[], "Update ROI "=FALSE}  # AlgoOut
          n386 = Array Size(array=w1144) -> (size(s)=w1142:i32)
          n387 = Equal?(x=w1142, y=1) -> (x = y?=w1138:bool)
          n388 = Array Size(array=w1143) -> (size(s)=w1140:i32)
          n389 = Equal?(x=w1140, y=3) -> (x = y?=w1137:bool)
          n390 = And(x=w1138, y=w1137) -> (x .and. y?=w1136:bool)
          n391 = Index Array(array=w1143, index #1=2 ("index"), index #2=1 ("index"), index #3=0 ("index")) -> (element #1=w1116:sgl, element #2=w1117:sgl, element #3=w1118:sgl)
          n392 = Index Array(array=w1144) -> (element=w1121:cluster{"X":sgl, "Y":sgl})  [unwired: 1 in]
          n393 = Add(x=w1116, y=w1117) -> (x+y=w1115:sgl)
          n394 = case shown="True" w1136 {
            tunnel: w1146 -> [w1149 w1159]
            tunnel: w1121 -> [_ w1158]
            tunnel: w1115 -> [_ w1157]
            tunnel: w1118 -> [_ w1156]
            tunnel: [w1149 w1155] -> w1131
            tunnel: [w1150 w1152] -> w1124
            tunnel: w1121 -> [_ w1151]
            frame False {
              w1150 = T23 {"Line"={"Point 1"={"X"=nan, "Y"=nan}, "Point 2"={"X"=nan, "Y"=nan}}, "Straight Edges"=[], "Used Edges"=[]}  # NaN Line
            }
            frame True {
              n395 = call "LinefromPointAtAnAngleDist.vi"("error in (no error)"=w1159, "distance"=w1156, "Angle (deg)"=w1157, "Point"=w1158) -> ("error out"=w1155:errorcluster, "End Point"=w1153:cluster{"X":sgl, "Y":sgl})  [unwired: 5 in, 1 out]
              n396 = Bundle By Name(cluster=T23 {"Line"={"Point 1"={"X"=0.0, "Y"=0.0}, "Point 2"={"X"=0.0, "Y"=0.0}}, "Straight Edges"=[], "Used Edges"=[]} ("Line"), "Line.Point 1"=w1151, "Line.Point 2"=w1153) -> (w1152:T23)
            }
          }
          n397 = Build Array(w1124) -> (w1123:T18)
          n398 = Empty Array?(array=w1123) -> (empty?=w1126:bool)
          n399 = Select(t=w1125, s=w1126, f=w1123) -> (s? t:f=w1122:T18)
          n400 = for {
            tunnel: [w1148] -> w1128 mode=indexing
            tunnel: w1122 -> [w1147] mode=indexing
            n401 = Unbundle By Name(w1147) -> ("Line"=w1148:T24)
          }
          n402 = Bundle By Name(cluster=w1135, "VariableName"=w1127, "VariableType"="Line", "Line Array"=w1122) -> (w1129:T14)
          n403 = Bundle By Name(cluster=w1133, "Measurment Type"="Line", "PointForOverlays.Line"=w1128, "Measurment Name"=w1127) -> (w1130:T12)
        }
        frame "LineParalleltoaLineatDistance" {
          w1172 = T14 {"VariableName"="", "VariableType"="", "Co-sys Reference"={"Base Co-sys Reference"={"Origin"={"X"=0.0, "Y"=0.0}, "Angle (deg)"=0.0, "Axis Reference"=0, "Scale"=0.0}, "New Co-sys Reference"={"Origin"={"X"=0.0, "Y"=0.0}, "Angle (deg)"=0.0, "Axis Reference"=0, "Scale"=0.0}}, "PointArray"=[], "Line Array"=[], "CircleArrayOUT"=[], "TPDetails"={"DistanceInfo"={"X"=0.0, "Y"=0.0, "X'"=0.0, "Y'"=0.0, "DX"=0.0, "DY"=0.0, "Distance Type"=""}, "Feature and Datum details"=[]}, "Value"=[], "Display Name"=0.0, "ROIArray"=[], "Update ROI "=FALSE}  # AlgoOut
          n404 = Unbundle By Name(w1175) -> ("Width"=w1174:i32, "Height"=w1173:i32)
          n405 = Index Array "Indexing Line Array"(array=w1180) -> (element=w1179:T23)  [unwired: 1 in]
          n406 = Array Size(array=w1162) -> (size(s)=w1161:i32)
          n407 = Decrement(x=w1161) -> (x-1=w1160:i32)
          n408 = Unbundle By Name(w1179) -> ("Line"=w1178:T24)
          n409 = Index Array "Indexing Value Array"(array=w1162, index=w1160) -> (element=w1177:sgl)
          n410 = call "parallel line at a distance.vi"("Line"=w1178, "Distance in mm"=w1177, "Conversion factor"=w1176, "X resolution"=w1174, "Y resolution"=w1173, "error in (no error)"=w1181) -> ("Line Array out"=w1167:T18, "error out"=w1163:errorcluster)  [unwired: 12 in]
          n411 = for {
            tunnel: w1167 -> [w1183] mode=indexing
            tunnel: [w1182] -> w1168 mode=indexing
            n412 = Unbundle By Name(w1183) -> ("Line"=w1182:T24)
          }
          n413 = Bundle By Name(cluster=w1169, "Measurment Type"="Line", "PointForOverlays.Line"=w1168, "Measurment Name"=w1166) -> (w1164:T12)
          n414 = Bundle By Name(cluster=w1172, "VariableName"=w1166, "VariableType"="Line", "Line Array"=w1167) -> (w1165:T14)
        }
        frame "---- circle detection method----" {
        }
        frame "circleDirect" {
          w1231 = T59 {"Options"={"Search  Direction"=0, "Edge Options"={"Edge Polarity"=0, "Kernel Size"=3, "Width"=3, "Minimum Edge Strength"=50.0, "Interpolation Type"=enum."Zero Order", "Data Processing Method"=enum."Average"}, "Show Search Area"=FALSE, "Show Search Lines"=FALSE, "Show Edges Found"=FALSE, "Show Result"=FALSE, "Search Area Color"=65280, "Search Lines Color"=255, "Edge Locations Color"=16776960, "Result Color"=16711680, "Overlay Group Name"=""}, "Circle Fit Options"={"Process"=enum."Get First Edge", "Step Size"=3.0, "Max Pixel Radius"=3}}  # CircleSettings
          w1233 = T35 {"Point 1"={"X"=0.0, "Y"=0.0}, "Point 2"={"X"=0.0, "Y"=0.0}, "Center (Pixels)"={"X"=0.0, "Y"=0.0}, "Radius (Pixels)"=0.0}  # Circle
          w1236 = T14 {"VariableName"="", "VariableType"="", "Co-sys Reference"={"Base Co-sys Reference"={"Origin"={"X"=0.0, "Y"=0.0}, "Angle (deg)"=0.0, "Axis Reference"=0, "Scale"=0.0}, "New Co-sys Reference"={"Origin"={"X"=0.0, "Y"=0.0}, "Angle (deg)"=0.0, "Axis Reference"=0, "Scale"=0.0}}, "PointArray"=[], "Line Array"=[], "CircleArrayOUT"=[], "TPDetails"={"DistanceInfo"={"X"=0.0, "Y"=0.0, "X'"=0.0, "Y'"=0.0, "DX"=0.0, "DY"=0.0, "Distance Type"=""}, "Feature and Datum details"=[]}, "Value"=[], "Display Name"=0.0, "ROIArray"=[], "Update ROI "=FALSE}  # AlgoOut
          # "Overlay(Done)"
          n415 = Index Array(array=w1223) -> (element=w1224:T42)  [unwired: 1 in]
          n416 = Unbundle By Name(w1230) -> ("Search Direction"=w1229:u16, "Edge threshold"=w1228:dbl, "Edge Options"=w1227:T5, "Circle Fit Options"=w1204:T60, "ROI"=w1206:T47, "ROI Overlay Enabled"=w1219:bool)
          n417 = Unbundle By Name(w1224) -> ("Captured Image"=w1222:T3)
          n418 = case shown="False" w1219 {
            tunnel: w1226 -> [w1237 w1243]
            tunnel: [w1237 w1242] -> w1225
            tunnel: w1222 -> [w1238 w1241]
            tunnel: [w1238 w1240] -> w1210
            tunnel: w1206 -> [_ w1239]
            frame False {
              # "false"
              # "ROI overlay disabled"
            }
            frame True {
              # "ROI overlay enableed"
              n419 = call "IMAQ Overlay ROI"("error in (no error)"=w1243, "ROI Descriptor"=w1239, "Image"=w1241) -> ("error out"=w1242:errorcluster, "Image Out"=w1240:T3)  [unwired: 7 in]
            }
          }
          n420 = Bundle By Name(cluster=w1231, "Options.Overlay Group Name"=w1203, "Options.Search  Direction"=w1229, "Options.Edge Options.Minimum Edge Strength"=w1228, "Options.Edge Options"=w1227, "Circle Fit Options"=w1204, "Options.Show Result"=w1205) -> (w1220:T59)
          n421 = call "circleDetectDirect.vi"("Image"=w1210, "Settings"=w1220, "ROI Descriptor"=w1206, "error in (no error)"=w1225) -> ("ROI adjusted"=w1187:T47, "CircleDetected"=w1216:T48, "First Edges"=w1195:T15[], "Indexes of Points Used"=w1213:i32[], "error out"=w1186:errorcluster)  [unwired: 8 in, 3 out]
          n422 = Unbundle By Name(w1216) -> ("Center (Pixels)"=w1212:cluster{"X":sgl, "Y":sgl}, "Radius (Pixels)"=w1208:dbl)
          n423 = Array Size(array=w1195) -> (size(s)=w1199:i32)
          n424 = Decrement(x=w1199) -> (x-1=w1198:i32)
          n425 = call "point_within_img.vi"("Image"=w1210, "Point"=w1212) -> ("Point"=w1211:cluster{"Point X":dbl, "Point Y":dbl})  [unwired: 7 in, 2 out]
          n426 = Index Array(array=w1195, index #1=0 ("index"), index #2=w1198) -> (element #1=w1197:T15, element #2=w1196:T15)
          n427 = call "FEATURE_DETECTED.vi"("Point"=w1211) -> ("s? t:f"=w1202:cluster{"X":dbl, "Y":dbl}, "x .and. y?"=w1189:bool)  [unwired: 8 in, 1 out]
          n428 = Unbundle By Name(w1197) -> ("Location (Pixel)"=w1193:cluster{"X":sgl, "Y":sgl})
          n429 = Unbundle By Name(w1196) -> ("Location (Pixel)"=w1192:cluster{"X":sgl, "Y":sgl})
          n430 = Build Array(w1187) -> (w1191:T17)
          n431 = Select(t=nan ("f"), s=w1189, f=w1208) -> (s? t:f=w1201:dbl)
          n432 = Bundle By Name(cluster=T26 {"CircleDetected"={"Center (Pixels)"={"X"=0.0, "Y"=0.0}, "Radius (Pixels)"=0.0}, "First Edges"=[], "Indexes of Points Used"=[], "Start Point"={"X"=0.0, "Y"=0.0}, "End Point"={"X"=0.0, "Y"=0.0}} ("Circle Array"), "CircleDetected.Center (Pixels)"=w1202, "CircleDetected.Radius (Pixels)"=w1201, "First Edges"=w1195, "Indexes of Points Used"=w1213, "Start Point"=w1193, "End Point"=w1192) -> (w1215:T26)
          n433 = Bundle By Name(cluster=w1233, "Center (Pixels)"=w1202, "Radius (Pixels)"=w1201, "Point 1"=w1193, "Point 2"=w1192) -> (w1232:T35)
          n434 = Build Array(w1232) -> (w1190:T28)
          n435 = Build Array(w1215) -> (w1214:T19)
          n436 = Build Array(w1202) -> (w1207:cluster{"X":dbl, "Y":dbl}[])
          n437 = Not(x=w1189) -> (.not. x?=w1188:bool)
          n438 = Bundle By Name(cluster=w1217, "Measurment Type"="circle", "Measurment Name"=w1203, "PointForOverlays.Circle"=w1190) -> (w1218:T12)
          n439 = Bundle By Name(cluster=w1236, "VariableName"=w1203, "VariableType"="Circle", "CircleArrayOUT"=w1214, "PointArray"=w1207, "ROIArray"=w1191, "Update ROI"=w1188) -> (w1234:T14)
        }
        frame "detectAllCircles" {
          w1252 = T14 {"VariableName"="", "VariableType"="", "Co-sys Reference"={"Base Co-sys Reference"={"Origin"={"X"=0.0, "Y"=0.0}, "Angle (deg)"=0.0, "Axis Reference"=0, "Scale"=0.0}, "New Co-sys Reference"={"Origin"={"X"=0.0, "Y"=0.0}, "Angle (deg)"=0.0, "Axis Reference"=0, "Scale"=0.0}}, "PointArray"=[], "Line Array"=[], "CircleArrayOUT"=[], "TPDetails"={"DistanceInfo"={"X"=0.0, "Y"=0.0, "X'"=0.0, "Y'"=0.0, "DX"=0.0, "DY"=0.0, "Distance Type"=""}, "Feature and Datum details"=[]}, "Value"=[], "Display Name"=0.0, "ROIArray"=[], "Update ROI "=FALSE}  # AlgoOut
          n440 = Unbundle By Name(w1270) -> ("Shape Detection Settings.Circle Descriptor"=w1267:cluster{"Min Radius":dbl, "Max Radius":dbl}, "Shape Detection Settings.Curve Parameters"=w1264:T9, "ROI"=w1263:T47, "ROI Overlay Enabled"=w1262:bool)
          n441 = Index Array(array=w1271) -> (element=w1272:T42)  [unwired: 1 in]
          n442 = Unbundle By Name(w1272) -> ("Captured Image"=w1266:T3)
          n443 = case shown="True" w1262 {
            tunnel: w1266 -> [w1292 w1297]
            tunnel: w1269 -> [w1291 w1296]
            tunnel: [w1292 w1295] -> w1254
            tunnel: [w1291 w1294] -> w1268
            tunnel: w1263 -> [_ w1293]
            frame False {
              # "ROI overlay\ndisabled"
            }
            frame True {
              # "ROI overlay enabled"
              n444 = call "IMAQ Overlay ROI"("error in (no error)"=w1296, "ROI Descriptor"=w1293, "Image"=w1297) -> ("error out"=w1294:errorcluster, "Image Out"=w1295:T3)  [unwired: 7 in]
            }
          }
          n445 = call "detectCircle2.vi"("measurement overlay enable"=w1261, "Circle ROI"=w1263, "error in (no error)"=w1268, "Curve Parameters"=w1264, "Circle Descriptor"=w1267, "Image"=w1254) -> ("error out"=w1265:errorcluster, "Circle Out"=w1253:T61)  [unwired: 1 in, 2 out]
          n446 = for {
            tunnel: w1253 -> [w1281] mode=indexing
            tunnel: [w1289] -> w1249 mode=indexing
            tunnel: w1254 -> [w1285]
            tunnel: [w1276] -> w1245 mode=indexing
            w1290 = T35 {"Point 1"={"X"=0.0, "Y"=0.0}, "Point 2"={"X"=0.0, "Y"=0.0}, "Center (Pixels)"={"X"=0.0, "Y"=0.0}, "Radius (Pixels)"=0.0}  # Circle
            n447 = Unbundle By Name(w1281) -> ("CircleDetected.Center (Pixels)"=w1286:cluster{"X":sgl, "Y":sgl}, "CircleDetected.Radius (Pixels)"=w1282:dbl, "First Edges"=w1278:T15[], "Indexes of Points Used"=w1277:i32[])
            n448 = call "point_within_img.vi"("Image"=w1285, "Point"=w1286) -> ("error out"=w1288:errorcluster, "Point"=w1287:cluster{"Point X":dbl, "Point Y":dbl})  [unwired: 7 in, 1 out]
            n449 = call "FEATURE_DETECTED.vi"("error in (no error)"=w1288, "Point"=w1287) -> ("s? t:f"=w1279:cluster{"X":dbl, "Y":dbl}, "x .and. y?"=w1284:bool)  [unwired: 7 in, 1 out]
            n450 = Select(t=nan ("f"), s=w1284, f=w1282) -> (s? t:f=w1280:dbl)
            n451 = Bundle By Name(cluster=T26 {"CircleDetected"={"Center (Pixels)"={"X"=0.0, "Y"=0.0}, "Radius (Pixels)"=0.0}, "First Edges"=[], "Indexes of Points Used"=[], "Start Point"={"X"=0.0, "Y"=0.0}, "End Point"={"X"=0.0, "Y"=0.0}} ("Circle Array"), "CircleDetected.Center (Pixels)"=w1279, "CircleDetected.Radius (Pixels)"=w1280, "First Edges"=w1278, "Indexes of Points Used"=w1277) -> (w1276:T26)
            n452 = Bundle By Name(cluster=w1290, "Center (Pixels)"=w1279, "Radius (Pixels)"=w1280) -> (w1289:T35)
          }
          n453 = Empty Array?(array=w1249) -> (empty?=w1251:bool)
          n454 = Empty Array?(array=w1245) -> (empty?=w1247:bool)
          n455 = Select(t=T27 [] ("Circle Array"), s=w1247, f=w1245) -> (s? t:f=w1244:T27)
          n456 = Select(t=T28 [{"Point 1"={"X"=nan, "Y"=nan}, "Point 2"={"X"=nan, "Y"=nan}, "Center (Pixels)"={"X"=nan, "Y"=nan}, "Radius (Pixels)"=nan}], s=w1251, f=w1249) -> (s? t:f=w1248:T28)
          n457 = Bundle By Name(cluster=w1252, "VariableName"=w1273, "VariableType"="Circle", "CircleArrayOUT"=w1244) -> (w1257:T14)
          n458 = Bundle By Name(cluster=w1259, "Measurment Type"="circle", "Measurment Name"=w1273, "PointForOverlays.Circle"=w1248) -> (w1258:T12)
          n459 = Unbundle By Name(w1257) -> ("CircleArrayOUT"=w1256:T19)
          n460 = Index Array(array=w1256) -> (element=w1255:T26)  [unwired: 1 in]
          n461 = Unbundle By Name(w1255) -> ()  [unwired: 1 out]
        }
        frame "approximateCircleByarcs", "approximateCircleByPoints" {
          w1329 = T35 {"Point 1"={"X"=0.0, "Y"=0.0}, "Point 2"={"X"=0.0, "Y"=0.0}, "Center (Pixels)"={"X"=0.0, "Y"=0.0}, "Radius (Pixels)"=0.0}  # Circle
          w1332 = T14 {"VariableName"="", "VariableType"="", "Co-sys Reference"={"Base Co-sys Reference"={"Origin"={"X"=0.0, "Y"=0.0}, "Angle (deg)"=0.0, "Axis Reference"=0, "Scale"=0.0}, "New Co-sys Reference"={"Origin"={"X"=0.0, "Y"=0.0}, "Angle (deg)"=0.0, "Axis Reference"=0, "Scale"=0.0}}, "PointArray"=[], "Line Array"=[], "CircleArrayOUT"=[], "TPDetails"={"DistanceInfo"={"X"=0.0, "Y"=0.0, "X'"=0.0, "Y'"=0.0, "DX"=0.0, "DY"=0.0, "Distance Type"=""}, "Feature and Datum details"=[]}, "Value"=[], "Display Name"=0.0, "ROIArray"=[], "Update ROI "=FALSE}  # AlgoOut
          # "Overlay(Done)"
          n462 = Index Array(array=w1334) -> (element=w1335:T42)  [unwired: 1 in]
          n463 = case shown="\"approximateCircleByarcs\"" w1301 {
            tunnel: w1300 -> [w1338 _]
            tunnel: [w1338 w1339] -> w1298
            tunnel: w1299 -> [_ w1340]
            frame "approximateCircleByPoints", Default {
            }
            frame "approximateCircleByarcs" {
              n464 = for {
                tunnel: w1340 -> [w1343] mode=indexing
                tunnel: [w1341] -> w1339 mode=concatenating
                n465 = Unbundle By Name(w1343) -> ("First Edges"=w1342:T15[])
                n466 = for {
                  tunnel: w1342 -> [w1345] mode=indexing
                  tunnel: [w1344] -> w1341 mode=indexing
                  n467 = Unbundle By Name(w1345) -> ("Location (Pixel)"=w1344:cluster{"X":sgl, "Y":sgl})
                }
              }
            }
          }
          n468 = Unbundle By Name(w1335) -> ("Captured Image"=w1317:T3)
          n469 = Array Size(array=w1298) -> (size(s)=w1311:i32)
          n470 = Greater Or Equal?(x=w1311, y=3) -> (x >= y?=w1309:bool)
          n471 = case shown="True" w1309 {
            tunnel: w1337 -> [w1347 w1355]
            tunnel: w1330 -> [_ w1354]
            tunnel: [T29 {"Center"={"X"=nan, "Y"=nan}, "Radius"=nan} ("Circle") w1353] -> w1325
            tunnel: [w1347 w1352] -> w1320
            tunnel: w1317 -> [_ w1351]
            tunnel: w1313 -> [_ _]
            tunnel: w1298 -> [_ w1350]
            tunnel: [i32[] [] ("Indexes of Points Used") w1349] -> w1305
            frame False {
            }
            frame True {
              n472 = call "approximateCircleByPoints.vi"("error in (no error)"=w1355, "PointArray"=w1350, "Enable overlay?"=w1354, "Image in"=w1351) -> ("error out"=w1352:errorcluster, "Indexes of Points Used"=w1349:i32[], "Circle"=w1353:T29)  [unwired: 4 in, 1 out]
            }
          }
          n473 = Unbundle By Name(w1325) -> ("Center"=w1308:cluster{"X":sgl, "Y":sgl}, "Radius"=w1314:dbl)
          n474 = Index Array(array=w1305) -> (element=w1304:i32)  [unwired: 1 in]
          n475 = call "point_within_img.vi"("error in (no error)"=w1320, "Image"=w1317, "Point"=w1308) -> ("error out"=w1319:errorcluster, "Point"=w1318:cluster{"Point X":dbl, "Point Y":dbl})  [unwired: 6 in, 1 out]
          n476 = Index Array(array=w1298, index=w1304) -> (element=w1302:cluster{"X":sgl, "Y":sgl})
          n477 = call "FEATURE_DETECTED.vi"("error in (no error)"=w1319, "Point"=w1318) -> ("error out"=w1322:errorcluster, "s? t:f"=w1307:cluster{"X":dbl, "Y":dbl}, "x .and. y?"=w1316:bool)  [unwired: 7 in]
          n478 = Select(t=nan, s=w1316, f=w1314) -> (s? t:f=w1306:dbl)
          n479 = Bundle By Name(cluster=T26 {"CircleDetected"={"Center (Pixels)"={"X"=0.0, "Y"=0.0}, "Radius (Pixels)"=0.0}, "First Edges"=[], "Indexes of Points Used"=[], "Start Point"={"X"=0.0, "Y"=0.0}, "End Point"={"X"=0.0, "Y"=0.0}} ("Circle Array"), "CircleDetected.Center (Pixels)"=w1307, "CircleDetected.Radius (Pixels)"=w1306, "Start Point"=w1302, "End Point"=w1302) -> (w1324:T26)
          n480 = Bundle By Name(cluster=w1329, "Center (Pixels)"=w1307, "Radius (Pixels)"=w1306, "Point 1"=w1302, "Point 2"=w1302) -> (w1321:T35)
          n481 = Build Array(w1324) -> (w1323:T19)
          n482 = Build Array(w1321) -> (w1328:T28)
          n483 = Build Array(w1307) -> (w1312:cluster{"X":dbl, "Y":dbl}[])
          n484 = Bundle By Name(cluster=w1326, "Measurment Type"="circle", "PointForOverlays.Circle"=w1328, "Measurment Name"=w1313) -> (w1327:T12)
          n485 = Bundle By Name(cluster=w1332, "VariableName"=w1313, "VariableType"="Circle", "CircleArrayOUT"=w1323, "PointArray"=w1312) -> (w1336:T14)
        }
        frame "Detect Outer Circle", "Detect Root Circle" {
          w1377 = T35 {"Point 1"={"X"=0.0, "Y"=0.0}, "Point 2"={"X"=0.0, "Y"=0.0}, "Center (Pixels)"={"X"=0.0, "Y"=0.0}, "Radius (Pixels)"=0.0}  # Circle
          w1392 = T14 {"VariableName"="", "VariableType"="", "Co-sys Reference"={"Base Co-sys Reference"={"Origin"={"X"=0.0, "Y"=0.0}, "Angle (deg)"=0.0, "Axis Reference"=0, "Scale"=0.0}, "New Co-sys Reference"={"Origin"={"X"=0.0, "Y"=0.0}, "Angle (deg)"=0.0, "Axis Reference"=0, "Scale"=0.0}}, "PointArray"=[], "Line Array"=[], "CircleArrayOUT"=[], "TPDetails"={"DistanceInfo"={"X"=0.0, "Y"=0.0, "X'"=0.0, "Y'"=0.0, "DX"=0.0, "DY"=0.0, "Distance Type"=""}, "Feature and Datum details"=[]}, "Value"=[], "Display Name"=0.0, "ROIArray"=[], "Update ROI "=FALSE}  # AlgoOut
          # "Overlay(Done)"
          n486 = Delete From Array(array=w1385, length=1, index=0) -> (deleted portion=w1384:T19, array with subset deleted=w1360:T19)
          n487 = Index Array(array=w1384) -> (element=w1383:T26)  [unwired: 1 in]
          n488 = Unbundle By Name(w1383) -> ("CircleDetected.Center (Pixels)"=w1382:cluster{"X":sgl, "Y":sgl})
          n489 = call "Detect RootOuter Circle.vi"("Circle Array"=w1360, "Calibrated Image"=w1388, "Center (Pixels)"=w1382, "Conversion Factor"=w1381, "error in (no error)"=w1374, "Case name"=w1378, "Conversion Factor/Calibrated Image"=w1380) -> ("Circle Detected"=w1366:T26, "error out"=w1363:errorcluster)  [unwired: 11 in]
          n490 = Unbundle By Name(w1366) -> ("CircleDetected.Center (Pixels)"=w1371:cluster{"X":sgl, "Y":sgl}, "CircleDetected.Radius (Pixels)"=w1368:dbl, "First Edges"=w1367:T15[], "Indexes of Points Used"=w1361:i32[])
          n491 = call "FEATURE_DETECTED.vi"("error in (no error)"=w1363, "Point"=w1371) -> ("error out"=w1373:errorcluster, "x .and. y?"=w1372:bool)  [unwired: 7 in, 1 out]
          n492 = case shown="False" w1372 {
            tunnel: w1371 -> [w1400 _]
            tunnel: [w1400 w1404] -> w1370
            tunnel: [w1402 nan] -> w1369
            tunnel: w1368 -> [w1402 _]
            tunnel: w1367 -> [w1399 _]
            tunnel: w1366 -> [w1401 _]
            tunnel: [w1401 T30 {"CircleDetected"={"Center (Pixels)"={"X"=nan, "Y"=nan}, "Radius (Pixels)"=nan}, "First Edges"=[], "Indexes of Points Used"=[], "Start Point"={"X"=0.0, "Y"=0.0}, "End Point"={"X"=0.0, "Y"=0.0}} ("Circle Array")] -> w1359
            tunnel: [w1400 w1404] -> w1365
            tunnel: [w1397 w1404] -> w1358
            tunnel: [w1397 w1404] -> w1356
            tunnel: w1361 -> [w1396 _]
            frame False {
              n493 = Index Array(array=w1396) -> (element=w1395:i32)  [unwired: 1 in]
              n494 = Index Array(array=w1399, index=w1395) -> (element=w1398:T15)
              n495 = Unbundle By Name(w1398) -> ("Location (Pixel)"=w1397:cluster{"X":sgl, "Y":sgl})
            }
            frame True {
              w1404 = cluster{"X":sgl, "Y":sgl} {"X"=nan, "Y"=nan} ("Center (Pixels)")
            }
          }
          n496 = Build Array(w1365) -> (w1364:cluster{"X":sgl, "Y":sgl}[])
          n497 = Bundle By Name(cluster=w1359, "Start Point"=w1358, "End Point"=w1356) -> (w1357:T30)
          n498 = Bundle By Name(cluster=w1377, "Center (Pixels)"=w1370, "Radius (Pixels)"=w1369, "Point 1"=w1358, "Point 2"=w1356) -> (w1376:T35)
          n499 = Build Array(w1376) -> (w1375:T28)
          n500 = Build Array(w1357) -> (w1379:T27)
          n501 = Bundle By Name(cluster=w1389, "Measurment Type"="circle", "PointForOverlays.Circle"=w1375, "Measurment Name"=w1362) -> (w1390:T12)
          n502 = Bundle By Name(cluster=w1392, "VariableName"=w1362, "VariableType"="Circle", "CircleArrayOUT"=w1379, "PointArray"=w1364) -> (w1394:T14)
        }
        frame "Circumference points" {
          w1420 = T14 {"VariableName"="", "VariableType"="", "Co-sys Reference"={"Base Co-sys Reference"={"Origin"={"X"=0.0, "Y"=0.0}, "Angle (deg)"=0.0, "Axis Reference"=0, "Scale"=0.0}, "New Co-sys Reference"={"Origin"={"X"=0.0, "Y"=0.0}, "Angle (deg)"=0.0, "Axis Reference"=0, "Scale"=0.0}}, "PointArray"=[], "Line Array"=[], "CircleArrayOUT"=[], "TPDetails"={"DistanceInfo"={"X"=0.0, "Y"=0.0, "X'"=0.0, "Y'"=0.0, "DX"=0.0, "DY"=0.0, "Distance Type"=""}, "Feature and Datum details"=[]}, "Value"=[], "Display Name"=0.0, "ROIArray"=[], "Update ROI "=FALSE}  # AlgoOut
          # "Overlay(Done)"
          n503 = Index Array(array=w1422) -> (element=w1423:T42)  [unwired: 1 in]
          n504 = Unbundle By Name(w1417) -> ("ROI"=w1416:T47, "Edge Options"=w1415:T5, "Circle Fit Options"=w1414:T60, "ROI Overlay Enabled"=w1409:bool)
          n505 = Unbundle By Name(w1423) -> ("Captured Image"=w1418:T3)  [unwired: 1 out]
          n506 = call "Circumference points.vi"("Image in"=w1418, "ROI"=w1416, "Edge Options"=w1415, "Circle Fit Options"=w1414, "ROI Overlay Enabled"=w1409, "error in (no error)"=w1419, "group name"=w1407, "Measurement Overlay Enabled"=FALSE) -> ("Circle info"=w1411:T19, "error out"=w1413:errorcluster)  [unwired: 10 in]
          n507 = Empty Array?(array=w1411) -> (empty?=w1410:bool)
          n508 = case shown="False" w1410 {
            tunnel: w1411 -> [w1425 _]
            tunnel: [w1425 w1427] -> w1412
            frame False {
            }
            frame True {
              w1426 = T30 {"CircleDetected"={"Center (Pixels)"={"X"=nan, "Y"=nan}, "Radius (Pixels)"=nan}, "First Edges"=[], "Indexes of Points Used"=[], "Start Point"={"X"=0.0, "Y"=0.0}, "End Point"={"X"=0.0, "Y"=0.0}}  # Circle NaN Array
              n509 = Build Array(w1426) -> (w1427:T27)
            }
          }
          n510 = Bundle By Name(cluster=w1420, "VariableName"=w1407, "VariableType"="Circle", "CircleArrayOUT"=w1412) -> (w1424:T14)
        }
        frame "ArcDetect" {
          w1447 = T62 {"Edge Options"={"Edge Polarity"=0, "Kernel Size"=7, "Width"=7, "Minimum Edge Strength"=75.0, "Interpolation Type"=enum."Bilinear Fixed", "Data Processing Method"=enum."Average"}, "Scan Direction"=0, "Process"=enum."Get All Edges", "Step Size"=1.0}  # Settings
          w1450 = T14 {"VariableName"="", "VariableType"="", "Co-sys Reference"={"Base Co-sys Reference"={"Origin"={"X"=0.0, "Y"=0.0}, "Angle (deg)"=0.0, "Axis Reference"=0, "Scale"=0.0}, "New Co-sys Reference"={"Origin"={"X"=0.0, "Y"=0.0}, "Angle (deg)"=0.0, "Axis Reference"=0, "Scale"=0.0}}, "PointArray"=[], "Line Array"=[], "CircleArrayOUT"=[], "TPDetails"={"DistanceInfo"={"X"=0.0, "Y"=0.0, "X'"=0.0, "Y'"=0.0, "DX"=0.0, "DY"=0.0, "Distance Type"=""}, "Feature and Datum details"=[]}, "Value"=[], "Display Name"=0.0, "ROIArray"=[], "Update ROI "=FALSE}  # AlgoOut
          # "Overlay(Done)"
          n511 = Unbundle By Name(w1449) -> ("ROI"=w1431:T47, "ROI Overlay Enabled"=w1430:bool, "Edge Options"=w1446:T5, "Search Direction"=w1441:u16, "Process"=w1440:u16, "Circle Fit Options.Step Size"=w1442:dbl)
          n512 = Index Array(array=w1452) -> (element=w1453:T42)  [unwired: 1 in]
          n513 = Unbundle By Name(w1453) -> ("Captured Image"=w1433:T3)  [unwired: 1 out]
          n514 = Bundle By Name(cluster=w1447, "Edge Options"=w1446, "Scan Direction"=w1441, "Process"=w1440, "Step Size"=w1442) -> (w1443:T62)
          n515 = case shown="True" w1430 {
            tunnel: [w1455 w1457] -> w1432
            tunnel: w1433 -> [w1455 w1458]
            tunnel: w1431 -> [_ w1456]
            frame False {
            }
            frame True {
              n516 = call "IMAQ Overlay ROI"("ROI Descriptor"=w1456, "Image"=w1458) -> ("Image Out"=w1457:T3)  [unwired: 8 in, 1 out]
            }
          }
          n517 = call "Arc Detect.vi"("Image Out"=w1432, "ROI Descriptor"=w1431, "Settings"=w1443, "error in (no error)"=w1448) -> ("Circle Details"=w1445:T27, "Points"=w1428:cluster{"X":sgl, "Y":sgl}[], "error out"=w1444:errorcluster)  [unwired: 13 in]
          n518 = Empty Array?(array=w1445) -> (empty?=w1429:bool)
          n519 = case shown="False" w1429 {
            tunnel: w1445 -> [w1460 _]
            tunnel: [w1460 w1462] -> w1439
            tunnel: w1428 -> [w1459 _]
            tunnel: [w1459 cluster{"X":sgl, "Y":sgl}[] [{"X"=nan, "Y"=nan}] ("Points")] -> w1435
            frame False {
            }
            frame True {
              w1463 = T30 {"CircleDetected"={"Center (Pixels)"={"X"=nan, "Y"=nan}, "Radius (Pixels)"=nan}, "First Edges"=[], "Indexes of Points Used"=[], "Start Point"={"X"=0.0, "Y"=0.0}, "End Point"={"X"=0.0, "Y"=0.0}}  # Circle NaN Array
              n520 = Build Array(w1463) -> (w1462:T27)
            }
          }
          n521 = Bundle By Name(cluster=w1438, "Measurment Name"=w1436, "Measurment Type"="Point", "PointForOverlays.Points.Points"=w1435) -> (w1437:T12)
          n522 = Bundle By Name(cluster=w1450, "VariableName"=w1436, "VariableType"="Circle", "CircleArrayOUT"=w1439, "PointArray"=w1435) -> (w1454:T14)
        }
        frame "intermediateCircle" {
          w1465 = T26 {"CircleDetected"={"Center (Pixels)"={"X"=0.0, "Y"=0.0}, "Radius (Pixels)"=0.0}, "First Edges"=[], "Indexes of Points Used"=[], "Start Point"={"X"=0.0, "Y"=0.0}, "End Point"={"X"=0.0, "Y"=0.0}}  # Circle Array
          w1481 = T35 {"Point 1"={"X"=0.0, "Y"=0.0}, "Point 2"={"X"=0.0, "Y"=0.0}, "Center (Pixels)"={"X"=0.0, "Y"=0.0}, "Radius (Pixels)"=0.0}  # Circle
          w1490 = T14 {"VariableName"="", "VariableType"="", "Co-sys Reference"={"Base Co-sys Reference"={"Origin"={"X"=0.0, "Y"=0.0}, "Angle (deg)"=0.0, "Axis Reference"=0, "Scale"=0.0}, "New Co-sys Reference"={"Origin"={"X"=0.0, "Y"=0.0}, "Angle (deg)"=0.0, "Axis Reference"=0, "Scale"=0.0}}, "PointArray"=[], "Line Array"=[], "CircleArrayOUT"=[], "TPDetails"={"DistanceInfo"={"X"=0.0, "Y"=0.0, "X'"=0.0, "Y'"=0.0, "DX"=0.0, "DY"=0.0, "Distance Type"=""}, "Feature and Datum details"=[]}, "Value"=[], "Display Name"=0.0, "ROIArray"=[], "Update ROI "=FALSE}  # AlgoOut
          # "newly added"
          n523 = Index Array(array=w1487) -> (element=w1488:T42)  [unwired: 1 in]
          n524 = Index Array(array=w1469) -> (element #1=w1475:T26, element #2=w1474:T26)  [unwired: 2 in]
          n525 = Array Size(array=w1469) -> (size(s)=w1468:i32)
          n526 = Unbundle By Name(w1488) -> ("Captured Image"=w1484:T3)
          n527 = Unbundle By Name(w1475) -> ("CircleDetected"=w1471:T48)
          n528 = Unbundle By Name(w1474) -> ("CircleDetected"=w1470:T48)
          n529 = Equal?(x=w1468, y=2) -> (x = y?=w1464:bool)
          n530 = case shown="True" w1464 {
            tunnel: w1486 -> [w1495 w1502]
            tunnel: w1484 -> [_ w1501]
            tunnel: w1483 -> [_ w1500]
            tunnel: [w1495 w1499] -> w1479
            tunnel: [T29 {"Center"={"X"=nan, "Y"=nan}, "Radius"=nan} ("intermediateCircle") w1498] -> w1473
            tunnel: w1471 -> [_ w1497]
            tunnel: w1470 -> [_ w1496]
            frame False {
            }
            frame True {
              n531 = call "intermediateCircle.vi"("measurement overlay enabled"=w1500, "error in (no error)"=w1502, "Circle_2"=w1496, "Circle_1"=w1497, "Image"=w1501) -> ("error out"=w1499:errorcluster, "intermediateCircle"=w1498:T29)  [unwired: 4 in, 1 out]
            }
          }
          n532 = Unbundle By Name(w1473) -> ("Center"=w1478:cluster{"X":sgl, "Y":sgl}, "Radius"=w1480:dbl)
          n533 = Bundle By Name(cluster=w1481, "Center (Pixels)"=w1478, "Radius (Pixels)"=w1480) -> (w1491:T35)
          n534 = Bundle By Name(cluster=w1465, "CircleDetected"=w1473) -> (w1472:T26)
          n535 = Build Array(w1491) -> (w1482:T28)
          n536 = Build Array(w1472) -> (w1466:T19)
          n537 = Bundle By Name(cluster=w1477, "Measurment Type"="circle", "Measurment Name"=w1489, "PointForOverlays.Circle"=w1482) -> (w1476:T12)
          n538 = Bundle By Name(cluster=w1490, "VariableName"=w1489, "VariableType"="Circle", "CircleArrayOUT"=w1466) -> (w1492:T14)
        }
        frame "AuxiliaryCircle" {
          w1521 = T26 {"CircleDetected"={"Center (Pixels)"={"X"=0.0, "Y"=0.0}, "Radius (Pixels)"=0.0}, "First Edges"=[], "Indexes of Points Used"=[], "Start Point"={"X"=0.0, "Y"=0.0}, "End Point"={"X"=0.0, "Y"=0.0}}  # Circle Info
          w1524 = T35 {"Point 1"={"X"=0.0, "Y"=0.0}, "Point 2"={"X"=0.0, "Y"=0.0}, "Center (Pixels)"={"X"=0.0, "Y"=0.0}, "Radius (Pixels)"=0.0}  # Overlay Circle
          w1533 = T14 {"VariableName"="", "VariableType"="", "Co-sys Reference"={"Base Co-sys Reference"={"Origin"={"X"=0.0, "Y"=0.0}, "Angle (deg)"=0.0, "Axis Reference"=0, "Scale"=0.0}, "New Co-sys Reference"={"Origin"={"X"=0.0, "Y"=0.0}, "Angle (deg)"=0.0, "Axis Reference"=0, "Scale"=0.0}}, "PointArray"=[], "Line Array"=[], "CircleArrayOUT"=[], "TPDetails"={"DistanceInfo"={"X"=0.0, "Y"=0.0, "X'"=0.0, "Y'"=0.0, "DX"=0.0, "DY"=0.0, "Distance Type"=""}, "Feature and Datum details"=[]}, "Value"=[], "Display Name"=0.0, "ROIArray"=[], "Update ROI "=FALSE}  # AlgoOut
          # "newly added"
          n539 = Array Size(array=w1506) -> (size(s)=w1507:i32)
          n540 = Decrement(x=w1507) -> (x-1=w1505:i32)
          n541 = Unbundle By Name(w1527) -> ("Width"=w1526:i32, "Height"=w1525:i32)
          n542 = Index Array "Indexing Value Array"(array=w1506, index=w1505) -> (element=w1528:sgl)
          n543 = Index Array "Indexing Point Array"(array=w1513) -> (element=w1512:cluster{"X":sgl, "Y":sgl})  [unwired: 1 in]
          n544 = call "AuxiliaryCircle.vi"("centre of circle"=w1512, "Dia in mm"=w1528, "X Resolution"=w1526, "Y Resolution"=w1525, "conversion factor"=w1529, "error in"=w1530) -> ("centre of circle"=w1504:cluster{"centre x":dbl, "centre y":dbl}, "Radius in pixel"=w1509:dbl, "error out"=w1515:errorcluster)  [unwired: 11 in]
          n545 = Unbundle By Name(w1504) -> ("centre x"=w1510:dbl)
          n546 = Add(x=w1510, y=w1509) -> (x+y=w1511:dbl)
          n547 = Bundle By Name(cluster=w1504, "centre x"=w1511) -> (w1508:cluster{"centre x":dbl, "centre y":dbl})
          n548 = Bundle By Name(cluster=w1524, "Center (Pixels)"=w1504, "Radius (Pixels)"=w1509, "Point 1"=w1508, "Point 2"=w1508) -> (w1523:T35)
          n549 = Bundle By Name(cluster=w1521, "CircleDetected.Center (Pixels)"=w1504, "CircleDetected.Radius (Pixels)"=w1509) -> (w1520:T26)
          n550 = Build Array(w1523) -> (w1522:T28)
          n551 = Build Array(w1520) -> (w1519:T19)
          n552 = Build Array(w1504) -> (w1514:cluster{"centre x":dbl, "centre y":dbl}[])
          n553 = Bundle By Name(cluster=w1531, "Measurment Type"="Circle", "Measurment Name"=w1503, "PointForOverlays.Circle"=w1522) -> (w1532:T12)
          n554 = Bundle By Name(cluster=w1533, "VariableName"=w1503, "VariableType"="Circle", "CircleArrayOUT"=w1519, "PointArray"=w1514) -> (w1516:T14)
        }
        frame "AutoCenteringInternal" {
          w1548 = T26 {"CircleDetected"={"Center (Pixels)"={"X"=0.0, "Y"=0.0}, "Radius (Pixels)"=0.0}, "First Edges"=[], "Indexes of Points Used"=[], "Start Point"={"X"=0.0, "Y"=0.0}, "End Point"={"X"=0.0, "Y"=0.0}}  # Circle Info
          w1550 = T35 {"Point 1"={"X"=0.0, "Y"=0.0}, "Point 2"={"X"=0.0, "Y"=0.0}, "Center (Pixels)"={"X"=0.0, "Y"=0.0}, "Radius (Pixels)"=0.0}  # Overlay Circle
          w1566 = "Circle" ("VariableType")
          w1569 = T14 {"VariableName"="", "VariableType"="", "Co-sys Reference"={"Base Co-sys Reference"={"Origin"={"X"=0.0, "Y"=0.0}, "Angle (deg)"=0.0, "Axis Reference"=0, "Scale"=0.0}, "New Co-sys Reference"={"Origin"={"X"=0.0, "Y"=0.0}, "Angle (deg)"=0.0, "Axis Reference"=0, "Scale"=0.0}}, "PointArray"=[], "Line Array"=[], "CircleArrayOUT"=[], "TPDetails"={"DistanceInfo"={"X"=0.0, "Y"=0.0, "X'"=0.0, "Y'"=0.0, "DX"=0.0, "DY"=0.0, "Distance Type"=""}, "Feature and Datum details"=[]}, "Value"=[], "Display Name"=0.0, "ROIArray"=[], "Update ROI "=FALSE}  # AlgoOut
          # "Coertion Dot because of Enum to Integer Difference"
          n555 = Index Array(array=w1571) -> (element=w1570:T42)  [unwired: 1 in]
          n556 = Array Size(array=w1535) -> (size(s)=w1536:i32)
          n557 = Index Array(array=w1553) -> (element=w1552:T26)  [unwired: 1 in]
          n558 = Unbundle By Name(w1572) -> ("ROI"=w1560:T47, "Edge Options"=w1559:T5, "Line Options.Step Size"=w1558:u32)
          n559 = Unbundle By Name(w1570) -> ("Captured Image"=w1563:T3)
          n560 = Decrement(x=w1536) -> (x-1=w1534:i32)
          n561 = Unbundle By Name(w1552) -> ("CircleDetected.Center (Pixels)"=w1551:cluster{"X":sgl, "Y":sgl})
          n562 = Index Array(array=w1535, index=w1534) -> (element=w1554:sgl)
          n563 = case shown="True" w1562 {
            tunnel: w1560 -> [_ w1576]
            tunnel: w1563 -> [w1573 w1575]
            tunnel: [w1573 w1574] -> w1561
            frame False {
            }
            frame True {
              n564 = call "IMAQ Overlay ROI"("ROI Descriptor"=w1576, "Image"=w1575) -> ("Image Out"=w1574:T3)  [unwired: 8 in, 1 out]
            }
          }
          n565 = call "auto center internal.vi"("Image In"=w1561, "Annular ROI"=w1560, "Edge Options"=w1559, "Step Size"=w1558, "Refenerence circle Center"=w1551, "dia in mm"=w1554, "Conversioin factor"=w1557, "error in (no error)"=w1538, "Conversion Factor Y/N"=w1556, "calib image"=w1555) -> ("centre"=w1541:cluster{"X":dbl, "Y":dbl}, "Radius"=w1540:dbl, "error out"=w1539:errorcluster)  [unwired: 15 in]
          n566 = Unbundle By Name(w1541) -> ("X"=w1545:dbl)
          n567 = Add(x=w1545, y=w1540) -> (x+y=w1546:dbl)
          n568 = Bundle By Name(cluster=w1541, "X"=w1546) -> (w1544:cluster{"X":dbl, "Y":dbl})
          n569 = Bundle By Name(cluster=w1548, "CircleDetected.Center (Pixels)"=w1541, "CircleDetected.Radius (Pixels)"=w1540) -> (w1547:T26)
          n570 = Bundle By Name(cluster=w1550, "Center (Pixels)"=w1541, "Radius (Pixels)"=w1540, "Point 1"=w1544, "Point 2"=w1544) -> (w1549:T35)
          n571 = Build Array(w1547) -> (w1542:T19)
          n572 = Build Array(w1541) -> (w1537:cluster{"X":dbl, "Y":dbl}[])
          n573 = Build Array(w1549) -> (w1543:T28)
          n574 = Bundle By Name(cluster=w1567, "Measurment Name"=w1564, "PointForOverlays.Circle"=w1543, "Measurment Type"=w1566) -> (w1565:T12)
          n575 = Bundle By Name(cluster=w1569, "VariableName"=w1564, "VariableType"=w1566, "CircleArrayOUT"=w1542, "PointArray"=w1537) -> (w1568:T14)
        }
        frame "CurvePeakPoint" {
          w1594 = "Point" ("VariableType")
          w1597 = T14 {"VariableName"="", "VariableType"="", "Co-sys Reference"={"Base Co-sys Reference"={"Origin"={"X"=0.0, "Y"=0.0}, "Angle (deg)"=0.0, "Axis Reference"=0, "Scale"=0.0}, "New Co-sys Reference"={"Origin"={"X"=0.0, "Y"=0.0}, "Angle (deg)"=0.0, "Axis Reference"=0, "Scale"=0.0}}, "PointArray"=[], "Line Array"=[], "CircleArrayOUT"=[], "TPDetails"={"DistanceInfo"={"X"=0.0, "Y"=0.0, "X'"=0.0, "Y'"=0.0, "DX"=0.0, "DY"=0.0, "Distance Type"=""}, "Feature and Datum details"=[]}, "Value"=[], "Display Name"=0.0, "ROIArray"=[], "Update ROI "=FALSE}  # AlgoOut
          # "Coertion Dot because of Enum to Integer Difference"
          n576 = Index Array(array=w1599) -> (element=w1598:T42)  [unwired: 1 in]
          n577 = Index Array(array=w1586) -> (element=w1589:T23)  [unwired: 1 in]
          n578 = Unbundle By Name(w1600) -> ("ROI"=w1587:T47, "Edge Options"=w1578:T5, "Process"=w1577:u16, "Line Options.Step Size"=w1584:u32, "Search Direction"=w1583:u16)
          n579 = Unbundle By Name(w1598) -> ("Captured Image"=w1591:T3)
          n580 = Unbundle By Name(w1589) -> ("Line"=w1585:T24)
          n581 = case shown="True" w1590 {
            tunnel: w1587 -> [_ w1604]
            tunnel: w1591 -> [w1601 w1603]
            tunnel: [w1601 w1602] -> w1588
            frame False {
            }
            frame True {
              n582 = call "IMAQ Overlay ROI"("ROI Descriptor"=w1604, "Image"=w1603) -> ("Image Out"=w1602:T3)  [unwired: 8 in, 1 out]
            }
          }
          n583 = call "PeakPointDetection.vi"("Image"=w1588, "ROI"=w1587, "Reference Line"=w1585, "Step Size"=w1584, "Search Direction"=w1583, "error in (no error)"=w1582, "Process"=w1577, "Edge Options"=w1578) -> ("Peak Point"=w1580:cluster{"X":sgl, "Y":sgl}, "error IO"=w1581:errorcluster)  [unwired: 9 in, 1 out]
          n584 = Build Array(w1580) -> (w1579:cluster{"X":sgl, "Y":sgl}[])
          n585 = Bundle By Name(cluster=w1595, "Measurment Name"=w1592, "PointForOverlays.Points.Points"=w1579, "Measurment Type"=w1594) -> (w1593:T12)
          n586 = Bundle By Name(cluster=w1597, "VariableName"=w1592, "VariableType"=w1594, "PointArray"=w1579) -> (w1596:T14)
        }
        frame "AutoCenteringExternal" {
          w1626 = T26 {"CircleDetected"={"Center (Pixels)"={"X"=0.0, "Y"=0.0}, "Radius (Pixels)"=0.0}, "First Edges"=[], "Indexes of Points Used"=[], "Start Point"={"X"=0.0, "Y"=0.0}, "End Point"={"X"=0.0, "Y"=0.0}}  # Circle Info
          w1628 = T35 {"Point 1"={"X"=0.0, "Y"=0.0}, "Point 2"={"X"=0.0, "Y"=0.0}, "Center (Pixels)"={"X"=0.0, "Y"=0.0}, "Radius (Pixels)"=0.0}  # Overlay Circle
          w1635 = "Circle" ("VariableType")
          w1638 = T14 {"VariableName"="", "VariableType"="", "Co-sys Reference"={"Base Co-sys Reference"={"Origin"={"X"=0.0, "Y"=0.0}, "Angle (deg)"=0.0, "Axis Reference"=0, "Scale"=0.0}, "New Co-sys Reference"={"Origin"={"X"=0.0, "Y"=0.0}, "Angle (deg)"=0.0, "Axis Reference"=0, "Scale"=0.0}}, "PointArray"=[], "Line Array"=[], "CircleArrayOUT"=[], "TPDetails"={"DistanceInfo"={"X"=0.0, "Y"=0.0, "X'"=0.0, "Y'"=0.0, "DX"=0.0, "DY"=0.0, "Distance Type"=""}, "Feature and Datum details"=[]}, "Value"=[], "Display Name"=0.0, "ROIArray"=[], "Update ROI "=FALSE}  # AlgoOut
          # "Coertion Dot because of Enum to Integer Difference"
          n587 = Index Array(array=w1640) -> (element=w1639:T42)  [unwired: 1 in]
          n588 = Array Size(array=w1605) -> (size(s)=w1607:i32)
          n589 = Index Array(array=w1630) -> (element=w1629:T26)  [unwired: 1 in]
          n590 = Unbundle By Name(w1641) -> ("ROI"=w1617:T47, "Edge Options"=w1616:T5, "Line Options.Step Size"=w1615:u32)
          n591 = Unbundle By Name(w1639) -> ("Captured Image"=w1632:T3)
          n592 = Decrement(x=w1607) -> (x-1=w1606:i32)
          n593 = Unbundle By Name(w1629) -> ("CircleDetected.Center (Pixels)"=w1614:cluster{"X":sgl, "Y":sgl})
          n594 = Index Array(array=w1605, index=w1606) -> (element=w1613:sgl)
          n595 = case shown="True" w1631 {
            tunnel: w1617 -> [_ w1645]
            tunnel: w1632 -> [w1642 w1644]
            tunnel: [w1642 w1643] -> w1618
            frame False {
            }
            frame True {
              n596 = call "IMAQ Overlay ROI"("ROI Descriptor"=w1645, "Image"=w1644) -> ("Image Out"=w1643:T3)  [unwired: 8 in, 1 out]
            }
          }
          n597 = call "auto center external.vi"("Image In"=w1618, "Annular ROI"=w1617, "Edge Options"=w1616, "Step Size"=w1615, "Refenerence circle Center"=w1614, "dia in mm"=w1613, "Conversioin factor"=w1612, "error in (no error)"=w1611) -> ("centre"=w1609:cluster{"X":dbl, "Y":dbl}, "Radius"=w1610:dbl, "error out"=w1608:errorcluster)  [unwired: 17 in]
          n598 = Unbundle By Name(w1609) -> ("X"=w1623:dbl)
          n599 = Add(x=w1623, y=w1610) -> (x+y=w1624:dbl)
          n600 = Bundle By Name(cluster=w1609, "X"=w1624) -> (w1622:cluster{"X":dbl, "Y":dbl})
          n601 = Bundle By Name(cluster=w1626, "CircleDetected.Center (Pixels)"=w1609, "CircleDetected.Radius (Pixels)"=w1610) -> (w1625:T26)
          n602 = Bundle By Name(cluster=w1628, "Center (Pixels)"=w1609, "Radius (Pixels)"=w1610, "Point 1"=w1622, "Point 2"=w1622) -> (w1627:T35)
          n603 = Build Array(w1625) -> (w1620:T19)
          n604 = Build Array(w1609) -> (w1619:cluster{"X":dbl, "Y":dbl}[])
          n605 = Build Array(w1627) -> (w1621:T28)
          n606 = Bundle By Name(cluster=w1636, "Measurment Name"=w1633, "PointForOverlays.Circle"=w1621, "Measurment Type"=w1635) -> (w1634:T12)
          n607 = Bundle By Name(cluster=w1638, "VariableName"=w1633, "VariableType"=w1635, "CircleArrayOUT"=w1620, "PointArray"=w1619) -> (w1637:T14)
        }
        frame "----distance measurements----" {
        }
        frame "pointToPoint" {
          w1664 = T14 {"VariableName"="", "VariableType"="", "Co-sys Reference"={"Base Co-sys Reference"={"Origin"={"X"=0.0, "Y"=0.0}, "Angle (deg)"=0.0, "Axis Reference"=0, "Scale"=0.0}, "New Co-sys Reference"={"Origin"={"X"=0.0, "Y"=0.0}, "Angle (deg)"=0.0, "Axis Reference"=0, "Scale"=0.0}}, "PointArray"=[], "Line Array"=[], "CircleArrayOUT"=[], "TPDetails"={"DistanceInfo"={"X"=0.0, "Y"=0.0, "X'"=0.0, "Y'"=0.0, "DX"=0.0, "DY"=0.0, "Distance Type"=""}, "Feature and Datum details"=[]}, "Value"=[], "Display Name"=0.0, "ROIArray"=[], "Update ROI "=FALSE}  # AlgoOut
          # "Overlay(Done)"
          # "finds the point to point distance of the two given points"
          n608 = Index Array(array=w1659) -> (element #1=w1656:cluster{"X":sgl, "Y":sgl}, element #2=w1655:cluster{"X":sgl, "Y":sgl})  [unwired: 2 in]
          n609 = Array Size(array=w1659) -> (size(s)=w1658:i32)
          n610 = Greater Or Equal?(x=w1658, y=2) -> (x >= y?=w1649:bool)
          n611 = call "pointToPoint.vi"("error in (no error)"=w1674, "Point2"=w1655, "Point1"=w1656) -> ("error out"=w1672:errorcluster, "lineOUT"=w1660:T32)  [unwired: 6 in, 1 out]
          n612 = Unbundle By Name(w1660) -> ("Point1 (Pixels)"=w1663:cluster{"X":sgl, "Y":sgl}, "Point2 (Pixels)"=w1662:cluster{"X":sgl, "Y":sgl})
          n613 = Not Equal?(x=w1656, y=w1655) -> (x != y?=w1654:cluster{"X":bool, "Y":bool})
          n614 = Unbundle By Name(w1654) -> ("X"=w1653:bool, "Y"=w1652:bool)
          n615 = case shown="\"Measure\"" w1665 {
            tunnel: [w1678 w1691 w1733] -> w1673
            tunnel: w1672 -> [w1677 w1695 w1731]
            tunnel: w1671 -> [_ _ w1730]
            tunnel: w1661 -> [_ w1693 w1728]
            tunnel: [w1677 w1695 w1727] -> w1651
            tunnel: w1663 -> [_ w1686 w1715]
            tunnel: w1662 -> [_ w1685 w1714]
            tunnel: w1669 -> [_ _ w1726]
            tunnel: w1668 -> [_ _ w1725]
            tunnel: w1664 -> [w1678 w1694 w1724]
            tunnel: w1659 -> [_ _ w1721]
            tunnel: w1653 -> [_ w1689 _]
            tunnel: w1652 -> [_ w1688 _]
            tunnel: [cluster{"X":sgl, "Y":sgl}[] [] ("PointForOverlays.Points.Points") cluster{"X":sgl, "Y":sgl}[] [] ("PointForOverlays.Points.Points") w1713] -> w1650
            tunnel: [T31 [] ("Line") w1679 T31 [] ("Line")] -> w1648
            tunnel: w1649 -> [_ w1680 _]
            frame Default {
            }
            frame "Detect" {
              n616 = Compound Arithmetic op=OR(w1689, w1688) -> (w1684:bool)
              n617 = And(x=w1684, y=w1680) -> (x .and. y?=w1683:bool)
              n618 = case shown="True" w1683 {
                tunnel: w1686 -> [_ w1701]
                tunnel: w1685 -> [_ w1702]
                tunnel: [w1699 w1706] -> w1687
                tunnel: [w1698 w1703] -> w1681
                frame False {
                  w1697 = cluster{"X":sgl, "Y":sgl} {"X"=nan, "Y"=nan} ("Line.Point 1")
                  n619 = Bundle By Name(cluster=T23 {"Line"={"Point 1"={"X"=0.0, "Y"=0.0}, "Point 2"={"X"=0.0, "Y"=0.0}}, "Straight Edges"=[], "Used Edges"=[]} ("Line"), "Line.Point 1"=w1697, "Line.Point 2"=w1697) -> (w1699:T23)
                  n620 = Bundle By Name(cluster=T24 {"Point 1"={"X"=0.0, "Y"=0.0}, "Point 2"={"X"=0.0, "Y"=0.0}} ("Line"), "Point 1"=w1697, "Point 2"=w1697) -> (w1698:T24)
                }
                frame True {
                  n621 = Bundle By Name(cluster=T23 {"Line"={"Point 1"={"X"=0.0, "Y"=0.0}, "Point 2"={"X"=0.0, "Y"=0.0}}, "Straight Edges"=[], "Used Edges"=[]} ("Line"), "Line.Point 1"=w1701, "Line.Point 2"=w1702) -> (w1706:T23)
                  n622 = Bundle By Name(cluster=T24 {"Point 1"={"X"=0.0, "Y"=0.0}, "Point 2"={"X"=0.0, "Y"=0.0}} ("Line"), "Point 2"=w1702, "Point 1"=w1701) -> (w1703:T24)
                }
              }
              n623 = Build Array(w1687) -> (w1690:T18)
              n624 = Bundle By Name(cluster=w1694, "VariableName"=w1693, "VariableType"="Line", "Line Array"=w1690) -> (w1691:T14)
              n625 = Build Array(w1681) -> (w1679:T31)
            }
            frame "Measure" {
              n626 = case shown="False" w1726 {
                tunnel: [w1747 w1754] -> w1732
                tunnel: w1731 -> [w1746 w1754]
                tunnel: w1730 -> [w1744 _]
                tunnel: [w1743 w1748] -> w1729
                tunnel: w1715 -> [w1742 w1753]
                tunnel: w1714 -> [w1741 w1752]
                tunnel: w1725 -> [_ w1751]
                frame False {
                  n627 = Build Array(w1742, w1741) -> (w1745:cluster{"X":sgl, "Y":sgl}[])
                  n628 = call "IMAQ Convert Pixel to Real World"("error in (no error)"=w1746, "Array of Pixel Coordinates"=w1745, "Calibrated Image"=w1744) -> ("error out"=w1747:errorcluster, "Array of Real World Coordinates"=w1743:cluster{"X":sgl, "Y":sgl}[])  [unwired: 3 in, 4 out]
                }
                frame True {
                  n629 = Divide(x=w1753, y=w1751) -> (x/y=w1750:cluster{"X":dbl, "Y":dbl})
                  n630 = Divide(x=w1752, y=w1751) -> (x/y=w1749:cluster{"X":dbl, "Y":dbl})
                  n631 = Build Array(w1750, w1749) -> (w1748:cluster{"X":dbl, "Y":dbl}[])
                }
              }
              n632 = call "IMAQ Point Distances"("Points"=w1729, "error in (no error)"=w1732) -> ("Distances"=w1710:sgl[], "error out"=w1727:errorcluster)  [unwired: 3 in]
              n633 = Index Array(array=w1721) -> (element #1=w1720:cluster{"X":sgl, "Y":sgl}, element #2=w1719:cluster{"X":sgl, "Y":sgl})  [unwired: 2 in]
              n634 = Array Size(array=w1721) -> (size(s)=w1723:i32)
              n635 = Not Equal?(x=w1720, y=w1719) -> (x != y?=w1718:cluster{"X":bool, "Y":bool})
              n636 = Unbundle By Name(w1718) -> ("X"=w1717:bool, "Y"=w1716:bool)
              n637 = Equal?(x=w1723, y=2) -> (x = y?=w1712:bool)
              n638 = Compound Arithmetic op=OR(w1717, w1716) -> (w1711:bool)
              n639 = And(x=w1712, y=w1711) -> (x .and. y?=w1709:bool)
              n640 = case shown="True" w1709 {
                tunnel: w1715 -> [_ w1740]
                tunnel: w1714 -> [_ w1739]
                tunnel: [cluster{"X":sgl, "Y":sgl}[] [{"X"=nan, "Y"=nan}] ("PointForOverlays.Points.Points") w1738] -> w1713
                tunnel: [sgl[] [nan] ("Distances") w1737] -> w1708
                tunnel: w1710 -> [_ w1737]
                frame False {
                }
                frame True {
                  n641 = Build Array(w1740, w1739) -> (w1738:cluster{"X":sgl, "Y":sgl}[])
                }
              }
              n642 = Bundle By Name(cluster=w1724, "VariableName"=w1728, "VariableType"="Value", "Value"=w1708) -> (w1733:T14)
            }
          }
          n643 = Bundle By Name(cluster=w1667, "Measurment Type"="lineSeg", "Measurment Name"=w1661, "PointForOverlays.Line"=w1648, "PointForOverlays.Points.Points"=w1650) -> (w1666:T12)
        }
        frame "pointToCircle" {
          w1770 = 1 ("y")
          w1793 = T14 {"VariableName"="", "VariableType"="", "Co-sys Reference"={"Base Co-sys Reference"={"Origin"={"X"=0.0, "Y"=0.0}, "Angle (deg)"=0.0, "Axis Reference"=0, "Scale"=0.0}, "New Co-sys Reference"={"Origin"={"X"=0.0, "Y"=0.0}, "Angle (deg)"=0.0, "Axis Reference"=0, "Scale"=0.0}}, "PointArray"=[], "Line Array"=[], "CircleArrayOUT"=[], "TPDetails"={"DistanceInfo"={"X"=0.0, "Y"=0.0, "X'"=0.0, "Y'"=0.0, "DX"=0.0, "DY"=0.0, "Distance Type"=""}, "Feature and Datum details"=[]}, "Value"=[], "Display Name"=0.0, "ROIArray"=[], "Update ROI "=FALSE}  # AlgoOut
          # "finds the distance between the point and the circle center"
          n644 = Array Size(array=w1757) -> (size(s)=w1756:i32)
          n645 = Index Array(array=w1787) -> (element=w1788:T42)  [unwired: 1 in]
          n646 = Index Array(array=w1773) -> (element=w1776:T26)  [unwired: 1 in]
          n647 = Index Array(array=w1774) -> (element=w1766:cluster{"X":sgl, "Y":sgl})  [unwired: 1 in]
          n648 = Decrement(x=w1756) -> (x-1=w1755:i32)
          n649 = Array Size(array=w1774) -> (size(s)=w1772:i32)
          n650 = Array Size(array=w1773) -> (size(s)=w1771:i32)
          n651 = Index Array(array=w1757, index=w1755) -> (element=w1763:sgl)
          n652 = Unbundle By Name(w1788) -> ("Captured Image"=w1775:T3)
          n653 = Unbundle By Name(w1776) -> ("CircleDetected.Center (Pixels)"=w1765:cluster{"X":sgl, "Y":sgl})
          n654 = Greater Or Equal?(x=w1772, y=w1770) -> (x >= y?=w1769:bool)
          n655 = Greater Or Equal?(x=w1771, y=w1770) -> (x >= y?=w1768:bool)
          n656 = And(x=w1769, y=w1768) -> (x .and. y?=w1764:bool)
          n657 = case shown="True" w1764 {
            tunnel: w1766 -> [_ w1803]
            tunnel: w1765 -> [_ w1802]
            tunnel: [cluster{"X":sgl, "Y":sgl}[] [{"X"=nan, "Y"=nan}] w1804] -> w1758
            tunnel: w1763 -> [_ w1801]
            tunnel: [w1795 w1800] -> w1762
            tunnel: [w1795 w1799] -> w1761
            tunnel: [w1794 w1797] -> w1760
            tunnel: w1759 -> [w1794 w1797]
            frame False {
              w1795 = cluster{"X":sgl, "Y":sgl} {"X"=nan, "Y"=nan} ("Extended Point 2")
            }
            frame True {
              n658 = call "CircleExtendedDistanceFinding.vi"("Value 2"=w1801, "Value 1"=0.0, "Point 2"=w1802, "Point 1"=w1803) -> ("Extended Point 2"=w1799:cluster{"X":sgl, "Y":sgl}, "Extended Point 1"=w1800:cluster{"X":sgl, "Y":sgl})  [unwired: 5 in, 1 out]
              n659 = Build Array(w1800, w1799) -> (w1804:cluster{"X":sgl, "Y":sgl}[])
            }
          }
          n660 = case shown="True" w1780 {
            tunnel: [w1811 w1818] -> w1791
            tunnel: [w1810 w1812] -> w1790
            tunnel: w1760 -> [w1809 w1818]
            tunnel: w1789 -> [w1807 _]
            tunnel: w1761 -> [w1806 w1816]
            tunnel: w1762 -> [w1805 w1817]
            tunnel: w1779 -> [_ w1815]
            frame False {
              n661 = Build Array(w1805, w1806) -> (w1808:cluster{"X":sgl, "Y":sgl}[])
              n662 = call "IMAQ Convert Pixel to Real World"("error in (no error)"=w1809, "Array of Pixel Coordinates"=w1808, "Calibrated Image"=w1807) -> ("error out"=w1811:errorcluster, "Array of Real World Coordinates"=w1810:cluster{"X":sgl, "Y":sgl}[])  [unwired: 3 in, 4 out]
            }
            frame True {
              n663 = Divide(x=w1817, y=w1815) -> (x/y=w1814:cluster{"X":dbl, "Y":dbl})
              n664 = Divide(x=w1816, y=w1815) -> (x/y=w1813:cluster{"X":dbl, "Y":dbl})
              n665 = Build Array(w1814, w1813) -> (w1812:cluster{"X":dbl, "Y":dbl}[])
            }
          }
          n666 = call "IMAQ Point Distances"("Points"=w1790, "error in (no error)"=w1791) -> ("Distances"=w1781:sgl[], "error out"=w1786:errorcluster)  [unwired: 3 in]
          n667 = case shown="True" w1784 {
            tunnel: w1775 -> [_ w1823]
            tunnel: w1786 -> [w1819 w1824]
            tunnel: [w1819 w1825] -> w1785
            tunnel: w1761 -> [_ w1821]
            tunnel: w1762 -> [_ w1822]
            tunnel: w1767 -> [_ w1820]
            frame False {
              # "Measurement overlay disabled"
            }
            frame True {
              # "Measurement overlay enabled"
              n668 = call "IMAQ Overlay Line"("Group"=w1820, "error in (no error)"=w1824, "End Point"=w1821, "Start Point"=w1822, "Image"=w1823) -> ("error out"=w1825:errorcluster)  [unwired: 5 in, 1 out]
            }
          }
          n669 = Bundle By Name(cluster=w1793, "VariableName"=w1767, "VariableType"="Value", "Value"=w1781) -> (w1782:T14)
          n670 = Bundle By Name(cluster=w1778, "PointForOverlays.Points.Points"=w1758, "Measurment Type"="lineSeg", "Measurment Name"=w1767) -> (w1777:T12)
        }
        frame "lineToLine" {
          w1858 = T14 {"VariableName"="", "VariableType"="", "Co-sys Reference"={"Base Co-sys Reference"={"Origin"={"X"=0.0, "Y"=0.0}, "Angle (deg)"=0.0, "Axis Reference"=0, "Scale"=0.0}, "New Co-sys Reference"={"Origin"={"X"=0.0, "Y"=0.0}, "Angle (deg)"=0.0, "Axis Reference"=0, "Scale"=0.0}}, "PointArray"=[], "Line Array"=[], "CircleArrayOUT"=[], "TPDetails"={"DistanceInfo"={"X"=0.0, "Y"=0.0, "X'"=0.0, "Y'"=0.0, "DX"=0.0, "DY"=0.0, "Distance Type"=""}, "Feature and Datum details"=[]}, "Value"=[], "Display Name"=0.0, "ROIArray"=[], "Update ROI "=FALSE}  # AlgoOut
          # "finds the distance between the two lines. it is actually the point to line distance from center point of line 1 to line 2"
          n671 = Index Array(array=w1841) -> (element #1=w1842:T23, element #2=w1843:T23)  [unwired: 2 in]
          n672 = Array Size(array=w1841) -> (size(s)=w1840:i32)
          n673 = Unbundle By Name(w1842) -> ("Line"=w1837:T24)
          n674 = Unbundle By Name(w1843) -> ("Line"=w1836:T24)
          n675 = Equal?(x=w1840, y=2) -> (x = y?=w1829:bool)
          n676 = Index Array(array=w1852) -> (element=w1853:T42)  [unwired: 1 in]
          n677 = Not Equal?(x=w1837, y=w1836) -> (x != y?=w1835:T49)
          n678 = Unbundle By Name(w1853) -> ("Captured Image"=w1838:T3)
          n679 = Unbundle By Name(w1835) -> ("Point 1.X"=w1834:bool, "Point 1.Y"=w1833:bool, "Point 2.X"=w1832:bool, "Point 2.Y"=w1831:bool)
          n680 = Compound Arithmetic op=OR(w1834, w1833, w1832, w1831) -> (w1830:bool)
          n681 = And(x=w1830, y=w1829) -> (x .and. y?=w1828:bool)
          n682 = case shown="True" w1828 {
            tunnel: w1859 -> [w1863 w1886]
            tunnel: w1855 -> [_ w1882]
            tunnel: w1854 -> [_ w1881]
            tunnel: [w1863 w1879] -> w1851
            tunnel: w1838 -> [_ w1878]
            tunnel: [w1861 w1875] -> w1849
            tunnel: w1848 -> [_ w1874]
            tunnel: w1847 -> [_ w1873]
            tunnel: w1844 -> [_ w1872]
            tunnel: w1837 -> [_ w1870]
            tunnel: w1836 -> [_ w1871]
            tunnel: [cluster{"X":sgl, "Y":sgl}[] [{"X"=nan, "Y"=nan}] w1865] -> w1827
            frame False {
              n683 = Build Array(nan) -> (w1861:dbl[])
            }
            frame True {
              n684 = call "lineToline.vi"("error in (no error)"=w1886, "Line2"=w1871, "Line1"=w1870) -> ("error out"=w1883:errorcluster, "lineOUT"=w1864:T32)  [unwired: 6 in, 1 out]
              n685 = Unbundle By Name(w1864) -> ("Point1 (Pixels)"=w1877:cluster{"X":sgl, "Y":sgl}, "Point2 (Pixels)"=w1876:cluster{"X":sgl, "Y":sgl})
              n686 = case shown="True" w1874 {
                tunnel: [w1893 w1897] -> w1885
                tunnel: [w1892 w1894] -> w1884
                tunnel: w1883 -> [w1891 w1897]
                tunnel: w1882 -> [w1889 _]
                tunnel: w1877 -> [w1888 w1900]
                tunnel: w1876 -> [w1887 w1899]
                tunnel: w1873 -> [_ w1898]
                frame False {
                  n687 = Build Array(w1888, w1887) -> (w1890:cluster{"X":sgl, "Y":sgl}[])
                  n688 = call "IMAQ Convert Pixel to Real World"("error in (no error)"=w1891, "Array of Pixel Coordinates"=w1890, "Calibrated Image"=w1889) -> ("error out"=w1893:errorcluster, "Array of Real World Coordinates"=w1892:cluster{"X":sgl, "Y":sgl}[])  [unwired: 3 in, 4 out]
                }
                frame True {
                  n689 = Divide(x=w1900, y=w1898) -> (x/y=w1896:cluster{"X":dbl, "Y":dbl})
                  n690 = Divide(x=w1899, y=w1898) -> (x/y=w1895:cluster{"X":dbl, "Y":dbl})
                  n691 = Build Array(w1896, w1895) -> (w1894:cluster{"X":dbl, "Y":dbl}[])
                }
              }
              n692 = call "IMAQ Point Distances"("Points"=w1884, "error in (no error)"=w1885) -> ("Distances"=w1875:sgl[], "error out"=w1880:errorcluster)  [unwired: 3 in]
              n693 = Unbundle By Name(w1870) -> ("Point 1"=w1869:cluster{"X":sgl, "Y":sgl}, "Point 2"=w1868:cluster{"X":sgl, "Y":sgl})
              n694 = Unbundle By Name(w1871) -> ("Point 1"=w1867:cluster{"X":sgl, "Y":sgl}, "Point 2"=w1866:cluster{"X":sgl, "Y":sgl})
              n695 = case shown="True" w1881 {
                tunnel: w1878 -> [_ w1905]
                tunnel: w1880 -> [w1901 w1906]
                tunnel: [w1901 w1907] -> w1879
                tunnel: w1877 -> [_ w1904]
                tunnel: w1876 -> [_ w1903]
                tunnel: w1872 -> [_ w1902]
                frame False {
                  # "Measurement overlay disabled"
                }
                frame True {
                  # "Measurement overlay enabled"
                  n696 = call "IMAQ Overlay Line"("Group"=w1902, "error in (no error)"=w1906, "End Point"=w1903, "Start Point"=w1904, "Image"=w1905) -> ("error out"=w1907:errorcluster)  [unwired: 5 in, 1 out]
                }
              }
              n697 = Build Array(w1869, w1868, w1867, w1866) -> (w1865:cluster{"X":sgl, "Y":sgl}[])
            }
          }
          n698 = Bundle By Name(cluster=w1845, "Measurment Type"="lineSeg", "Measurment Subtype"="LinetoLine", "Measurment Name"=w1844, "PointForOverlays.Points.Points"=w1827) -> (w1846:T12)
          n699 = Bundle By Name(cluster=w1858, "VariableName"=w1844, "VariableType"="Value", "Value"=w1849) -> (w1856:T14)
        }
        frame "lineToCircle" {
          w1920 = "PointToVirtualLine"  # Measurment Name
          w1919 = "PointToLine"  # Measurment Name
          w1944 = T23 {"Line"={"Point 1"={"X"=0.0, "Y"=0.0}, "Point 2"={"X"=0.0, "Y"=0.0}}, "Straight Edges"=[], "Used Edges"=[]}  # Line
          w1962 = T14 {"VariableName"="", "VariableType"="", "Co-sys Reference"={"Base Co-sys Reference"={"Origin"={"X"=0.0, "Y"=0.0}, "Angle (deg)"=0.0, "Axis Reference"=0, "Scale"=0.0}, "New Co-sys Reference"={"Origin"={"X"=0.0, "Y"=0.0}, "Angle (deg)"=0.0, "Axis Reference"=0, "Scale"=0.0}}, "PointArray"=[], "Line Array"=[], "CircleArrayOUT"=[], "TPDetails"={"DistanceInfo"={"X"=0.0, "Y"=0.0, "X'"=0.0, "Y'"=0.0, "DX"=0.0, "DY"=0.0, "Distance Type"=""}, "Feature and Datum details"=[]}, "Value"=[], "Display Name"=0.0, "ROIArray"=[], "Update ROI "=FALSE}  # AlgoOut
          # "finds the perpendicular distance from the circle's center point to the line"
          n700 = Index Array(array=w1935) -> (element=w1939:T26)  [unwired: 1 in]
          n701 = Index Array(array=w1936) -> (element=w1941:T23)  [unwired: 1 in]
          n702 = Array Size(array=w1936) -> (size(s)=w1934:i32)
          n703 = Array Size(array=w1935) -> (size(s)=w1931:i32)
          n704 = Index Array(array=w1925) -> (element=w1924:sgl)  [unwired: 1 in]
          n705 = Index Array(array=w1955) -> (element=w1956:T42)  [unwired: 1 in]
          n706 = Unbundle By Name(w1939) -> ("CircleDetected"=w1938:T48, "CircleDetected.Center (Pixels)"=w1910:cluster{"X":sgl, "Y":sgl})
          n707 = Greater Or Equal?(x=w1934, y=1) -> (x >= y?=w1929:bool)
          n708 = Greater Or Equal?(x=w1931, y=1) -> (x >= y?=w1930:bool)
          n709 = Unbundle By Name(w1941) -> ("Straight Edges"=w1918:T52, "Line.Point 1"=w1921:cluster{"X":sgl, "Y":sgl}, "Line.Point 2"=w1922:cluster{"X":sgl, "Y":sgl}, "Line"=w1940:T24)
          n710 = Unbundle By Name(w1956) -> ("Captured Image"=w1937:T3)
          n711 = And(x=w1930, y=w1929) -> (x .and. y?=w1928:bool)
          n712 = case shown="True" w1928 {
            tunnel: w1963 -> [w1977 w1982]
            tunnel: [w1977 w1981] -> w1927
            tunnel: w1940 -> [_ w1980]
            tunnel: w1938 -> [_ w1979]
            tunnel: [T32 {"Point1 (Pixels)"={"X"=nan, "Y"=nan}, "Point2 (Pixels)"={"X"=nan, "Y"=nan}} ("lineOut") w1978] -> w1909
            frame False {
            }
            frame True {
              n713 = call "lineToCircle.vi"("error in (no error)"=w1982, "Circle"=w1979, "Line"=w1980) -> ("error out"=w1981:errorcluster, "lineOut"=w1978:T32)  [unwired: 6 in, 1 out]
            }
          }
          n714 = Empty Array?(array=w1918) -> (empty?=w1916:bool)
          n715 = Unbundle By Name(w1909) -> ("Point2 (Pixels)"=w1908:cluster{"X":sgl, "Y":sgl})
          n716 = case shown="True" w1928 {
            tunnel: w1908 -> [_ w1974]
            tunnel: w1910 -> [_ w1973]
            tunnel: [cluster{"X":sgl, "Y":sgl}[] [{"X"=nan, "Y"=nan}] w1975] -> w1915
            tunnel: w1924 -> [_ w1972]
            tunnel: [w1965 w1971] -> w1914
            tunnel: [w1965 w1970] -> w1923
            tunnel: [w1964 w1969] -> w1926
            tunnel: w1927 -> [w1964 w1969]
            tunnel: w1922 -> [_ w1968]
            tunnel: w1921 -> [_ w1967]
            frame False {
              w1965 = cluster{"X":sgl, "Y":sgl} {"X"=nan, "Y"=nan} ("Extended Point 2")
            }
            frame True {
              n717 = call "CircleExtendedDistanceFinding.vi"("Value 2"=w1972, "Point 2"=w1973, "Point 1"=w1974) -> ("Extended Point 2"=w1970:cluster{"X":sgl, "Y":sgl}, "Extended Point 1"=w1971:cluster{"X":sgl, "Y":sgl})  [unwired: 6 in, 1 out]
              n718 = Build Array(w1967, w1968, w1970) -> (w1975:cluster{"X":sgl, "Y":sgl}[])
            }
          }
          n719 = Replace Array Subset(array=w1915, new element=w1914, index=1) -> (w1912:cluster{"X":sgl, "Y":sgl}[])
          n720 = Select(t=w1912, s=w1916, f=w1915) -> (s? t:f=w1911:cluster{"X":sgl, "Y":sgl}[])
          n721 = case shown="True" w1948 {
            tunnel: [w1989 w1990] -> w1959
            tunnel: [w1988 w1991] -> w1958
            tunnel: w1926 -> [w1987 w1990]
            tunnel: w1957 -> [w1985 _]
            tunnel: w1923 -> [w1984 w1995]
            tunnel: w1914 -> [w1983 w1996]
            tunnel: w1949 -> [_ w1994]
            frame False {
              n722 = Build Array(w1983, w1984) -> (w1986:cluster{"X":sgl, "Y":sgl}[])
              n723 = call "IMAQ Convert Pixel to Real World"("error in (no error)"=w1987, "Array of Pixel Coordinates"=w1986, "Calibrated Image"=w1985) -> ("error out"=w1989:errorcluster, "Array of Real World Coordinates"=w1988:cluster{"X":sgl, "Y":sgl}[])  [unwired: 3 in, 4 out]
            }
            frame True {
              n724 = Divide(x=w1996, y=w1994) -> (x/y=w1993:cluster{"X":dbl, "Y":dbl})
              n725 = Divide(x=w1995, y=w1994) -> (x/y=w1992:cluster{"X":dbl, "Y":dbl})
              n726 = Build Array(w1993, w1992) -> (w1991:cluster{"X":dbl, "Y":dbl}[])
            }
          }
          n727 = Bundle By Name(cluster=w1944, "Line"=w1909) -> (w1943:T23)
          n728 = Build Array(w1943) -> (w1942:T18)
          n729 = call "IMAQ Point Distances"("Points"=w1958, "error in (no error)"=w1959) -> ("Distances"=w1950:sgl[], "error out"=w1954:errorcluster)  [unwired: 3 in]
          n730 = Select(t=w1920, s=w1916, f=w1919) -> (s? t:f=w1917:string)
          n731 = Bundle By Name(cluster=w1962, "VariableName"=w1945, "VariableType"="Value", "Line Array"=w1942, "Value"=w1950) -> (w1960:T14)
          n732 = case shown="True" w1951 {
            tunnel: w1937 -> [_ w2001]
            tunnel: w1954 -> [w1997 w2002]
            tunnel: [w1997 w2003] -> w1953
            tunnel: w1923 -> [_ w2000]
            tunnel: w1914 -> [_ w1999]
            tunnel: w1945 -> [_ w1998]
            frame False {
              # "Measurement overlay disabled"
            }
            frame True {
              # "Measurement overlay enabled"
              n733 = call "IMAQ Overlay Line"("Group"=w1998, "error in (no error)"=w2002, "End Point"=w2000, "Start Point"=w1999, "Image"=w2001) -> ("error out"=w2003:errorcluster)  [unwired: 5 in, 1 out]
            }
          }
          n734 = Bundle By Name(cluster=w1946, "PointForOverlays.Points.Points"=w1911, "Measurment Type"="lineSeg", "Measurment Subtype"=w1917, "Measurment Name"=w1945) -> (w1947:T12)
        }
        frame "pointToLine" {
          w2012 = "PointToVirtualLine"  # Measurment Name
          w2011 = "PointToLine"  # Measurment Name
          w2049 = T14 {"VariableName"="", "VariableType"="", "Co-sys Reference"={"Base Co-sys Reference"={"Origin"={"X"=0.0, "Y"=0.0}, "Angle (deg)"=0.0, "Axis Reference"=0, "Scale"=0.0}, "New Co-sys Reference"={"Origin"={"X"=0.0, "Y"=0.0}, "Angle (deg)"=0.0, "Axis Reference"=0, "Scale"=0.0}}, "PointArray"=[], "Line Array"=[], "CircleArrayOUT"=[], "TPDetails"={"DistanceInfo"={"X"=0.0, "Y"=0.0, "X'"=0.0, "Y'"=0.0, "DX"=0.0, "DY"=0.0, "Distance Type"=""}, "Feature and Datum details"=[]}, "Value"=[], "Display Name"=0.0, "ROIArray"=[], "Update ROI "=FALSE}  # AlgoOut
          n735 = Index Array(array=w2040) -> (element=w2041:T42)  [unwired: 1 in]
          n736 = Index Array(array=w2025) -> (element=w2026:cluster{"X":sgl, "Y":sgl})  [unwired: 1 in]
          n737 = Index Array(array=w2020) -> (element=w2029:T23)  [unwired: 1 in]
          n738 = Unbundle By Name(w2041) -> ("Captured Image"=w2028:T3)
          n739 = Unbundle By Name(w2029) -> ("Straight Edges"=w2013:T52, "Line.Point 1"=w2015:cluster{"X":sgl, "Y":sgl}, "Line.Point 2"=w2016:cluster{"X":sgl, "Y":sgl}, "Line"=w2027:T24)
          n740 = Array Size(array=w2020) -> (size(s)=w2021:i32)
          n741 = Array Size(array=w2025) -> (size(s)=w2024:i32)
          n742 = Equal?(x=w2021, y=1) -> (x = y?=w2019:bool)
          n743 = Equal?(x=w2024, y=1) -> (x = y?=w2018:bool)
          n744 = And(x=w2019, y=w2018) -> (x .and. y?=w2017:bool)
          n745 = Empty Array?(array=w2013) -> (empty?=w2009:bool)
          n746 = case shown="True" w2017 {
            tunnel: w2050 -> [w2053 w2061]
            tunnel: [w2053 w2060] -> w2045
            tunnel: [T24 {"Point 1"={"X"=nan, "Y"=nan}, "Point 2"={"X"=nan, "Y"=nan}} ("Line") w2059] -> w2044
            tunnel: w2027 -> [_ w2058]
            tunnel: w2026 -> [_ w2057]
            tunnel: w2016 -> [_ w2056]
            tunnel: w2015 -> [_ w2055]
            tunnel: [cluster{"X":sgl, "Y":sgl}[] [{"X"=nan, "Y"=nan}] w2054] -> w2008
            frame False {
            }
            frame True {
              n747 = call "pointToLine.vi"("error in (no error)"=w2061, "Line"=w2058, "Point"=w2057) -> ("error out"=w2060:errorcluster, "Line"=w2059:T24)  [unwired: 6 in, 1 out]
              n748 = Build Array(w2055, w2056, w2057) -> (w2054:cluster{"X":sgl, "Y":sgl}[])
            }
          }
          n749 = Unbundle By Name(w2044) -> ("Point 1"=w2036:cluster{"X":sgl, "Y":sgl}, "Point 2"=w2007:cluster{"X":sgl, "Y":sgl})
          n750 = case shown="False" w2034 {
            tunnel: [w2068 w2075] -> w2046
            tunnel: w2045 -> [w2067 w2075]
            tunnel: [w2065 w2069] -> w2043
            tunnel: w2042 -> [w2064 _]
            tunnel: w2036 -> [w2063 w2074]
            tunnel: w2007 -> [w2062 w2073]
            tunnel: w2033 -> [_ w2072]
            frame False {
              n751 = Build Array(w2063, w2062) -> (w2066:cluster{"X":sgl, "Y":sgl}[])
              n752 = call "IMAQ Convert Pixel to Real World"("error in (no error)"=w2067, "Array of Pixel Coordinates"=w2066, "Calibrated Image"=w2064) -> ("error out"=w2068:errorcluster, "Array of Real World Coordinates"=w2065:cluster{"X":sgl, "Y":sgl}[])  [unwired: 3 in, 4 out]
            }
            frame True {
              n753 = Divide(x=w2074, y=w2072) -> (x/y=w2071:cluster{"X":dbl, "Y":dbl})
              n754 = Divide(x=w2073, y=w2072) -> (x/y=w2070:cluster{"X":dbl, "Y":dbl})
              n755 = Build Array(w2071, w2070) -> (w2069:cluster{"X":dbl, "Y":dbl}[])
            }
          }
          n756 = Replace Array Subset(array=w2008, new element=w2007, index=1) -> (w2006:cluster{"X":sgl, "Y":sgl}[])
          n757 = call "IMAQ Point Distances"("Points"=w2043, "error in (no error)"=w2046) -> ("Distances"=w2035:sgl[], "error out"=w2039:errorcluster)  [unwired: 3 in]
          n758 = Select(t=w2006, s=w2009, f=w2008) -> (s? t:f=w2005:cluster{"X":sgl, "Y":sgl}[])
          n759 = case shown="True" w2014 {
            tunnel: w2028 -> [_ w2080]
            tunnel: w2039 -> [w2076 w2081]
            tunnel: [w2076 w2082] -> w2038
            tunnel: w2036 -> [_ w2078]
            tunnel: w2007 -> [_ w2079]
            tunnel: w2030 -> [_ w2077]
            frame False {
              # "Measurement overlay disabled"
            }
            frame True {
              # "Measurement overlay enabled"
              n760 = call "IMAQ Overlay Line"("Group"=w2077, "error in (no error)"=w2081, "End Point"=w2079, "Start Point"=w2078, "Image"=w2080) -> ("error out"=w2082:errorcluster)  [unwired: 5 in, 1 out]
            }
          }
          n761 = Select(t=w2012, s=w2009, f=w2011) -> (s? t:f=w2010:string)
          n762 = Bundle By Name(cluster=w2031, "Measurment Subtype"=w2010, "Measurment Type"="lineSeg", "Measurment Name"=w2030, "PointForOverlays.Points.Points"=w2005) -> (w2032:T12)
          n763 = Bundle By Name(cluster=w2049, "VariableName"=w2030, "VariableType"="Value", "Value"=w2035) -> (w2047:T14)
        }
        frame "circleToCircle" {
          w2123 = T14 {"VariableName"="", "VariableType"="", "Co-sys Reference"={"Base Co-sys Reference"={"Origin"={"X"=0.0, "Y"=0.0}, "Angle (deg)"=0.0, "Axis Reference"=0, "Scale"=0.0}, "New Co-sys Reference"={"Origin"={"X"=0.0, "Y"=0.0}, "Angle (deg)"=0.0, "Axis Reference"=0, "Scale"=0.0}}, "PointArray"=[], "Line Array"=[], "CircleArrayOUT"=[], "TPDetails"={"DistanceInfo"={"X"=0.0, "Y"=0.0, "X'"=0.0, "Y'"=0.0, "DX"=0.0, "DY"=0.0, "Distance Type"=""}, "Feature and Datum details"=[]}, "Value"=[], "Display Name"=0.0, "ROIArray"=[], "Update ROI "=FALSE}  # AlgoOut
          # "finds the distance between the two circles, it is actually the point to point distance from center of circle 1 to  center of circle 2"
          n764 = Index Array(array=w2106) -> (element #1=w2108:T26, element #2=w2107:T26)  [unwired: 2 in]
          n765 = Index Array(array=w2091) -> (element #1=w2088:sgl, element #2=w2087:sgl)  [unwired: 2 in]
          n766 = Index Array(array=w2118) -> (element=w2119:T42)  [unwired: 1 in]
          n767 = Unbundle By Name(w2108) -> ("CircleDetected.Center (Pixels)"=w2097:cluster{"X":sgl, "Y":sgl}, "CircleDetected.Radius (Pixels)"=w2084:dbl)
          n768 = Unbundle By Name(w2107) -> ("CircleDetected.Center (Pixels)"=w2093:cluster{"X":sgl, "Y":sgl})
          n769 = Array Size(array=w2091) -> (size(s)=w2092:i32)
          n770 = Unbundle By Name(w2119) -> ("Captured Image"=w2103:T3)
          n771 = Equal?(x=w2092, y=2) -> (x = y?=w2089:bool)
          n772 = case shown="False" w2089 {
            tunnel: w2087 -> [_ w2139]
            tunnel: w2088 -> [w2130 w2140]
            tunnel: [w2136 w2140] -> w2086
            tunnel: [w2133 w2139] -> w2085
            tunnel: w2084 -> [w2125 _]
            frame False {
              w2134 = sgl 0.0 ("f")
              n773 = Negate(x=w2125) -> (-x=w2127:dbl)
              n774 = Number To Fractional String(number=w2125, precision (6)=i16 3) -> (F-format string=w2124:string)  [unwired: 2 in]
              n775 = Number To Fractional String(number=w2127, precision (6)=i16 3) -> (F-format string=w2128:string)  [unwired: 2 in]
              n776 = Number To Fractional String(number=w2130, precision (6)=i16 3) -> (F-format string=w2131:string)  [unwired: 2 in]
              n777 = Equal?(x=w2124, y=w2131) -> (x = y?=w2137:bool)
              n778 = Equal?(x=w2128, y=w2131) -> (x = y?=w2138:bool)
              n779 = Or(x=w2137, y=w2138) -> (x .or. y?=w2135:bool)
              n780 = Select(t=w2130, s=w2135, f=w2134) -> (s? t:f=w2136:sgl)
              n781 = Select(t=w2134, s=w2135, f=w2130) -> (s? t:f=w2133:sgl)
            }
            frame True {
            }
          }
          n782 = Array Size(array=w2106) -> (size(s)=w2105:i32)
          n783 = Equal?(x=w2105, y=2) -> (x = y?=w2098:bool)
          n784 = case shown="True" w2098 {
            tunnel: w2083 -> [w2143 w2146]
            tunnel: [w2143 w2146] -> w2100
            tunnel: w2097 -> [_ w2150]
            tunnel: w2093 -> [_ w2149]
            tunnel: [cluster{"X":sgl, "Y":sgl}[] [{"X"=nan, "Y"=nan}] w2151] -> w2096
            tunnel: w2086 -> [_ w2148]
            tunnel: w2085 -> [_ w2147]
            tunnel: [w2141 w2145] -> w2095
            tunnel: [w2141 w2144] -> w2094
            frame False {
              w2141 = cluster{"X":sgl, "Y":sgl} {"X"=nan, "Y"=nan} ("Extended Point 2")
            }
            frame True {
              n785 = call "CircleExtendedDistanceFinding.vi"("Value 2"=w2147, "Value 1"=w2148, "Point 2"=w2149, "Point 1"=w2150) -> ("Extended Point 2"=w2144:cluster{"X":sgl, "Y":sgl}, "Extended Point 1"=w2145:cluster{"X":sgl, "Y":sgl})  [unwired: 5 in, 1 out]
              n786 = Build Array(w2145, w2144) -> (w2151:cluster{"X":sgl, "Y":sgl}[])
            }
          }
          n787 = case shown="False" w2113 {
            tunnel: [w2158 w2165] -> w2102
            tunnel: [w2157 w2159] -> w2101
            tunnel: w2100 -> [w2156 w2165]
            tunnel: w2120 -> [w2154 _]
            tunnel: w2094 -> [w2153 w2163]
            tunnel: w2095 -> [w2152 w2164]
            tunnel: w2112 -> [_ w2162]
            frame False {
              n788 = Build Array(w2152, w2153) -> (w2155:cluster{"X":sgl, "Y":sgl}[])
              n789 = call "IMAQ Convert Pixel to Real World"("error in (no error)"=w2156, "Array of Pixel Coordinates"=w2155, "Calibrated Image"=w2154) -> ("error out"=w2158:errorcluster, "Array of Real World Coordinates"=w2157:cluster{"X":sgl, "Y":sgl}[])  [unwired: 3 in, 4 out]
            }
            frame True {
              n790 = Divide(x=w2164, y=w2162) -> (x/y=w2161:cluster{"X":dbl, "Y":dbl})
              n791 = Divide(x=w2163, y=w2162) -> (x/y=w2160:cluster{"X":dbl, "Y":dbl})
              n792 = Build Array(w2161, w2160) -> (w2159:cluster{"X":dbl, "Y":dbl}[])
            }
          }
          n793 = call "IMAQ Point Distances"("Points"=w2101, "error in (no error)"=w2102) -> ("Distances"=w2114:sgl[], "error out"=w2099:errorcluster)  [unwired: 3 in]
          n794 = case shown="True" w2116 {
            tunnel: w2103 -> [_ w2170]
            tunnel: w2099 -> [w2166 w2171]
            tunnel: [w2166 w2172] -> w2117
            tunnel: w2094 -> [_ w2169]
            tunnel: w2095 -> [_ w2168]
            tunnel: w2109 -> [_ w2167]
            frame False {
              # "Measurement overlay disabled"
            }
            frame True {
              # "Measurement overlay enabled"
              n795 = call "IMAQ Overlay Line"("Group"=w2167, "error in (no error)"=w2171, "End Point"=w2169, "Start Point"=w2168, "Image"=w2170) -> ("error out"=w2172:errorcluster)  [unwired: 5 in, 1 out]
            }
          }
          n796 = Bundle By Name(cluster=w2111, "Measurment Type"="lineSeg", "Measurment Name"=w2109, "PointForOverlays.Points.Points"=w2096) -> (w2110:T12)
          n797 = Bundle By Name(cluster=w2123, "VariableName"=w2109, "VariableType"="Value", "Value"=w2114) -> (w2121:T14)
        }
        frame "PointtoPointParallel" {
          w2220 = T14 {"VariableName"="", "VariableType"="", "Co-sys Reference"={"Base Co-sys Reference"={"Origin"={"X"=0.0, "Y"=0.0}, "Angle (deg)"=0.0, "Axis Reference"=0, "Scale"=0.0}, "New Co-sys Reference"={"Origin"={"X"=0.0, "Y"=0.0}, "Angle (deg)"=0.0, "Axis Reference"=0, "Scale"=0.0}}, "PointArray"=[], "Line Array"=[], "CircleArrayOUT"=[], "TPDetails"={"DistanceInfo"={"X"=0.0, "Y"=0.0, "X'"=0.0, "Y'"=0.0, "DX"=0.0, "DY"=0.0, "Distance Type"=""}, "Feature and Datum details"=[]}, "Value"=[], "Display Name"=0.0, "ROIArray"=[], "Update ROI "=FALSE}  # AlgoOut
          # "Overlay Points order\nPara = Pi,P2,P1\nPer = Pi, P1,P2"
          # "Distance Between any two points in parallel with the reference Line"
          n798 = Array Size(array=w2206) -> (size(s)=w2209:i32)
          n799 = Array Size(array=w2205) -> (size(s)=w2212:i32)
          n800 = Index Array(array=w2206) -> (element=w2224:T23)  [unwired: 1 in]
          n801 = Index Array(array=w2205) -> (element #1=w2184:cluster{"X":sgl, "Y":sgl}, element #2=w2182:cluster{"X":sgl, "Y":sgl})  [unwired: 2 in]
          n802 = Unbundle By Name(w2224) -> ("Line"=w2194:T24, "Line.Point 1"=w2185:cluster{"X":sgl, "Y":sgl}, "Line.Point 2"=w2183:cluster{"X":sgl, "Y":sgl})
          n803 = Greater Or Equal?(x=w2209, y=1) -> (x >= y?=w2208:bool)
          n804 = Greater Or Equal?(x=w2212, y=2) -> (x >= y?=w2207:bool)
          n805 = And(x=w2208, y=w2207) -> (x .and. y?=w2200:bool)
          n806 = Not Equal?(x=w2184, y=w2182) -> (x != y?=w2204:cluster{"X":bool, "Y":bool})
          n807 = Equal?(x=w2183, y=w2184) -> (x = y?=w2190:cluster{"X":bool, "Y":bool})
          n808 = Unbundle By Name(w2204) -> ("X"=w2203:bool, "Y"=w2202:bool)
          n809 = Cluster To Array(cluster=w2190) -> (array=w2191:bool[])
          n810 = Equal?(x=w2185, y=w2184) -> (x = y?=w2186:cluster{"X":bool, "Y":bool})
          n811 = Equal?(x=w2183, y=w2182) -> (x = y?=w2179:cluster{"X":bool, "Y":bool})
          n812 = And Array Elements(Boolean array=w2191) -> (logical AND=w2189:bool)
          n813 = Cluster To Array(cluster=w2186) -> (array=w2187:bool[])
          n814 = Cluster To Array(cluster=w2179) -> (array=w2178:bool[])
          n815 = Or(x=w2203, y=w2202) -> (x .or. y?=w2201:bool)
          n816 = And Array Elements(Boolean array=w2187) -> (logical AND=w2181:bool)
          n817 = And Array Elements(Boolean array=w2178) -> (logical AND=w2180:bool)
          n818 = And(x=w2201, y=w2200) -> (x .and. y?=w2174:bool)
          n819 = And(x=w2181, y=w2180) -> (x .and. y?=w2177:bool)
          n820 = Equal?(x=w2185, y=w2182) -> (x = y?=w2193:cluster{"X":bool, "Y":bool})
          n821 = Cluster To Array(cluster=w2193) -> (array=w2192:bool[])
          n822 = And Array Elements(Boolean array=w2192) -> (logical AND=w2188:bool)
          n823 = And(x=w2188, y=w2189) -> (x .and. y?=w2176:bool)
          n824 = Not Or(1:w2176, 2:w2177) -> (0:w2175:bool)
          n825 = And(x=w2175, y=w2174) -> (x .and. y?=w2173:bool)
          n826 = case shown="True" w2173 {
            tunnel: w2225 -> [w2228 w2249]
            tunnel: w2194 -> [_ w2248]
            tunnel: w2184 -> [_ w2238]
            tunnel: w2182 -> [_ w2231]
            tunnel: w2223 -> [_ w2243]
            tunnel: w2222 -> [_ w2242]
            tunnel: w2221 -> [_ w2241]
            tunnel: [sgl[] [nan] ("X") w2240] -> w2214
            tunnel: [w2228 w2239] -> w2199
            tunnel: [cluster{"X":sgl, "Y":sgl}[] [{"X"=nan, "Y"=nan}] ("Point 1") w2237] -> w2198
            tunnel: w2197 -> [_ w2234]
            tunnel: w2196 -> [_ w2230]
            frame False {
            }
            frame True {
              n827 = call "Point2Point Parallel  Perpendicular.vi"("error in (no error)"=w2249, "Point 2"=w2231, "Point 1"=w2238, "Reference Line"=w2248) -> ("error out"=w2244:errorcluster, "Parallel Line"=w2245:cluster{"X":sgl, "Y":sgl}[])  [unwired: 4 in, 2 out]
              n828 = Index Array(array=w2245) -> (element #1=w2236:cluster{"X":sgl, "Y":sgl}, element #2=w2235:cluster{"X":sgl, "Y":sgl})  [unwired: 2 in]
              n829 = call "Check for Circle.vi"("Point"=w2236, "Point 3"=w2231, "Point 2"=w2235, "CircleArrayOUT"=w2234, "Values Array"=w2230) -> ("point 3"=w2229:cluster{"X":sgl, "Y":sgl}, "Extended Point 1"=w2233:cluster{"X":sgl, "Y":sgl}, "Extended Point 2"=w2232:cluster{"X":sgl, "Y":sgl})  [unwired: 8 in]
              n830 = Build Array(w2229, w2233, w2232) -> (w2237:cluster{"X":sgl, "Y":sgl}[])
              n831 = case shown="False" w2243 {
                tunnel: [w2256 w2263] -> w2247
                tunnel: [w2255 w2257] -> w2246
                tunnel: w2244 -> [w2254 w2263]
                tunnel: w2241 -> [w2252 _]
                tunnel: w2232 -> [w2251 w2261]
                tunnel: w2233 -> [w2250 w2262]
                tunnel: w2242 -> [_ w2260]
                frame False {
                  n832 = Build Array(w2250, w2251) -> (w2253:cluster{"X":sgl, "Y":sgl}[])
                  n833 = call "IMAQ Convert Pixel to Real World"("error in (no error)"=w2254, "Array of Pixel Coordinates"=w2253, "Calibrated Image"=w2252) -> ("error out"=w2256:errorcluster, "Array of Real World Coordinates"=w2255:cluster{"X":sgl, "Y":sgl}[])  [unwired: 3 in, 4 out]
                }
                frame True {
                  n834 = Divide(x=w2262, y=w2260) -> (x/y=w2259:cluster{"X":dbl, "Y":dbl})
                  n835 = Divide(x=w2261, y=w2260) -> (x/y=w2258:cluster{"X":dbl, "Y":dbl})
                  n836 = Build Array(w2259, w2258) -> (w2257:cluster{"X":dbl, "Y":dbl}[])
                }
              }
              n837 = call "IMAQ Point Distances"("Points"=w2246, "error in (no error)"=w2247) -> ("Distances"=w2240:sgl[], "error out"=w2239:errorcluster)  [unwired: 3 in]
            }
          }
          n838 = Bundle By Name(cluster=w2217, "PointForOverlays.Points.Points"=w2198, "Measurment Name"=w2216, "Measurment Type"="LineSeg", "Measurment Subtype"="PointToVirtualLine" ("Measurment Type"), "Result"=w2214) -> (w2213:T12)
          n839 = Bundle By Name(cluster=w2220, "VariableName"=w2216, "VariableType"="Value", "Value"=w2214) -> (w2218:T14)
        }
        frame "PointtoPointPerpendicular" {
          w2311 = T14 {"VariableName"="", "VariableType"="", "Co-sys Reference"={"Base Co-sys Reference"={"Origin"={"X"=0.0, "Y"=0.0}, "Angle (deg)"=0.0, "Axis Reference"=0, "Scale"=0.0}, "New Co-sys Reference"={"Origin"={"X"=0.0, "Y"=0.0}, "Angle (deg)"=0.0, "Axis Reference"=0, "Scale"=0.0}}, "PointArray"=[], "Line Array"=[], "CircleArrayOUT"=[], "TPDetails"={"DistanceInfo"={"X"=0.0, "Y"=0.0, "X'"=0.0, "Y'"=0.0, "DX"=0.0, "DY"=0.0, "Distance Type"=""}, "Feature and Datum details"=[]}, "Value"=[], "Display Name"=0.0, "ROIArray"=[], "Update ROI "=FALSE}  # AlgoOut
          # "Overlay Points order\nPara = Pi,P2,P1\nPer = Pi, P1,P2"
          # "Distance Between any two points in parallel with the reference Line"
          n840 = Array Size(array=w2297) -> (size(s)=w2300:i32)
          n841 = Array Size(array=w2296) -> (size(s)=w2303:i32)
          n842 = Index Array(array=w2297) -> (element=w2315:T23)  [unwired: 1 in]
          n843 = Index Array(array=w2296) -> (element #1=w2271:cluster{"X":sgl, "Y":sgl}, element #2=w2275:cluster{"X":sgl, "Y":sgl})  [unwired: 2 in]
          n844 = Unbundle By Name(w2315) -> ("Line"=w2314:T24, "Line.Point 1"=w2272:cluster{"X":sgl, "Y":sgl}, "Line.Point 2"=w2276:cluster{"X":sgl, "Y":sgl})
          n845 = Greater Or Equal?(x=w2300, y=1) -> (x >= y?=w2299:bool)
          n846 = Greater Or Equal?(x=w2303, y=2) -> (x >= y?=w2298:bool)
          n847 = And(x=w2299, y=w2298) -> (x .and. y?=w2291:bool)
          n848 = Equal?(x=w2276, y=w2271) -> (x = y?=w2282:cluster{"X":bool, "Y":bool})
          n849 = Not Equal?(x=w2271, y=w2275) -> (x != y?=w2295:cluster{"X":bool, "Y":bool})
          n850 = Cluster To Array(cluster=w2282) -> (array=w2281:bool[])
          n851 = And Array Elements(Boolean array=w2281) -> (logical AND=w2279:bool)
          n852 = Equal?(x=w2272, y=w2275) -> (x = y?=w2283:cluster{"X":bool, "Y":bool})
          n853 = Unbundle By Name(w2295) -> ("X"=w2294:bool, "Y"=w2293:bool)
          n854 = Cluster To Array(cluster=w2283) -> (array=w2284:bool[])
          n855 = Equal?(x=w2276, y=w2275) -> (x = y?=w2278:cluster{"X":bool, "Y":bool})
          n856 = And Array Elements(Boolean array=w2284) -> (logical AND=w2280:bool)
          n857 = Cluster To Array(cluster=w2278) -> (array=w2277:bool[])
          n858 = Or(x=w2294, y=w2293) -> (x .or. y?=w2292:bool)
          n859 = And Array Elements(Boolean array=w2277) -> (logical AND=w2269:bool)
          n860 = And(x=w2280, y=w2279) -> (x .and. y?=w2267:bool)
          n861 = And(x=w2292, y=w2291) -> (x .and. y?=w2265:bool)
          n862 = Equal?(x=w2272, y=w2271) -> (x = y?=w2273:cluster{"X":bool, "Y":bool})
          n863 = Cluster To Array(cluster=w2273) -> (array=w2274:bool[])
          n864 = And Array Elements(Boolean array=w2274) -> (logical AND=w2270:bool)
          n865 = And(x=w2270, y=w2269) -> (x .and. y?=w2268:bool)
          n866 = Not Or(1:w2267, 2:w2268) -> (0:w2266:bool)
          n867 = And(x=w2266, y=w2265) -> (x .and. y?=w2264:bool)
          n868 = case shown="True" w2264 {
            tunnel: w2316 -> [w2319 w2340]
            tunnel: w2314 -> [_ w2339]
            tunnel: w2271 -> [_ w2322]
            tunnel: w2275 -> [_ w2324]
            tunnel: w2287 -> [_ w2335]
            tunnel: w2313 -> [_ w2334]
            tunnel: w2312 -> [_ w2333]
            tunnel: [sgl[] [nan] ("X") w2332] -> w2305
            tunnel: [w2319 w2331] -> w2290
            tunnel: [cluster{"X":sgl, "Y":sgl}[] [{"X"=nan, "Y"=nan}] ("Point 1") w2329] -> w2289
            tunnel: w2288 -> [_ w2328]
            tunnel: w2286 -> [_ w2321]
            frame False {
            }
            frame True {
              n869 = call "Point2Point Parallel  Perpendicular.vi"("error in (no error)"=w2340, "Point 2"=w2324, "Point 1"=w2322, "Reference Line"=w2339) -> ("error out"=w2336:errorcluster, "Perpendicular Line"=w2330:cluster{"X":sgl, "Y":sgl}[])  [unwired: 4 in, 2 out]
              n870 = Index Array(array=w2330) -> (element #1=w2327:cluster{"X":sgl, "Y":sgl}, element #2=w2326:cluster{"X":sgl, "Y":sgl})  [unwired: 2 in]
              n871 = call "Check for Circle.vi"("Point"=w2327, "Point 3"=w2322, "Point 2"=w2326, "CircleArrayOUT"=w2328, "Values Array"=w2321) -> ("point 3"=w2320:cluster{"X":sgl, "Y":sgl}, "Extended Point 1"=w2325:cluster{"X":sgl, "Y":sgl}, "Extended Point 2"=w2323:cluster{"X":sgl, "Y":sgl})  [unwired: 8 in]
              n872 = case shown="False" w2335 {
                tunnel: [w2347 w2354] -> w2338
                tunnel: [w2346 w2348] -> w2337
                tunnel: w2336 -> [w2345 w2354]
                tunnel: w2333 -> [w2343 _]
                tunnel: w2323 -> [w2342 w2352]
                tunnel: w2325 -> [w2341 w2353]
                tunnel: w2334 -> [_ w2351]
                frame False {
                  n873 = Build Array(w2341, w2342) -> (w2344:cluster{"X":sgl, "Y":sgl}[])
                  n874 = call "IMAQ Convert Pixel to Real World"("error in (no error)"=w2345, "Array of Pixel Coordinates"=w2344, "Calibrated Image"=w2343) -> ("error out"=w2347:errorcluster, "Array of Real World Coordinates"=w2346:cluster{"X":sgl, "Y":sgl}[])  [unwired: 3 in, 4 out]
                }
                frame True {
                  n875 = Divide(x=w2353, y=w2351) -> (x/y=w2350:cluster{"X":dbl, "Y":dbl})
                  n876 = Divide(x=w2352, y=w2351) -> (x/y=w2349:cluster{"X":dbl, "Y":dbl})
                  n877 = Build Array(w2350, w2349) -> (w2348:cluster{"X":dbl, "Y":dbl}[])
                }
              }
              n878 = Build Array(w2320, w2325, w2323) -> (w2329:cluster{"X":sgl, "Y":sgl}[])
              n879 = call "IMAQ Point Distances"("Points"=w2337, "error in (no error)"=w2338) -> ("Distances"=w2332:sgl[], "error out"=w2331:errorcluster)  [unwired: 3 in]
            }
          }
          n880 = Bundle By Name(cluster=w2308, "PointForOverlays.Points.Points"=w2289, "Measurment Name"=w2307, "Measurment Type"="LineSeg", "Measurment Subtype"="PointToVirtualLine" ("Measurment Type"), "Result"=w2305) -> (w2304:T12)
          n881 = Bundle By Name(cluster=w2311, "VariableName"=w2307, "VariableType"="Value", "Value"=w2305) -> (w2309:T14)
        }
        frame "RadiusDifference" {
          w2374 = T14 {"VariableName"="", "VariableType"="", "Co-sys Reference"={"Base Co-sys Reference"={"Origin"={"X"=0.0, "Y"=0.0}, "Angle (deg)"=0.0, "Axis Reference"=0, "Scale"=0.0}, "New Co-sys Reference"={"Origin"={"X"=0.0, "Y"=0.0}, "Angle (deg)"=0.0, "Axis Reference"=0, "Scale"=0.0}}, "PointArray"=[], "Line Array"=[], "CircleArrayOUT"=[], "TPDetails"={"DistanceInfo"={"X"=0.0, "Y"=0.0, "X'"=0.0, "Y'"=0.0, "DX"=0.0, "DY"=0.0, "Distance Type"=""}, "Feature and Datum details"=[]}, "Value"=[], "Display Name"=0.0, "ROIArray"=[], "Update ROI "=FALSE}  # AlgoOut
          n882 = Index Array "Indexing  Circle Array"(array=w2377) -> (element #1=w2376:T26, element #2=w2375:T26)  [unwired: 2 in]
          n883 = Unbundle By Name(w2376) -> ("CircleDetected.Center (Pixels)"=w2368:cluster{"X":sgl, "Y":sgl}, "CircleDetected.Radius (Pixels)"=w2364:dbl)
          n884 = Unbundle By Name(w2375) -> ("CircleDetected.Center (Pixels)"=w2363:cluster{"X":sgl, "Y":sgl}, "CircleDetected.Radius (Pixels)"=w2367:dbl)
          n885 = call "RadiusDifference.vi"("circle 1"=w2368, "r1"=w2364, "circle 2"=w2363, "r2"=w2367, "conversion\nfactor"=w2361, "error in"=w2378) -> ("Radius\ndifference"=w2362:dbl, "concentricity or not?"=w2358:bool, "error out"=w2366:errorcluster)  [unwired: 11 in]
          n886 = Build Array(w2362) -> (w2370:dbl[])
          n887 = case shown="True" w2358 {
            tunnel: w2368 -> [_ w2389]
            tunnel: w2367 -> [_ w2388]
            tunnel: [w2381 w2387] -> w2357
            tunnel: [w2380 w2386] -> w2356
            tunnel: w2366 -> [w2379 w2385]
            tunnel: [w2379 w2384] -> w2365
            tunnel: w2364 -> [_ w2383]
            tunnel: w2363 -> [_ w2382]
            frame False {
              w2380 = cluster{dbl, "centre y":dbl} {nan, "centre y"=nan}  # EndPoint
              w2381 = cluster{dbl, "centre y":dbl} {nan, "centre y"=nan}  # start point
            }
            frame True {
              n888 = call "overlay computation for radius difference algo.vi"("circle 1"=w2389, "r1"=w2383, "circle 2"=w2382, "r2"=w2388, "error in (no error)"=w2385) -> ("start point"=w2387:cluster{dbl, "centre y":dbl}, "EndPoint"=w2386:cluster{dbl, "centre y":dbl}, "error IO"=w2384:errorcluster)  [unwired: 8 in]
            }
          }
          n889 = Bundle By Name(cluster=w2374, "VariableName"=w2369, "VariableType"="Value", "Value"=w2370) -> (w2359:T14)
          n890 = Build Array(w2357, w2356) -> (w2355:cluster{dbl, "centre y":dbl}[])
          n891 = Bundle By Name(cluster=w2371, "PointForOverlays.Points.Points"=w2355, "Measurment Name"=w2369, "Measurment Type"="LineSeg", "Result"=w2370) -> (w2360:T12)
        }
        frame "AverageClamp" {
          w2413 = T14 {"VariableName"="", "VariableType"="", "Co-sys Reference"={"Base Co-sys Reference"={"Origin"={"X"=0.0, "Y"=0.0}, "Angle (deg)"=0.0, "Axis Reference"=0, "Scale"=0.0}, "New Co-sys Reference"={"Origin"={"X"=0.0, "Y"=0.0}, "Angle (deg)"=0.0, "Axis Reference"=0, "Scale"=0.0}}, "PointArray"=[], "Line Array"=[], "CircleArrayOUT"=[], "TPDetails"={"DistanceInfo"={"X"=0.0, "Y"=0.0, "X'"=0.0, "Y'"=0.0, "DX"=0.0, "DY"=0.0, "Distance Type"=""}, "Feature and Datum details"=[]}, "Value"=[], "Display Name"=0.0, "ROIArray"=[], "Update ROI "=FALSE}  # AlgoOut
          n892 = Index Array(array=w2404) -> (element=w2403:T42)  [unwired: 1 in]
          n893 = Unbundle By Name(w2401) -> ("ROI"=w2400:T47, "Edge Options"=w2399:T5, "Line Options.Step Size"=w2398:u32, "Search Direction"=w2391:u16)
          n894 = Unbundle By Name(w2403) -> ("Captured Image"=w2402:T3)
          n895 = call "Average Clamp.vi"("Refnum in"=w2402, "ROI Descriptor in"=w2400, "Edge Options"=w2399, "Step Size"=w2398, "conversion \nfactor"=w2397, "error in"=w2406, "Scan Direction"=w2391) -> ("distance"=w2396:dbl, "line1"=w2394:cluster{"X":sgl, "Y":sgl}[], "line 2"=w2393:cluster{"X":sgl, "Y":sgl}[], "error out"=w2405:errorcluster)  [unwired: 9 in]
          n896 = Build Array (concatenate)(w2394, w2393) -> (w2392:cluster{"X":sgl, "Y":sgl}[])
          n897 = Build Array(w2396) -> (w2395:dbl[])
          n898 = Bundle By Name(cluster=w2413, "VariableName"=w2409, "VariableType"="Value", "Value"=w2395) -> (w2407:T14)
          n899 = Bundle By Name(cluster=w2410, "PointForOverlays.Points.Points"=w2392, "Measurment Name"=w2409, "Measurment Type"="LineSeg", "Measurment Subtype"="LineToLine", "Result"=w2395) -> (w2408:T12)
        }
        frame "MaxClamp" {
          w2435 = T14 {"VariableName"="", "VariableType"="", "Co-sys Reference"={"Base Co-sys Reference"={"Origin"={"X"=0.0, "Y"=0.0}, "Angle (deg)"=0.0, "Axis Reference"=0, "Scale"=0.0}, "New Co-sys Reference"={"Origin"={"X"=0.0, "Y"=0.0}, "Angle (deg)"=0.0, "Axis Reference"=0, "Scale"=0.0}}, "PointArray"=[], "Line Array"=[], "CircleArrayOUT"=[], "TPDetails"={"DistanceInfo"={"X"=0.0, "Y"=0.0, "X'"=0.0, "Y'"=0.0, "DX"=0.0, "DY"=0.0, "Distance Type"=""}, "Feature and Datum details"=[]}, "Value"=[], "Display Name"=0.0, "ROIArray"=[], "Update ROI "=FALSE}  # AlgoOut
          n900 = Index Array(array=w2426) -> (element=w2425:T42)  [unwired: 1 in]
          n901 = Unbundle By Name(w2423) -> ("ROI"=w2422:T47, "Edge Options"=w2417:T5, "Line Options.Step Size"=w2416:u32, "Search Direction"=w2415:u16)
          n902 = Unbundle By Name(w2425) -> ("Captured Image"=w2424:T3)
          n903 = call "max clamp.vi"("Refnum in"=w2424, "ROI Descriptor out"=w2422, "Edge\nOptions"=w2417, "Step size"=w2416, "Scan Direction"=w2415, "conversion factor"=w2414, "error in (no error)"=w2428) -> ("distance"=w2421:dbl, "Line"=w2419:cluster{"X":sgl, "Y":sgl}[], "error out"=w2427:errorcluster)  [unwired: 18 in]
          n904 = Build Array(w2421) -> (w2420:dbl[])
          n905 = Bundle By Name(cluster=w2435, "VariableName"=w2431, "VariableType"="Value", "Value"=w2420) -> (w2429:T14)
          n906 = Bundle By Name(cluster=w2432, "PointForOverlays.Points.Points"=w2419, "Measurment Name"=w2431, "Measurment Type"="LineSeg", "Measurment Subtype"="PointToVirtualLine", "Result"=w2420) -> (w2430:T12)
        }
        frame "SpanOverTeeth" {
          w2461 = T14 {"VariableName"="", "VariableType"="", "Co-sys Reference"={"Base Co-sys Reference"={"Origin"={"X"=0.0, "Y"=0.0}, "Angle (deg)"=0.0, "Axis Reference"=0, "Scale"=0.0}, "New Co-sys Reference"={"Origin"={"X"=0.0, "Y"=0.0}, "Angle (deg)"=0.0, "Axis Reference"=0, "Scale"=0.0}}, "PointArray"=[], "Line Array"=[], "CircleArrayOUT"=[], "TPDetails"={"DistanceInfo"={"X"=0.0, "Y"=0.0, "X'"=0.0, "Y'"=0.0, "DX"=0.0, "DY"=0.0, "Distance Type"=""}, "Feature and Datum details"=[]}, "Value"=[], "Display Name"=0.0, "ROIArray"=[], "Update ROI "=FALSE}  # AlgoOut
          # "Point to Point"
          n907 = Index Array(array=w2454) -> (element=w2453:T42)  [unwired: 1 in]
          n908 = Index Array(array=w2449) -> (element=w2448:T26)  [unwired: 1 in]
          n909 = Unbundle By Name(w2452) -> ("ROI"=w2447:T47, "Edge Options"=w2445:T5)  [unwired: 1 out]
          n910 = Unbundle By Name(w2453) -> ("Captured Image"=w2450:T3)
          n911 = Unbundle By Name(w2448) -> ("CircleDetected.Center (Pixels)"=w2444:cluster{"X":sgl, "Y":sgl}, "CircleDetected.Radius (Pixels)"=w2443:dbl)
          n912 = call "IMAQ Convert ROI to Line"("ROI Descriptor"=w2447) -> ("Line"=w2446:T36)  [unwired: 8 in, 1 out]
          n913 = call "span over teeth.vi"("image in"=w2450, "input Line"=w2446, "Edge Options"=w2445, "Reference Circle Center"=w2444, "Requred Dia in mm"=w2443, "Calibrated Image"=w2442, "conversion factor\nY/N"=w2436, "error in (no error)"=w2440, "conversion\nfactor"=w2441) -> ("Line overlay"=w2438:cluster{"X":sgl, "Y":sgl}[], "distance in mm"=w2439:dbl, "error out"=w2437:errorcluster)  [unwired: 16 in]
          n914 = Build Array(w2439) -> (w2451:dbl[])
          n915 = Bundle By Name(cluster=w2461, "VariableName"=w2457, "VariableType"="Value", "Value"=w2451) -> (w2455:T14)
          n916 = Bundle By Name(cluster=w2458, "PointForOverlays.Points.Points"=w2438, "Measurment Name"=w2457, "Measurment Type"="LineSeg", "Result"=w2451) -> (w2456:T12)
        }
        frame "----Rect Dect----" {
        }
        frame "RectangleDetect" {
          w2482 = 400.0  # Minimum match score
          w2493 = T14 {"VariableName"="", "VariableType"="", "Co-sys Reference"={"Base Co-sys Reference"={"Origin"={"X"=0.0, "Y"=0.0}, "Angle (deg)"=0.0, "Axis Reference"=0, "Scale"=0.0}, "New Co-sys Reference"={"Origin"={"X"=0.0, "Y"=0.0}, "Angle (deg)"=0.0, "Axis Reference"=0, "Scale"=0.0}}, "PointArray"=[], "Line Array"=[], "CircleArrayOUT"=[], "TPDetails"={"DistanceInfo"={"X"=0.0, "Y"=0.0, "X'"=0.0, "Y'"=0.0, "DX"=0.0, "DY"=0.0, "Distance Type"=""}, "Feature and Datum details"=[]}, "Value"=[], "Display Name"=0.0, "ROIArray"=[], "Update ROI "=FALSE}  # AlgoOut
          n917 = Index Array(array=w2495, index=0) -> (element=w2496:T42)
          n918 = Unbundle By Name(w2489) -> ("Shape Detection Settings"=w2484:T63, "Measurement Overlay Enabled"=w2483:bool, "ROI Overlay Enabled"=w2488:bool, "ROI"=w2481:T47)
          n919 = Unbundle By Name(w2496) -> ("Captured Image"=w2475:T3)
          n920 = case shown="True" w2488 {
            tunnel: w2487 -> [w2510 w2516]
            tunnel: [w2510 w2515] -> w2486
            tunnel: w2475 -> [w2511 w2514]
            tunnel: [w2511 w2513] -> w2485
            tunnel: w2481 -> [_ w2512]
            frame False {
            }
            frame True {
              n921 = call "IMAQ Overlay ROI"("error in (no error)"=w2516, "ROI Descriptor"=w2512, "Image"=w2514) -> ("error out"=w2515:errorcluster, "Image Out"=w2513:T3)  [unwired: 7 in]
            }
          }
          n922 = call "Rectangle_detect_4_ROI_int.vi"("Image Out"=w2485, "Minimum match score"=w2482, "ROI Descriptor"=w2481, "Shape Detection Settings"=w2484, "Measurement Overlay Enabled"=w2483, "error in (no error)"=w2486, "Calibrated Image"=w2478) -> ("Line Detection (Height_Width)"=w2477:T64, "Height & Width"=w2467:sgl[], "error out"=w2474:errorcluster)  [unwired: 6 in]
          n923 = for {
            tunnel: w2477 -> [w2506] mode=indexing
            tunnel: [w2505] -> w2476 mode=indexing
            tunnel: w2475 -> [w2504]
            tunnel: [w2499] -> w2473
            tunnel: w2474 -> [w2499]
            tunnel: [w2498] -> w2471 mode=indexing
            tunnel: [w2497] -> w2472 mode=indexing
            n924 = Unbundle By Name(w2506) -> ("Point1 (Pixels)"=w2509:cluster{"X":sgl, "Y":sgl}, "Point2 (Pixels)"=w2508:cluster{"X":sgl, "Y":sgl})
            n925 = call "point_within_img.vi"("Image"=w2504, "Point"=w2509) -> ("Point"=w2503:cluster{"Point X":dbl, "Point Y":dbl})  [unwired: 7 in, 2 out]
            n926 = call "point_within_img.vi"("Image"=w2504, "Point"=w2508) -> ("Point"=w2501:cluster{"Point X":dbl, "Point Y":dbl})  [unwired: 7 in, 2 out]
            n927 = call "FEATURE_DETECTED.vi"("Point"=w2503) -> ("s? t:f"=w2502:cluster{"X":dbl, "Y":dbl}, "x .and. y?"=w2497:bool)  [unwired: 8 in, 1 out]
            n928 = call "FEATURE_DETECTED.vi"("Point"=w2501) -> ("s? t:f"=w2500:cluster{"X":dbl, "Y":dbl}, "x .and. y?"=w2498:bool)  [unwired: 8 in, 1 out]
            n929 = Bundle(cluster=T33 {"Point 1 (Pixel)"={"X"=0.0, "Y"=0.0}, "Point 2 (Pixel)"={"X"=0.0, "Y"=0.0}}, "Point 1 (Pixel)"=w2502, "Point 2 (Pixel)"=w2500) -> (w2505:T33)
          }
          n930 = And Array Elements(Boolean array=w2472) -> (logical AND=w2470:bool)
          n931 = And Array Elements(Boolean array=w2471) -> (logical AND=w2469:bool)
          n932 = Or(x=w2470, y=w2469) -> (x .or. y?=w2468:bool)
          n933 = Select(t=sgl[] [nan], s=w2468, f=w2467) -> (s? t:f=w2465:sgl[])
          n934 = Bundle By Name(cluster=w2479, "Measurment Type"="lineSeg", "Measurment Name"=w2492, "PointForOverlays.Line"=w2476) -> (w2480:T12)
          n935 = Bundle By Name(cluster=w2493, "VariableName"=w2492, "VariableType"="Value", "Value"=w2465) -> (w2490:T14)
        }
        frame "----angle measurements----" {
        }
        frame "angle2Lines" {
          w2550 = T14 {"VariableName"="", "VariableType"="", "Co-sys Reference"={"Base Co-sys Reference"={"Origin"={"X"=0.0, "Y"=0.0}, "Angle (deg)"=0.0, "Axis Reference"=0, "Scale"=0.0}, "New Co-sys Reference"={"Origin"={"X"=0.0, "Y"=0.0}, "Angle (deg)"=0.0, "Axis Reference"=0, "Scale"=0.0}}, "PointArray"=[], "Line Array"=[], "CircleArrayOUT"=[], "TPDetails"={"DistanceInfo"={"X"=0.0, "Y"=0.0, "X'"=0.0, "Y'"=0.0, "DX"=0.0, "DY"=0.0, "Distance Type"=""}, "Feature and Datum details"=[]}, "Value"=[], "Display Name"=0.0, "ROIArray"=[], "Update ROI "=FALSE}  # AlgoOut
          n936 = Index Array(array=w2539) -> (element #1=w2541:T23, element #2=w2540:T23)  [unwired: 2 in]
          n937 = Index Array(array=w2526) -> (element=w2523:sgl)  [unwired: 1 in]
          n938 = Array Size(array=w2539) -> (size(s)=w2538:i32)
          n939 = Unbundle By Name(w2541) -> ("Line"=w2536:T24)
          n940 = Unbundle By Name(w2540) -> ("Line"=w2535:T24)
          n941 = Equal?(x=w2538, y=2) -> (x = y?=w2528:bool)
          n942 = Not Equal?(x=w2536, y=w2535) -> (x != y?=w2534:T49)
          n943 = Unbundle By Name(w2534) -> ("Point 1.X"=w2533:bool, "Point 1.Y"=w2532:bool, "Point 2.X"=w2531:bool, "Point 2.Y"=w2530:bool)
          n944 = Compound Arithmetic op=OR(w2533, w2532, w2531, w2530) -> (w2529:bool)
          n945 = And(x=w2529, y=w2528) -> (x .and. y?=w2527:bool)
          n946 = case shown="True" w2527 {
            tunnel: w2551 -> [w2564 w2570]
            tunnel: [nan ("value") w2569] -> w2524
            tunnel: [w2564 w2568] -> w2544
            tunnel: w2536 -> [_ w2567]
            tunnel: w2535 -> [_ w2566]
            tunnel: [T34 {"Point 1"={"X"=0.0, "Y"=0.0}, "Point 2"={"X"=0.0, "Y"=0.0}, "vertex"={"X"=0.0, "Y"=0.0}, "Point 1a"={"X"=0.0, "Y"=0.0}, "Point 2a"={"X"=0.0, "Y"=0.0}, "line1Point1"={"X"=0.0, "Y"=0.0}, "line1Point2"={"X"=0.0, "Y"=0.0}, "line2Point1"={"X"=0.0, "Y"=0.0}, "line2Point2"={"X"=0.0, "Y"=0.0}, "Angle DMS mode"=FALSE} ("Angle") w2565] -> w2519
            frame False {
            }
            frame True {
              n947 = call "angleBetweenTwoLines.vi"("error in (no error)"=w2570, "Line2"=w2566, "Line1"=w2567) -> ("error out"=w2568:errorcluster, "value"=w2569:dbl, "Angle"=w2565:T34)  [unwired: 6 in]
            }
          }
          n948 = Greater Than 0?(x=w2523) -> (x > 0?=w2522:bool)
          n949 = case shown="True" w2522 {
            tunnel: [w2553 w2558] -> w2525
            tunnel: w2524 -> [w2553 w2557]
            tunnel: w2523 -> [_ w2556]
            tunnel: ["theta" ("Angle type") w2555] -> w2520
            frame False {
            }
            frame True {
              n950 = To Unsigned Long Integer(number=w2556) -> (unsigned 32bit integer=w2554:u32)
              n951 = case shown="360" w2554 {
                tunnel: ["theta" ("Angle type") "360-theta" ("Angle type") "180-theta" ("Angle type")] -> w2555
                frame Default {
                }
                frame 360 {
                }
                frame 180 {
                }
              }
              n952 = Subtract(x=w2556, y=w2557) -> (x-y=w2558:dbl)
            }
          }
          n953 = Build Array(w2525) -> (w2547:dbl[])
          n954 = Build Array(w2519) -> (w2521:T65)
          n955 = Bundle By Name(cluster=w2550, "VariableName"=w2546, "VariableType"="Angle", "Value"=w2547) -> (w2548:T14)
          n956 = Bundle By Name(cluster=w2542, "Measurment Type"="angle", "Measurment Name"=w2546, "PointForOverlays.Angle"=w2521, "Measurment Subtype"=w2520) -> (w2543:T12)
        }
        frame "angle3Points" {
          w2582 = cluster{"X":sgl, "Y":sgl} {"X"=nan, "Y"=nan} ("CircleDetected.Center (Pixels)")
          w2612 = T14 {"VariableName"="", "VariableType"="", "Co-sys Reference"={"Base Co-sys Reference"={"Origin"={"X"=0.0, "Y"=0.0}, "Angle (deg)"=0.0, "Axis Reference"=0, "Scale"=0.0}, "New Co-sys Reference"={"Origin"={"X"=0.0, "Y"=0.0}, "Angle (deg)"=0.0, "Axis Reference"=0, "Scale"=0.0}}, "PointArray"=[], "Line Array"=[], "CircleArrayOUT"=[], "TPDetails"={"DistanceInfo"={"X"=0.0, "Y"=0.0, "X'"=0.0, "Y'"=0.0, "DX"=0.0, "DY"=0.0, "Distance Type"=""}, "Feature and Datum details"=[]}, "Value"=[], "Display Name"=0.0, "ROIArray"=[], "Update ROI "=FALSE}  # AlgoOut
          # "finds the angle between three points"
          n957 = Array Size(array=w2576) -> (size(s)=w2575:i32)
          n958 = Decrement(x=w2575) -> (x-1=w2574:i32)
          n959 = Index Array(array=w2606) -> (element=w2607:T42)  [unwired: 1 in]
          n960 = Index Array(array=w2576, index=w2574) -> (element=w2577:sgl)
          n961 = Index Array(array=w2601) -> (element #1=w2598:cluster{"X":sgl, "Y":sgl}, element #2=w2597:cluster{"X":sgl, "Y":sgl}, element #3=w2596:cluster{"X":sgl, "Y":sgl})  [unwired: 3 in]
          n962 = Unbundle By Name(w2607) -> ()  [unwired: 2 out]
          n963 = Array Size(array=w2601) -> (size(s)=w2600:i32)
          n964 = Equal?(x=w2600, y=3) -> (x = y?=w2581:bool)
          n965 = Select(t=w2598, s=w2581, f=w2582) -> (s? t:f=w2593:cluster{"X":sgl, "Y":sgl})
          n966 = Select(t=w2597, s=w2581, f=w2582) -> (s? t:f=w2595:cluster{"X":sgl, "Y":sgl})
          n967 = Select(t=w2596, s=w2581, f=w2582) -> (s? t:f=w2594:cluster{"X":sgl, "Y":sgl})
          n968 = Not Equal?(x=w2593, y=w2595) -> (x != y?=w2592:cluster{"X":bool, "Y":bool})
          n969 = Not Equal?(x=w2595, y=w2594) -> (x != y?=w2591:cluster{"X":bool, "Y":bool})
          n970 = Not Equal?(x=w2594, y=w2593) -> (x != y?=w2590:cluster{"X":bool, "Y":bool})
          n971 = Unbundle By Name(w2591) -> ("X"=w2586:bool, "Y"=w2587:bool)
          n972 = Unbundle By Name(w2592) -> ("X"=w2584:bool, "Y"=w2585:bool)
          n973 = Unbundle By Name(w2590) -> ("X"=w2588:bool, "Y"=w2589:bool)
          n974 = Compound Arithmetic op=AND(w2584, w2585, w2586, w2587, w2588, w2589, w2581) -> (w2583:bool)
          n975 = case shown="True" w2583 {
            tunnel: w2613 -> [w2626 w2633]
            tunnel: [T34 {"Point 1"={"X"=0.0, "Y"=0.0}, "Point 2"={"X"=0.0, "Y"=0.0}, "vertex"={"X"=0.0, "Y"=0.0}, "Point 1a"={"X"=0.0, "Y"=0.0}, "Point 2a"={"X"=0.0, "Y"=0.0}, "line1Point1"={"X"=0.0, "Y"=0.0}, "line1Point2"={"X"=0.0, "Y"=0.0}, "line2Point1"={"X"=0.0, "Y"=0.0}, "line2Point2"={"X"=0.0, "Y"=0.0}, "Angle DMS mode"=FALSE} ("Angle") w2627] -> w2572
            tunnel: w2593 -> [_ w2632]
            tunnel: w2595 -> [_ w2631]
            tunnel: w2594 -> [_ w2630]
            tunnel: [nan w2629] -> w2580
            tunnel: [w2626 w2628] -> w2604
            frame False {
            }
            frame True {
              n976 = call "angleBetween3Points.vi"("error in (no error)"=w2633, "Point 3"=w2630, "Point 2 Vertex"=w2631, "Point 1"=w2632) -> ("error out"=w2628:errorcluster, "value"=w2629:dbl, "Angle"=w2627:T34)  [unwired: 5 in]
            }
          }
          n977 = Greater Than 0?(x=w2577) -> (x > 0?=w2578:bool)
          n978 = case shown="True" w2578 {
            tunnel: [w2615 w2620] -> w2579
            tunnel: w2580 -> [w2615 w2619]
            tunnel: w2577 -> [_ w2618]
            tunnel: ["theta" ("Angle type") w2617] -> w2571
            frame False {
            }
            frame True {
              n979 = To Unsigned Long Integer(number=w2618) -> (unsigned 32bit integer=w2616:u32)
              n980 = case shown="180" w2616 {
                tunnel: ["theta" ("Angle type") "360-theta" ("Angle type") "180-theta" ("Angle type")] -> w2617
                frame Default {
                }
                frame 360 {
                }
                frame 180 {
                }
              }
              n981 = Subtract(x=w2618, y=w2619) -> (x-y=w2620:dbl)
            }
          }
          n982 = Build Array(w2572) -> (w2573:T65)
          n983 = Build Array(w2579) -> (w2609:dbl[])
          n984 = Bundle By Name(cluster=w2602, "Measurment Type"="angle", "Measurment Name"=w2608, "PointForOverlays.Angle"=w2573, "Measurment Subtype"=w2571) -> (w2603:T12)
          n985 = Bundle By Name(cluster=w2612, "VariableName"=w2608, "VariableType"="Angle", "Value"=w2609) -> (w2610:T14)
        }
        frame "----radius measurements----" {
        }
        frame "circleDiameter" {
          w2658 = T35 {"Point 1"={"X"=0.0, "Y"=0.0}, "Point 2"={"X"=0.0, "Y"=0.0}, "Center (Pixels)"={"X"=0.0, "Y"=0.0}, "Radius (Pixels)"=0.0}  # Circle
          w2669 = T14 {"VariableName"="", "VariableType"="", "Co-sys Reference"={"Base Co-sys Reference"={"Origin"={"X"=0.0, "Y"=0.0}, "Angle (deg)"=0.0, "Axis Reference"=0, "Scale"=0.0}, "New Co-sys Reference"={"Origin"={"X"=0.0, "Y"=0.0}, "Angle (deg)"=0.0, "Axis Reference"=0, "Scale"=0.0}}, "PointArray"=[], "Line Array"=[], "CircleArrayOUT"=[], "TPDetails"={"DistanceInfo"={"X"=0.0, "Y"=0.0, "X'"=0.0, "Y'"=0.0, "DX"=0.0, "DY"=0.0, "Distance Type"=""}, "Feature and Datum details"=[]}, "Value"=[], "Display Name"=0.0, "ROIArray"=[], "Update ROI "=FALSE}  # AlgoOut
          n986 = Index Array(array=w2653) -> (element=w2661:T26)  [unwired: 1 in]
          n987 = Unbundle By Name(w2661) -> ("CircleDetected.Center (Pixels)"=w2640:cluster{"X":sgl, "Y":sgl}, "CircleDetected.Radius (Pixels)"=w2639:dbl, "Start Point"=w2645:cluster{"X":sgl, "Y":sgl}, "End Point"=w2644:cluster{"X":sgl, "Y":sgl})
          n988 = Array Size(array=w2653) -> (size(s)=w2652:i32)
          n989 = Greater Or Equal?(x=w2652, y=1) -> (x >= y?=w2650:bool)
          n990 = Unbundle By Name(w2640) -> ("X"=w2641:sgl)
          n991 = Add(x=w2641, y=w2639) -> (x+y=w2643:dbl)
          n992 = Subtract(x=w2641, y=w2639) -> (x-y=w2642:dbl)
          n993 = Bundle By Name(cluster=w2640, "X"=w2643) -> (w2638:cluster{"X":sgl, "Y":sgl})
          n994 = Bundle By Name(cluster=w2640, "X"=w2642) -> (w2637:cluster{"X":sgl, "Y":sgl})
          n995 = Build Array(w2638, w2637) -> (w2636:cluster{"X":sgl, "Y":sgl}[])
          n996 = Bundle By Name(cluster=w2658, "Center (Pixels)"=w2640, "Radius (Pixels)"=w2639, "Point 1"=w2645, "Point 2"=w2644) -> (w2647:T35)
          n997 = case shown="True" w2657 {
            tunnel: w2670 -> [w2679 w2683]
            tunnel: [w2678 w2680] -> w2666
            tunnel: [w2677 w2683] -> w2665
            tunnel: w2664 -> [w2676 _]
            tunnel: w2656 -> [_ w2682]
            tunnel: w2636 -> [w2675 w2681]
            frame False {
              n998 = call "IMAQ Convert Pixel to Real World"("error in (no error)"=w2679, "Array of Pixel Coordinates"=w2675, "Calibrated Image"=w2676) -> ("error out"=w2677:errorcluster, "Array of Real World Coordinates"=w2678:cluster{"X":sgl, "Y":sgl}[])  [unwired: 3 in, 4 out]
            }
            frame True {
              n999 = Divide(x=w2681, y=w2682) -> (x/y=w2680:cluster{"X":dbl, "Y":dbl}[])
            }
          }
          n1000 = call "IMAQ Point Distances"("Points"=w2666, "error in (no error)"=w2665) -> ("Distances"=w2649:sgl[], "error out"=w2663:errorcluster)  [unwired: 3 in]
          n1001 = case shown="False" w2650 {
            tunnel: w2649 -> [_ w2674]
            tunnel: [sgl[] [nan] ("Distances") w2674] -> w2646
            tunnel: [T35 {"Point 1"={"X"=nan, "Y"=nan}, "Point 2"={"X"=nan, "Y"=nan}, "Center (Pixels)"={"X"=nan, "Y"=nan}, "Radius (Pixels)"=nan} ("Circle") w2673] -> w2648
            tunnel: w2647 -> [_ w2673]
            frame False {
            }
            frame True {
            }
          }
          n1002 = Build Array(w2648) -> (w2660:T28)
          n1003 = Bundle By Name(cluster=w2654, "Measurment Type"="circle", "Measurment Name"=w2659, "PointForOverlays.Circle"=w2660) -> (w2655:T12)
          n1004 = Bundle By Name(cluster=w2669, "VariableName"=w2659, "VariableType"="Value", "Value"=w2646) -> (w2667:T14)
        }
        frame "circleRadius" {
          w2702 = T35 {"Point 1"={"X"=0.0, "Y"=0.0}, "Point 2"={"X"=0.0, "Y"=0.0}, "Center (Pixels)"={"X"=0.0, "Y"=0.0}, "Radius (Pixels)"=0.0}  # Circle
          w2719 = T14 {"VariableName"="", "VariableType"="", "Co-sys Reference"={"Base Co-sys Reference"={"Origin"={"X"=0.0, "Y"=0.0}, "Angle (deg)"=0.0, "Axis Reference"=0, "Scale"=0.0}, "New Co-sys Reference"={"Origin"={"X"=0.0, "Y"=0.0}, "Angle (deg)"=0.0, "Axis Reference"=0, "Scale"=0.0}}, "PointArray"=[], "Line Array"=[], "CircleArrayOUT"=[], "TPDetails"={"DistanceInfo"={"X"=0.0, "Y"=0.0, "X'"=0.0, "Y'"=0.0, "DX"=0.0, "DY"=0.0, "Distance Type"=""}, "Feature and Datum details"=[]}, "Value"=[], "Display Name"=0.0, "ROIArray"=[], "Update ROI "=FALSE}  # AlgoOut
          n1005 = Index Array(array=w2694) -> (element=w2709:T26)  [unwired: 1 in]
          n1006 = Array Size(array=w2694) -> (size(s)=w2693:i32)
          n1007 = Unbundle By Name(w2709) -> ("CircleDetected.Center (Pixels)"=w2701:cluster{"X":sgl, "Y":sgl}, "CircleDetected.Radius (Pixels)"=w2686:dbl, "Start Point"=w2685:cluster{"X":sgl, "Y":sgl}, "End Point"=w2684:cluster{"X":sgl, "Y":sgl})
          n1008 = Greater Or Equal?(x=w2693, y=1) -> (x >= y?=w2691:bool)
          n1009 = Unbundle By Name(w2701) -> ("X"=w2708:sgl)
          n1010 = Add(x=w2708, y=w2686) -> (x+y=w2716:dbl)
          n1011 = Subtract(x=w2708, y=w2686) -> (x-y=w2715:dbl)
          n1012 = Bundle By Name(cluster=w2701, "X"=w2716) -> (w2707:cluster{"X":sgl, "Y":sgl})
          n1013 = Bundle By Name(cluster=w2701, "X"=w2715) -> (w2706:cluster{"X":sgl, "Y":sgl})
          n1014 = Build Array(w2707, w2706) -> (w2705:cluster{"X":sgl, "Y":sgl}[])
          n1015 = Bundle By Name(cluster=w2702, "Center (Pixels)"=w2701, "Radius (Pixels)"=w2686, "Point 1"=w2685, "Point 2"=w2684) -> (w2688:T35)
          n1016 = case shown="True" w2700 {
            tunnel: w2720 -> [w2729 w2733]
            tunnel: [w2728 w2730] -> w2714
            tunnel: [w2727 w2733] -> w2713
            tunnel: w2712 -> [w2726 _]
            tunnel: w2705 -> [w2725 w2732]
            tunnel: w2699 -> [_ w2731]
            frame False {
              n1017 = call "IMAQ Convert Pixel to Real World"("error in (no error)"=w2729, "Array of Pixel Coordinates"=w2725, "Calibrated Image"=w2726) -> ("error out"=w2727:errorcluster, "Array of Real World Coordinates"=w2728:cluster{"X":sgl, "Y":sgl}[])  [unwired: 3 in, 4 out]
            }
            frame True {
              n1018 = Divide(x=w2732, y=w2731) -> (x/y=w2730:cluster{"X":dbl, "Y":dbl}[])
            }
          }
          n1019 = call "IMAQ Point Distances"("Points"=w2714, "error in (no error)"=w2713) -> ("Distances"=w2696:sgl[], "error out"=w2711:errorcluster)  [unwired: 3 in]
          n1020 = Divide(x=w2696, y=2.0) -> (x/y=w2690:dbl[])
          n1021 = case shown="True" w2691 {
            tunnel: w2690 -> [_ w2724]
            tunnel: [sgl[] [nan] ("Distances") w2724] -> w2689
            tunnel: w2688 -> [_ w2723]
            tunnel: [T35 {"Point 1"={"X"=nan, "Y"=nan}, "Point 2"={"X"=nan, "Y"=nan}, "Center (Pixels)"={"X"=nan, "Y"=nan}, "Radius (Pixels)"=nan} ("Circle") w2723] -> w2687
            frame False {
            }
            frame True {
            }
          }
          n1022 = Build Array(w2687) -> (w2704:T28)
          n1023 = Bundle By Name(cluster=w2697, "Measurment Type"="CircleRadius", "Measurment Name"=w2703, "PointForOverlays.Circle"=w2704) -> (w2698:T12)
          n1024 = Bundle By Name(cluster=w2719, "VariableName"=w2703, "VariableType"="Value", "Value"=w2689) -> (w2717:T14)
        }
        frame "----ROI conversion----" {
        }
        frame "lineToROI" {
          w2749 = T14 {"VariableName"="", "VariableType"="", "Co-sys Reference"={"Base Co-sys Reference"={"Origin"={"X"=0.0, "Y"=0.0}, "Angle (deg)"=0.0, "Axis Reference"=0, "Scale"=0.0}, "New Co-sys Reference"={"Origin"={"X"=0.0, "Y"=0.0}, "Angle (deg)"=0.0, "Axis Reference"=0, "Scale"=0.0}}, "PointArray"=[], "Line Array"=[], "CircleArrayOUT"=[], "TPDetails"={"DistanceInfo"={"X"=0.0, "Y"=0.0, "X'"=0.0, "Y'"=0.0, "DX"=0.0, "DY"=0.0, "Distance Type"=""}, "Feature and Datum details"=[]}, "Value"=[], "Display Name"=0.0, "ROIArray"=[], "Update ROI "=FALSE}  # AlgoOut
          n1025 = Index Array(array=w2736) -> (element=w2742:T23)  [unwired: 1 in]
          n1026 = Unbundle By Name(w2742) -> ("Line.Point 1.X"=w2741:sgl, "Line.Point 1.Y"=w2740:sgl, "Line.Point 1.X"=w2739:sgl, "Line.Point 1.Y"=w2738:sgl)
          n1027 = Bundle By Name(cluster=T36 {"Start X"=0, "Start Y"=0, "End X"=0, "End Y"=0} ("Line"), "Start X"=w2741, "Start Y"=w2740, "End X"=w2739, "End Y"=w2738) -> (w2737:T36)
          n1028 = call "IMAQ Convert Line to ROI"("error in (no error)"=w2744, "Line"=w2737) -> ("error out"=w2746:errorcluster, "ROI Descriptor"=w2747:T51)  [unwired: 7 in]
          n1029 = Build Array(w2747) -> (w2745:T51[])
          n1030 = Bundle By Name(cluster=w2749, "VariableName"=w2752, "VariableType"="ROI", "ROIArray"=w2745) -> (w2751:T14)
        }
        frame "circleToRoi" {
          w2761 = T14 {"VariableName"="", "VariableType"="", "Co-sys Reference"={"Base Co-sys Reference"={"Origin"={"X"=0.0, "Y"=0.0}, "Angle (deg)"=0.0, "Axis Reference"=0, "Scale"=0.0}, "New Co-sys Reference"={"Origin"={"X"=0.0, "Y"=0.0}, "Angle (deg)"=0.0, "Axis Reference"=0, "Scale"=0.0}}, "PointArray"=[], "Line Array"=[], "CircleArrayOUT"=[], "TPDetails"={"DistanceInfo"={"X"=0.0, "Y"=0.0, "X'"=0.0, "Y'"=0.0, "DX"=0.0, "DY"=0.0, "Distance Type"=""}, "Feature and Datum details"=[]}, "Value"=[], "Display Name"=0.0, "ROIArray"=[], "Update ROI "=FALSE}  # AlgoOut
          n1031 = Index Array(array=w2758) -> (element=w2754:T26)  [unwired: 1 in]
          n1032 = Unbundle By Name(w2754) -> ("CircleDetected"=w2753:T48)
          n1033 = call "circleToRoi.vi"("error in (no error)"=w2757, "intermediateCircle"=w2753) -> ("error out"=w2755:errorcluster, "Circle_ROI"=w2756:T51)  [unwired: 8 in]
          n1034 = Build Array(w2756) -> (w2759:T51[])
          n1035 = Bundle By Name(cluster=w2761, "VariableName"=w2764, "VariableType"="ROI", "ROIArray"=w2759) -> (w2763:T14)
        }
        frame "6-4STLROI" {
          w2777 = T38 {"Left"=0, "Top"=0, "Right"=0, "Bottom"=0, "Rotation"=0.0}  # Rectangle
          w2788 = T37 {"Search Direction"=0, "Edge Options"={"Edge Polarity"=0, "Kernel Size"=0, "Width"=0, "Minimum Edge Strength"=0.0, "Interpolation Type"=enum."Zero Order", "Data Processing Method"=enum."Average"}, "Line Options"={"Number of Lines"=0, "Type"=enum."First Edge Rake", "Min. Score"=0.0, "Max. Score"=0.0, "Orientation"=0.0, "Angle Range"=0.0, "Angle Tolerance"=0.0, "Step Size"=0, "Min. SNR (db)"=0.0, "Min. Points (%)"=0.0, "Hough Iterations"=0}}  # Settings
          w2790 = T14 {"VariableName"="", "VariableType"="", "Co-sys Reference"={"Base Co-sys Reference"={"Origin"={"X"=0.0, "Y"=0.0}, "Angle (deg)"=0.0, "Axis Reference"=0, "Scale"=0.0}, "New Co-sys Reference"={"Origin"={"X"=0.0, "Y"=0.0}, "Angle (deg)"=0.0, "Axis Reference"=0, "Scale"=0.0}}, "PointArray"=[], "Line Array"=[], "CircleArrayOUT"=[], "TPDetails"={"DistanceInfo"={"X"=0.0, "Y"=0.0, "X'"=0.0, "Y'"=0.0, "DX"=0.0, "DY"=0.0, "Distance Type"=""}, "Feature and Datum details"=[]}, "Value"=[], "Display Name"=0.0, "ROIArray"=[], "Update ROI "=FALSE}  # AlgoOut
          n1036 = Index Array(array=w2791) -> (element=w2792:T42)  [unwired: 1 in]
          n1037 = Unbundle By Name(w2765) -> ("Search Direction"=w2787:u16, "Edge Options"=w2786:T5, "Line Options"=w2785:T7, "ROI"=w2767:T47, "ROI Overlay Enabled"=w2766:bool)
          n1038 = Unbundle By Name(w2792) -> ("Captured Image"=w2769:T3)
          n1039 = Bundle By Name(cluster=w2788, "Search Direction"=w2787, "Edge Options"=w2786, "Line Options"=w2785) -> (w2784:T37)
          n1040 = case shown="True" w2766 {
            tunnel: w2771 -> [w2796 w2802]
            tunnel: [w2796 w2801] -> w2770
            tunnel: w2769 -> [w2797 w2800]
            tunnel: [w2797 w2799] -> w2768
            tunnel: w2767 -> [_ w2798]
            frame False {
              # "ROI overlay  disabled"
            }
            frame True {
              # "ROI overlay  enabled"
              n1041 = call "IMAQ Overlay ROI"("error in (no error)"=w2802, "ROI Descriptor"=w2798, "Image"=w2800) -> ("error out"=w2801:errorcluster, "Image Out"=w2799:T3)  [unwired: 7 in]
            }
          }
          n1042 = call "6-4STLROI.vi"("error in (no error)"=w2770, "ROI"=w2767, "Settings"=w2784, "Image IN"=w2768) -> ("error out"=w2776:errorcluster, "STLROI"=w2778:sgl[])  [unwired: 5 in, 1 out]
          n1043 = Index Array(array=w2778) -> (element #1=w2783:sgl, element #2=w2782:sgl, element #3=w2781:sgl, element #4=w2780:sgl, element #5=w2779:sgl)  [unwired: 5 in]
          n1044 = Bundle By Name(cluster=w2777, "Left"=w2783, "Top"=w2782, "Right"=w2781, "Bottom"=w2780, "Rotation"=w2779) -> (w2774:T38)
          n1045 = call "IMAQ Convert Rectangle to ROI"("error in (no error)"=w2776, "Rectangle"=w2774) -> ("error out"=w2775:errorcluster, "ROI Descriptor"=w2773:T51)  [unwired: 7 in]
          n1046 = Build Array(w2773) -> (w2772:T51[])
          n1047 = Bundle By Name(cluster=w2790, "VariableName"=w2795, "VariableType"="ROI", "ROIArray"=w2772) -> (w2794:T14)
        }
        frame "2-STLROI" {
          w2815 = T38 {"Left"=0, "Top"=0, "Right"=0, "Bottom"=0, "Rotation"=0.0}  # Rectangle
          w2825 = T37 {"Search Direction"=0, "Edge Options"={"Edge Polarity"=0, "Kernel Size"=0, "Width"=0, "Minimum Edge Strength"=0.0, "Interpolation Type"=enum."Zero Order", "Data Processing Method"=enum."Average"}, "Line Options"={"Number of Lines"=0, "Type"=enum."First Edge Rake", "Min. Score"=0.0, "Max. Score"=0.0, "Orientation"=0.0, "Angle Range"=0.0, "Angle Tolerance"=0.0, "Step Size"=0, "Min. SNR (db)"=0.0, "Min. Points (%)"=0.0, "Hough Iterations"=0}}  # Settings
          w2828 = T14 {"VariableName"="", "VariableType"="", "Co-sys Reference"={"Base Co-sys Reference"={"Origin"={"X"=0.0, "Y"=0.0}, "Angle (deg)"=0.0, "Axis Reference"=0, "Scale"=0.0}, "New Co-sys Reference"={"Origin"={"X"=0.0, "Y"=0.0}, "Angle (deg)"=0.0, "Axis Reference"=0, "Scale"=0.0}}, "PointArray"=[], "Line Array"=[], "CircleArrayOUT"=[], "TPDetails"={"DistanceInfo"={"X"=0.0, "Y"=0.0, "X'"=0.0, "Y'"=0.0, "DX"=0.0, "DY"=0.0, "Distance Type"=""}, "Feature and Datum details"=[]}, "Value"=[], "Display Name"=0.0, "ROIArray"=[], "Update ROI "=FALSE}  # AlgoOut
          n1048 = Unbundle By Name(w2826) -> ("Search Direction"=w2824:u16, "Edge Options"=w2823:T5, "Line Options"=w2822:T7, "ROI"=w2804:T47, "ROI Overlay Enabled"=w2803:bool)  [unwired: 1 out]
          n1049 = Index Array(array=w2829) -> (element=w2830:T42)  [unwired: 1 in]
          n1050 = Unbundle By Name(w2830) -> ("Captured Image"=w2806:T3)
          n1051 = Bundle By Name(cluster=w2825, "Search Direction"=w2824, "Edge Options"=w2823, "Line Options"=w2822) -> (w2821:T37)
          n1052 = case shown="True" w2803 {
            tunnel: w2808 -> [w2834 w2840]
            tunnel: [w2834 w2839] -> w2807
            tunnel: w2806 -> [w2835 w2838]
            tunnel: [w2835 w2837] -> w2805
            tunnel: w2804 -> [_ w2836]
            frame False {
              # "ROI overlay disabled"
            }
            frame True {
              # "ROI overlay enabled"
              n1053 = call "IMAQ Overlay ROI"("error in (no error)"=w2840, "ROI Descriptor"=w2836, "Image"=w2838) -> ("error out"=w2839:errorcluster, "Image Out"=w2837:T3)  [unwired: 7 in]
            }
          }
          n1054 = call "2STLROI.vi"("error in (no error)"=w2807, "ROI"=w2804, "Settings"=w2821, "Image IN"=w2805) -> ("error out"=w2811:errorcluster, "STLROI"=w2812:sgl[])  [unwired: 5 in, 1 out]
          n1055 = Index Array(array=w2812) -> (element #1=w2820:sgl, element #2=w2819:sgl, element #3=w2818:sgl, element #4=w2817:sgl, element #5=w2816:sgl)  [unwired: 5 in]
          n1056 = Bundle By Name(cluster=w2815, "Left"=w2820, "Top"=w2819, "Right"=w2818, "Bottom"=w2817, "Rotation"=w2816) -> (w2814:T38)
          n1057 = call "IMAQ Convert Rectangle to ROI"("error in (no error)"=w2811, "Rectangle"=w2814) -> ("error out"=w2810:errorcluster, "ROI Descriptor"=w2813:T51)  [unwired: 7 in]
          n1058 = Build Array(w2813) -> (w2809:T51[])
          n1059 = Bundle By Name(cluster=w2828, "VariableName"=w2833, "VariableType"="ROI", "ROIArray"=w2809) -> (w2832:T14)
        }
        frame "6-4STRROI" {
          w2853 = T38 {"Left"=0, "Top"=0, "Right"=0, "Bottom"=0, "Rotation"=0.0}  # Rectangle
          w2866 = T14 {"VariableName"="", "VariableType"="", "Co-sys Reference"={"Base Co-sys Reference"={"Origin"={"X"=0.0, "Y"=0.0}, "Angle (deg)"=0.0, "Axis Reference"=0, "Scale"=0.0}, "New Co-sys Reference"={"Origin"={"X"=0.0, "Y"=0.0}, "Angle (deg)"=0.0, "Axis Reference"=0, "Scale"=0.0}}, "PointArray"=[], "Line Array"=[], "CircleArrayOUT"=[], "TPDetails"={"DistanceInfo"={"X"=0.0, "Y"=0.0, "X'"=0.0, "Y'"=0.0, "DX"=0.0, "DY"=0.0, "Distance Type"=""}, "Feature and Datum details"=[]}, "Value"=[], "Display Name"=0.0, "ROIArray"=[], "Update ROI "=FALSE}  # AlgoOut
          n1060 = Unbundle By Name(w2864) -> ("Search Direction"=w2862:u16, "Edge Options"=w2861:T5, "Line Options"=w2860:T7, "ROI"=w2842:T47, "ROI Overlay Enabled"=w2841:bool)  [unwired: 1 out]
          n1061 = Index Array(array=w2867) -> (element=w2868:T42)  [unwired: 1 in]
          n1062 = Unbundle By Name(w2868) -> ("Captured Image"=w2843:T3)
          n1063 = Bundle By Name(cluster=T37 {"Search Direction"=0, "Edge Options"={"Edge Polarity"=0, "Kernel Size"=0, "Width"=0, "Minimum Edge Strength"=0.0, "Interpolation Type"=enum."Zero Order", "Data Processing Method"=enum."Average"}, "Line Options"={"Number of Lines"=0, "Type"=enum."First Edge Rake", "Min. Score"=0.0, "Max. Score"=0.0, "Orientation"=0.0, "Angle Range"=0.0, "Angle Tolerance"=0.0, "Step Size"=0, "Min. SNR (db)"=0.0, "Min. Points (%)"=0.0, "Hough Iterations"=0}} ("Settings"), "Search Direction"=w2862, "Edge Options"=w2861, "Line Options"=w2860) -> (w2859:T37)
          n1064 = case shown="False" w2841 {
            tunnel: w2846 -> [w2872 w2878]
            tunnel: [w2872 w2877] -> w2845
            tunnel: w2843 -> [w2873 w2876]
            tunnel: [w2873 w2875] -> w2844
            tunnel: w2842 -> [_ w2874]
            frame False {
              # "ROI overlay disabled"
            }
            frame True {
              # "ROI overlay enabled"
              n1065 = call "IMAQ Overlay ROI"("error in (no error)"=w2878, "ROI Descriptor"=w2874, "Image"=w2876) -> ("error out"=w2877:errorcluster, "Image Out"=w2875:T3)  [unwired: 7 in]
            }
          }
          n1066 = call "6-4STRROI.vi"("error in (no error)"=w2845, "ROI"=w2842, "Settings"=w2859, "Image IN"=w2844) -> ("error out"=w2850:errorcluster, "STLROI"=w2847:sgl[])  [unwired: 5 in, 1 out]
          n1067 = Index Array(array=w2847) -> (element #1=w2858:sgl, element #2=w2857:sgl, element #3=w2856:sgl, element #4=w2855:sgl, element #5=w2854:sgl)  [unwired: 5 in]
          n1068 = Bundle By Name(cluster=w2853, "Left"=w2858, "Top"=w2857, "Right"=w2856, "Bottom"=w2855, "Rotation"=w2854) -> (w2852:T38)
          n1069 = call "IMAQ Convert Rectangle to ROI"("error in (no error)"=w2850, "Rectangle"=w2852) -> ("error out"=w2849:errorcluster, "ROI Descriptor"=w2851:T51)  [unwired: 7 in]
          n1070 = Build Array(w2851) -> (w2848:T51[])
          n1071 = Bundle By Name(cluster=w2866, "VariableName"=w2871, "VariableType"="ROI", "ROIArray"=w2848) -> (w2870:T14)
        }
        frame "2-STRROI" {
          n1072 = Unbundle By Name(w2902) -> ("Search Direction"=w2900:u16, "Edge Options"=w2899:T5, "Line Options"=w2898:T7, "ROI Overlay Enabled"=w2880:bool, "ROI"=w2879:T47)  [unwired: 1 out]
          n1073 = Index Array(array=w2905) -> (element=w2906:T42)  [unwired: 1 in]
          n1074 = Unbundle By Name(w2906) -> ("Captured Image"=w2884:T3)
          n1075 = Bundle By Name(cluster=T37 {"Search Direction"=0, "Edge Options"={"Edge Polarity"=0, "Kernel Size"=0, "Width"=0, "Minimum Edge Strength"=0.0, "Interpolation Type"=enum."Zero Order", "Data Processing Method"=enum."Average"}, "Line Options"={"Number of Lines"=0, "Type"=enum."First Edge Rake", "Min. Score"=0.0, "Max. Score"=0.0, "Orientation"=0.0, "Angle Range"=0.0, "Angle Tolerance"=0.0, "Step Size"=0, "Min. SNR (db)"=0.0, "Min. Points (%)"=0.0, "Hough Iterations"=0}} ("Settings"), "Search Direction"=w2900, "Edge Options"=w2899, "Line Options"=w2898) -> (w2897:T37)
          n1076 = case shown="False" w2880 {
            tunnel: w2882 -> [w2910 w2916]
            tunnel: [w2910 w2915] -> w2881
            tunnel: w2884 -> [w2911 w2914]
            tunnel: [w2911 w2913] -> w2883
            tunnel: w2879 -> [_ w2912]
            frame False {
              # "ROI overlay disabled"
            }
            frame True {
              # "ROI overlay enabled"
              n1077 = call "IMAQ Overlay ROI"("error in (no error)"=w2916, "ROI Descriptor"=w2912, "Image"=w2914) -> ("error out"=w2915:errorcluster, "Image Out"=w2913:T3)  [unwired: 7 in]
            }
          }
          n1078 = call "2STRROI.vi"("error in (no error)"=w2881, "ROI"=w2879, "Settings"=w2897, "Image IN"=w2883) -> ("error out"=w2888:errorcluster, "STLROI"=w2885:sgl[])  [unwired: 5 in, 1 out]
          n1079 = Index Array(array=w2885) -> (element #1=w2896:sgl, element #2=w2895:sgl, element #3=w2894:sgl, element #4=w2893:sgl, element #5=w2892:sgl)  [unwired: 5 in]
          n1080 = Bundle By Name(cluster=T38 {"Left"=0, "Top"=0, "Right"=0, "Bottom"=0, "Rotation"=0.0} ("Rectangle"), "Left"=w2896, "Top"=w2895, "Right"=w2894, "Bottom"=w2893, "Rotation"=w2892) -> (w2890:T38)
          n1081 = call "IMAQ Convert Rectangle to ROI"("error in (no error)"=w2888, "Rectangle"=w2890) -> ("error out"=w2887:errorcluster, "ROI Descriptor"=w2889:T51)  [unwired: 7 in]
          n1082 = Build Array(w2889) -> (w2886:T51[])
          n1083 = Bundle By Name(cluster=T14 {"VariableName"="", "VariableType"="", "Co-sys Reference"={"Base Co-sys Reference"={"Origin"={"X"=0.0, "Y"=0.0}, "Angle (deg)"=0.0, "Axis Reference"=0, "Scale"=0.0}, "New Co-sys Reference"={"Origin"={"X"=0.0, "Y"=0.0}, "Angle (deg)"=0.0, "Axis Reference"=0, "Scale"=0.0}}, "PointArray"=[], "Line Array"=[], "CircleArrayOUT"=[], "TPDetails"={"DistanceInfo"={"X"=0.0, "Y"=0.0, "X'"=0.0, "Y'"=0.0, "DX"=0.0, "DY"=0.0, "Distance Type"=""}, "Feature and Datum details"=[]}, "Value"=[], "Display Name"=0.0, "ROIArray"=[], "Update ROI "=FALSE} ("AlgoOut"), "VariableName"=w2909, "VariableType"="ROI", "ROIArray"=w2886) -> (w2908:T14)
        }
        frame "findTopROI" {
          w2925 = T14 {"VariableName"="", "VariableType"="", "Co-sys Reference"={"Base Co-sys Reference"={"Origin"={"X"=0.0, "Y"=0.0}, "Angle (deg)"=0.0, "Axis Reference"=0, "Scale"=0.0}, "New Co-sys Reference"={"Origin"={"X"=0.0, "Y"=0.0}, "Angle (deg)"=0.0, "Axis Reference"=0, "Scale"=0.0}}, "PointArray"=[], "Line Array"=[], "CircleArrayOUT"=[], "TPDetails"={"DistanceInfo"={"X"=0.0, "Y"=0.0, "X'"=0.0, "Y'"=0.0, "DX"=0.0, "DY"=0.0, "Distance Type"=""}, "Feature and Datum details"=[]}, "Value"=[], "Display Name"=0.0, "ROIArray"=[], "Update ROI "=FALSE}  # AlgoOut
          w2928 = T38 {"Left"=0, "Top"=0, "Right"=0, "Bottom"=0, "Rotation"=0.0}  # Rectangle
          n1084 = Index Array(array=w2937) -> (element=w2938:T42)  [unwired: 1 in]
          n1085 = Unbundle By Name(w2940) -> ("ROI"=w2934:T47, "Edge Options"=w2935:T5)
          n1086 = Unbundle By Name(w2938) -> ("Captured Image"=w2936:T3)
          n1087 = call "computeTopROI.vi"("error in (no error)"=w2939, "Edge Options"=w2935, "ROI Descriptor"=w2934, "Image IN"=w2936) -> ("error out"=w2927:errorcluster, "TopROI"=w2920:sgl[])  [unwired: 5 in, 1 out]
          n1088 = Index Array(array=w2920) -> (element #1=w2933:sgl, element #2=w2932:sgl, element #3=w2931:sgl, element #4=w2930:sgl, element #5=w2929:sgl)  [unwired: 5 in]
          n1089 = Bundle By Name(cluster=w2928, "Left"=w2933, "Top"=w2932, "Right"=w2931, "Bottom"=w2930, "Rotation"=w2929) -> (w2926:T38)
          n1090 = call "IMAQ Convert Rectangle to ROI"("error in (no error)"=w2927, "Rectangle"=w2926) -> ("error out"=w2923:errorcluster, "ROI Descriptor"=w2922:T51)  [unwired: 7 in]
          n1091 = Build Array(w2922) -> (w2921:T51[])
          n1092 = Bundle By Name(cluster=w2925, "VariableName"=w2919, "VariableType"="ROI", "ROIArray"=w2921) -> (w2918:T14)
        }
        frame "----computation Will not work----" {
        }
        frame "dimoverpins" {
          w2965 = T14 {"VariableName"="", "VariableType"="", "Co-sys Reference"={"Base Co-sys Reference"={"Origin"={"X"=0.0, "Y"=0.0}, "Angle (deg)"=0.0, "Axis Reference"=0, "Scale"=0.0}, "New Co-sys Reference"={"Origin"={"X"=0.0, "Y"=0.0}, "Angle (deg)"=0.0, "Axis Reference"=0, "Scale"=0.0}}, "PointArray"=[], "Line Array"=[], "CircleArrayOUT"=[], "TPDetails"={"DistanceInfo"={"X"=0.0, "Y"=0.0, "X'"=0.0, "Y'"=0.0, "DX"=0.0, "DY"=0.0, "Distance Type"=""}, "Feature and Datum details"=[]}, "Value"=[], "Display Name"=0.0, "ROIArray"=[], "Update ROI "=FALSE}  # AlgoOut
          n1093 = Unbundle By Name(w2959) -> ("Edge Options"=w2954:T5, "Line Options"=w2953:T7)  [unwired: 1 out]
          n1094 = Array Subset(array=w2950, index=14, length=36) -> (w2948:cluster{"X":sgl, "Y":sgl}[])
          n1095 = Index Array(array=w2961) -> (element=w2962:T42)  [unwired: 1 in]
          n1096 = Bundle By Name(cluster=T39 {"Options"={"Search Direction"=0, "Edge Options"={"Edge Polarity"=2, "Kernel Size"=17, "Width"=5, "Minimum Edge Strength"=50.0, "Interpolation Type"=enum."Zero Order", "Data Processing Method"=enum."Average"}, "Show Search Area"=TRUE, "Show Search Lines"=TRUE, "Show Edges Found"=TRUE, "Show Result"=TRUE, "Search Area Color"=65280, "Search Lines Color"=255, "Edge Locations Color"=16776960, "Result Color"=16711680, "Overlay Group Name"=""}, "Line Fit Options"={"Number of Lines"=1, "Type"=enum."First Edge Rake", "Min. Score"=20.0, "Max. Score"=1000.0, "Orientation"=0.0, "Angle Range"=10.0, "Angle Tolerance"=1.0, "Step Size"=11, "Min. SNR (db)"=3.0, "Min. Points (%)"=25.0, "Hough Iterations"=5}} ("Settings"), "Options.Edge Options"=w2954, "Line Fit Options"=w2953) -> (w2952:T39)
          n1097 = Unbundle By Name(w2962) -> ("Captured Image"=w2958:T3)
          n1098 = call "dimOverPins.vi"("Settings"=w2952, "error in (no error)"=w2957, "edgePoints"=w2948, "Image in"=w2958) -> ("error out"=w2956:errorcluster, "Point array"=w2945:cluster{"X":sgl, "Y":sgl}[], "Image Out"=w2951:T3)  [unwired: 5 in]
          n1099 = Bundle By Name(cluster=w2943, "Measurment Type"="point", "Measurment Name"=w2964, "PointForOverlays.Points.Points"=w2945) -> (w2944:T12)
          n1100 = Bundle By Name(cluster=w2965, "VariableName"=w2964, "VariableType"="Point", "PointArray"=w2945) -> (w2966:T14)
          n1101 = case shown="True" w2963 {
            tunnel: w2951 -> [w2969 w2971]
            tunnel: [w2969 w2972] -> _
            tunnel: w2956 -> [w2968 w2973]
            tunnel: [w2968 w2974] -> w2960
            tunnel: w2945 -> [_ w2970]
            frame False {
              # "Measurement overlay disabled"
            }
            frame True {
              # "Measurement overlay enabled"
              n1102 = call "IMAQ Overlay Points"("error in (no error)"=w2973, "Array of Points"=w2970, "Image"=w2971) -> ("error out"=w2974:errorcluster, "Image Out"=w2972:T3)  [unwired: 7 in]
            }
          }
        }
        frame "MovePoints" {
          w2982 = T66 {"XL"=62.68532, "YL"=74.445, "Xmi"=0.0, "Ymi"=0.0}  # Calibration Constants
          w2990 = T14 {"VariableName"="", "VariableType"="", "Co-sys Reference"={"Base Co-sys Reference"={"Origin"={"X"=0.0, "Y"=0.0}, "Angle (deg)"=0.0, "Axis Reference"=0, "Scale"=0.0}, "New Co-sys Reference"={"Origin"={"X"=0.0, "Y"=0.0}, "Angle (deg)"=0.0, "Axis Reference"=0, "Scale"=0.0}}, "PointArray"=[], "Line Array"=[], "CircleArrayOUT"=[], "TPDetails"={"DistanceInfo"={"X"=0.0, "Y"=0.0, "X'"=0.0, "Y'"=0.0, "DX"=0.0, "DY"=0.0, "Distance Type"=""}, "Feature and Datum details"=[]}, "Value"=[], "Display Name"=0.0, "ROIArray"=[], "Update ROI "=FALSE}  # AlgoOut
          # "will not work"
          n1103 = Index Array(array=w2986) -> (element #1=w2985:sgl, element #2=w2984:sgl, element #3=w2981:sgl, element #4=w2980:sgl, element #5=w2978:sgl)  [unwired: 5 in]
          n1104 = Bundle By Name(cluster=w2982, "XL"=w2985, "YL"=w2984, "Xmi"=w2981, "Ymi"=w2980) -> (w2979:T66)
          n1105 = call "image to table axis.vi"("error in (no error)"=w2977, "Theta"=w2978, "Calibration Constants"=w2979, "Points"=w2983) -> ("error out"=w2976:errorcluster, "output cluster"=w2975:cluster{"X":dbl, "Y\n":dbl}[])  [unwired: 6 in]
          n1106 = Bundle By Name(cluster=w2990, "VariableName"=w2989, "VariableType"="Point", "PointArray"=w2975) -> (w2988:T14)
        }
        frame "2DPlaneFit" {
          w2999 = T14 {"VariableName"="", "VariableType"="", "Co-sys Reference"={"Base Co-sys Reference"={"Origin"={"X"=0.0, "Y"=0.0}, "Angle (deg)"=0.0, "Axis Reference"=0, "Scale"=0.0}, "New Co-sys Reference"={"Origin"={"X"=0.0, "Y"=0.0}, "Angle (deg)"=0.0, "Axis Reference"=0, "Scale"=0.0}}, "PointArray"=[], "Line Array"=[], "CircleArrayOUT"=[], "TPDetails"={"DistanceInfo"={"X"=0.0, "Y"=0.0, "X'"=0.0, "Y'"=0.0, "DX"=0.0, "DY"=0.0, "Distance Type"=""}, "Feature and Datum details"=[]}, "Value"=[], "Display Name"=0.0, "ROIArray"=[], "Update ROI "=FALSE}  # AlgoOut
          n1107 = call "Find 2D Best fit Plane.vi"("error in (no error)"=w3000, "Arrray of Datum Points"=w3001, "Array Of Z Points"=w2992) -> ("error out"=w2994:errorcluster, "Plane Coefficients"=w2997:dbl[])  [unwired: 7 in]
          n1108 = Bundle By Name(cluster=w2999, "VariableName"=w2993, "VariableType"="Values", "Value"=w2997) -> (w2995:T14)
        }
        frame "Distancefromaplane" {
          w3010 = T14 {"VariableName"="", "VariableType"="", "Co-sys Reference"={"Base Co-sys Reference"={"Origin"={"X"=0.0, "Y"=0.0}, "Angle (deg)"=0.0, "Axis Reference"=0, "Scale"=0.0}, "New Co-sys Reference"={"Origin"={"X"=0.0, "Y"=0.0}, "Angle (deg)"=0.0, "Axis Reference"=0, "Scale"=0.0}}, "PointArray"=[], "Line Array"=[], "CircleArrayOUT"=[], "TPDetails"={"DistanceInfo"={"X"=0.0, "Y"=0.0, "X'"=0.0, "Y'"=0.0, "DX"=0.0, "DY"=0.0, "Distance Type"=""}, "Feature and Datum details"=[]}, "Value"=[], "Display Name"=0.0, "ROIArray"=[], "Update ROI "=FALSE}  # AlgoOut
          n1109 = Array Size(array=w3006) -> (size(s)=w3005:i32)
          n1110 = Array Subset(array=w3016, index=4, length=w3005) -> (w3014:sgl[])
          n1111 = call "CombiningXY&Z.vi"("error in (no error)"=w3012, "Z"=w3014, "PointArray"=w3006) -> ("error out"=w3011:errorcluster, "XYZ Array"=w3013:cluster{"X":dbl, "Y":dbl, "Z":dbl}[])  [unwired: 7 in]
          n1112 = Array Subset "Array Subset"(array=w3016, index=0, length=4) -> (w3017:sgl[])
          n1113 = call "Distance From a Plane.vi"("error in (no error)"=w3011, "Arrray of Datum Points"=w3013, "Plane Coefficients"=w3017) -> ("error out"=w3002:errorcluster, "Array of Distances"=w3003:dbl[])  [unwired: 7 in]
          n1114 = Bundle By Name(cluster=w3010, "VariableName"=w3004, "VariableType"="Value", "Value"=w3003) -> (w3008:T14)
        }
        frame "PointsDepthDifference" {
          w3031 = T14 {"VariableName"="", "VariableType"="", "Co-sys Reference"={"Base Co-sys Reference"={"Origin"={"X"=0.0, "Y"=0.0}, "Angle (deg)"=0.0, "Axis Reference"=0, "Scale"=0.0}, "New Co-sys Reference"={"Origin"={"X"=0.0, "Y"=0.0}, "Angle (deg)"=0.0, "Axis Reference"=0, "Scale"=0.0}}, "PointArray"=[], "Line Array"=[], "CircleArrayOUT"=[], "TPDetails"={"DistanceInfo"={"X"=0.0, "Y"=0.0, "X'"=0.0, "Y'"=0.0, "DX"=0.0, "DY"=0.0, "Distance Type"=""}, "Feature and Datum details"=[]}, "Value"=[], "Display Name"=0.0, "ROIArray"=[], "Update ROI "=FALSE}  # AlgoOut
          n1115 = Index Array(array=w3025) -> (element #1=w3024:sgl, element #2=w3023:sgl)  [unwired: 2 in]
          n1116 = Subtract(x=w3024, y=w3023) -> (x-y=w3022:sgl)
          n1117 = Absolute Value(x=w3022) -> (abs(x)=w3021:sgl)
          n1118 = Build Array(w3021) -> (w3020:sgl[])
          n1119 = Bundle By Name(cluster=w3031, "VariableName"=w3027, "VariableType"="Value", "Value"=w3020) -> (w3028:T14)
        }
        frame "StageToPlaneAngle" {
          w3040 = T14 {"VariableName"="", "VariableType"="", "Co-sys Reference"={"Base Co-sys Reference"={"Origin"={"X"=0.0, "Y"=0.0}, "Angle (deg)"=0.0, "Axis Reference"=0, "Scale"=0.0}, "New Co-sys Reference"={"Origin"={"X"=0.0, "Y"=0.0}, "Angle (deg)"=0.0, "Axis Reference"=0, "Scale"=0.0}}, "PointArray"=[], "Line Array"=[], "CircleArrayOUT"=[], "TPDetails"={"DistanceInfo"={"X"=0.0, "Y"=0.0, "X'"=0.0, "Y'"=0.0, "DX"=0.0, "DY"=0.0, "Distance Type"=""}, "Feature and Datum details"=[]}, "Value"=[], "Display Name"=0.0, "ROIArray"=[], "Update ROI "=FALSE}  # AlgoOut
          n1120 = call "Plane to XY stage angle.vi"("Plane equation"=w3034) -> ("Plane angle (in degrees)"=w3033:dbl)  [unwired: 10 in]
          n1121 = Build Array(w3033) -> (w3032:dbl[])
          n1122 = Bundle By Name(cluster=w3040, "VariableName"=w3036, "VariableType"="Value", "Value"=w3032) -> (w3037:T14)
        }
        frame "----Profile Measurements----" {
        }
        frame "Concentricity" {
          w3053 = T35 {"Point 1"={"X"=0.0, "Y"=0.0}, "Point 2"={"X"=0.0, "Y"=0.0}, "Center (Pixels)"={"X"=0.0, "Y"=0.0}, "Radius (Pixels)"=0.0}  # Circle
          n1123 = Index Array(array=w3061) -> (element #1=w3060:T26, element #2=w3048:T26)  [unwired: 2 in]
          n1124 = Unbundle By Name(w3060) -> ("CircleDetected.Center (Pixels)"=w3050:cluster{"X":sgl, "Y":sgl})
          n1125 = Unbundle By Name(w3048) -> ("CircleDetected.Center (Pixels)"=w3049:cluster{"X":sgl, "Y":sgl})
          n1126 = Array Size(array=w3061) -> (size(s)=w3065:i32)
          n1127 = Equal?(x=w3065, y=2) -> (x = y?=w3043:bool)
          n1128 = case shown="True" w3043 {
            tunnel: w3051 -> [w3074 w3084]
            tunnel: [w3074 w3083] -> w3071
            tunnel: w3070 -> [_ w3082]
            tunnel: w3050 -> [_ w3081]
            tunnel: w3049 -> [_ w3080]
            tunnel: [dbl[] [nan] w3078] -> w3067
            tunnel: w3063 -> [_ w3077]
            tunnel: w3062 -> [_ w3076]
            tunnel: [w3073 w3075] -> w3047
            tunnel: w3048 -> [_ w3075]
            frame False {
              w3073 = T30 {"CircleDetected"={"Center (Pixels)"={"X"=nan, "Y"=nan}, "Radius (Pixels)"=nan}, "First Edges"=[], "Indexes of Points Used"=[], "Start Point"={"X"=0.0, "Y"=0.0}, "End Point"={"X"=0.0, "Y"=0.0}}  # Circle NaN Array
            }
            frame True {
              n1129 = call "concentricity.vi"(6:"Conversion Factor"=w3077, 7:"Conversion Factor"=w3076, "error in (no error)"=w3084, "Cricle Center 1"=w3080, "Cricle Center 2"=w3081, "Calibrated Image"=w3082) -> ("error out"=w3083:errorcluster, "Concentiricty"=w3079:sgl)  [unwired: 4 in]
              n1130 = Build Array(w3079) -> (w3078:sgl[])
            }
          }
          n1131 = Unbundle By Name(w3047) -> ("CircleDetected.Center (Pixels)"=w3055:cluster{"X":dbl, "Y":dbl}, "CircleDetected.Radius (Pixels)"=w3046:dbl, "Start Point"=w3045:cluster{"X":sgl, "Y":sgl}, "End Point"=w3044:cluster{"X":sgl, "Y":sgl})
          n1132 = Bundle By Name(cluster=w3053, "Center (Pixels)"=w3055, "Radius (Pixels)"=w3046, "Point 1"=w3045, "Point 2"=w3044) -> (w3054:T35)
          n1133 = Bundle By Name(cluster=T14 {"VariableName"="", "VariableType"="", "Co-sys Reference"={"Base Co-sys Reference"={"Origin"={"X"=0.0, "Y"=0.0}, "Angle (deg)"=0.0, "Axis Reference"=0, "Scale"=0.0}, "New Co-sys Reference"={"Origin"={"X"=0.0, "Y"=0.0}, "Angle (deg)"=0.0, "Axis Reference"=0, "Scale"=0.0}}, "PointArray"=[], "Line Array"=[], "CircleArrayOUT"=[], "TPDetails"={"DistanceInfo"={"X"=0.0, "Y"=0.0, "X'"=0.0, "Y'"=0.0, "DX"=0.0, "DY"=0.0, "Distance Type"=""}, "Feature and Datum details"=[]}, "Value"=[], "Display Name"=0.0, "ROIArray"=[], "Update ROI "=FALSE} ("AlgoOut"), "VariableName"=w3052, "VariableType"="Value", "Value"=w3067) -> (w3066:T14)
          n1134 = Build Array(w3054) -> (w3058:T28)
          n1135 = Bundle By Name(cluster=w3057, "PointForOverlays.Circle"=w3058, "Measurment Type"="Concentricity", "Measurment Name"=w3052) -> (w3056:T12)
        }
        frame "Parallality" {
          n1136 = Index Array(array=w3111) -> (element=w3110:T42)  [unwired: 1 in]
          n1137 = Index Array(array=w3114) -> (element #1=w3097:T23, element #2=w3089:T23)  [unwired: 2 in]
          n1138 = Array Size(array=w3114) -> (size(s)=w3113:i32)
          n1139 = Unbundle By Name(w3110) -> ()  [unwired: 2 out]
          n1140 = Equal?(x=w3113, y=2) -> (x = y?=w3087:bool)
          n1141 = Unbundle By Name(w3089) -> ("Line"=w3094:T24)
          n1142 = Unbundle By Name(w3097) -> ("Line"=w3095:T24)
          n1143 = Not Equal?(x=w3095, y=w3094) -> (x != y?=w3096:T49)
          n1144 = Unbundle By Name(w3096) -> ("Point 1.X"=w3090:bool, "Point 1.Y"=w3091:bool, "Point 2.X"=w3092:bool, "Point 2.Y"=w3093:bool)
          n1145 = Compound Arithmetic op=OR(w3090, w3091, w3092, w3093) -> (w3088:bool)
          n1146 = And(x=w3087, y=w3088) -> (x .and. y?=w3086:bool)
          n1147 = case shown="True" w3086 {
            tunnel: w3121 -> [w3123 w3133]
            tunnel: [w3123 w3132] -> w3120
            tunnel: w3109 -> [_ w3131]
            tunnel: [nan ("Parallality") w3130] -> w3117
            tunnel: w3095 -> [_ w3129]
            tunnel: w3094 -> [_ w3128]
            tunnel: w3108 -> [_ w3127]
            tunnel: w3107 -> [_ w3126]
            tunnel: w3089 -> [_ w3125]
            tunnel: [T23 {"Line"={"Point 1"={"X"=nan, "Y"=nan}, "Point 2"={"X"=nan, "Y"=nan}}, "Straight Edges"=[], "Used Edges"=[]} ("Line") w3125] -> w3085
            frame False {
            }
            frame True {
              n1148 = call "Parallality.vi"("Calibrated Image"=w3131, "Converstion Factor"=w3126, "Line 1"=w3129, "Line 2"=w3128, "error in (no error)"=w3133, "Conversion Factor"=w3127) -> ("Parallality"=w3130:dbl, "error out"=w3132:errorcluster)  [unwired: 8 in]
            }
          }
          n1149 = Unbundle By Name(w3085) -> ("Line.Point 1"=w3106:cluster{"X":sgl, "Y":sgl}, "Line.Point 2"=w3105:cluster{"X":sgl, "Y":sgl})
          n1150 = Bundle By Name(cluster=T24 {"Point 1"={"X"=0.0, "Y"=0.0}, "Point 2"={"X"=0.0, "Y"=0.0}} ("Line"), "Point 1"=w3106, "Point 2"=w3105) -> (w3103:T24)
          n1151 = Build Array(w3103) -> (w3102:T31)
          n1152 = Bundle By Name(cluster=w3100, "PointForOverlays.Line"=w3102, "Measurment Name"=w3098, "Measurment Type"="Parallelism") -> (w3099:T12)
          n1153 = Build Array(w3117) -> (w3116:dbl[])
          n1154 = Bundle By Name(cluster=T14 {"VariableName"="", "VariableType"="", "Co-sys Reference"={"Base Co-sys Reference"={"Origin"={"X"=0.0, "Y"=0.0}, "Angle (deg)"=0.0, "Axis Reference"=0, "Scale"=0.0}, "New Co-sys Reference"={"Origin"={"X"=0.0, "Y"=0.0}, "Angle (deg)"=0.0, "Axis Reference"=0, "Scale"=0.0}}, "PointArray"=[], "Line Array"=[], "CircleArrayOUT"=[], "TPDetails"={"DistanceInfo"={"X"=0.0, "Y"=0.0, "X'"=0.0, "Y'"=0.0, "DX"=0.0, "DY"=0.0, "Distance Type"=""}, "Feature and Datum details"=[]}, "Value"=[], "Display Name"=0.0, "ROIArray"=[], "Update ROI "=FALSE} ("AlgoOut"), "VariableName"=w3098, "VariableType"="Value", "Value"=w3116) -> (w3115:T14)
        }
        frame "Straightness" {
          n1155 = Index Array(array=w3142) -> (element=w3141:T42)  [unwired: 1 in]
          n1156 = Unbundle By Name(w3141) -> ()  [unwired: 1 out]
          n1157 = Index Array(array=w3139) -> (element=w3155:T23)  [unwired: 1 in]
          n1158 = Array Size(array=w3139) -> (size(s)=w3138:i32)
          n1159 = Equal?(x=w3138, y=1) -> (x = y?=w3136:bool)
          n1160 = Unbundle By Name(w3155) -> ("Line"=w3135:T24, "Straight Edges"=w3153:T52, "Used Edges"=w3154:cluster{"Edge Information":T15[]}[])
          n1161 = case shown="True" w3136 {
            tunnel: w3159 -> [_ w3175]
            tunnel: [nan ("Final Straightness value") w3174] -> w3158
            tunnel: [w3166 w3173] -> w3157
            tunnel: w3156 -> [w3166 w3172]
            tunnel: w3154 -> [_ w3171]
            tunnel: w3153 -> [_ w3170]
            tunnel: w3152 -> [_ w3169]
            tunnel: w3151 -> [_ w3168]
            tunnel: w3135 -> [_ w3167]
            tunnel: [T24 {"Point 1"={"X"=nan, "Y"=nan}, "Point 2"={"X"=nan, "Y"=nan}} ("Line") w3167] -> w3134
            frame False {
            }
            frame True {
              n1162 = call "straightness.vi"("Calibrated Image"=w3175, "Straight Edges"=w3170, "Edge Information"=w3171, "Converstion Factor"=w3169, "Converstion Factor 2"=w3168, "error in (no error)"=w3172) -> ("Final Straightness value"=w3174:dbl, "error out"=w3173:errorcluster)  [unwired: 8 in]
            }
          }
          n1163 = Unbundle By Name(w3134) -> ("Point 1"=w3150:cluster{"X":sgl, "Y":sgl}, "Point 2"=w3149:cluster{"X":sgl, "Y":sgl})
          n1164 = Bundle By Name(cluster=T24 {"Point 1"={"X"=0.0, "Y"=0.0}, "Point 2"={"X"=0.0, "Y"=0.0}} ("Line"), "Point 1"=w3150, "Point 2"=w3149) -> (w3147:T24)
          n1165 = Build Array(w3147) -> (w3146:T31)
          n1166 = Bundle By Name(cluster=w3144, "PointForOverlays.Line"=w3146, "Measurment Name"=w3140, "Measurment Type"="Straightness") -> (w3143:T12)
          n1167 = Build Array(w3158) -> (w3161:dbl[])
          n1168 = Bundle By Name(cluster=T14 {"VariableName"="", "VariableType"="", "Co-sys Reference"={"Base Co-sys Reference"={"Origin"={"X"=0.0, "Y"=0.0}, "Angle (deg)"=0.0, "Axis Reference"=0, "Scale"=0.0}, "New Co-sys Reference"={"Origin"={"X"=0.0, "Y"=0.0}, "Angle (deg)"=0.0, "Axis Reference"=0, "Scale"=0.0}}, "PointArray"=[], "Line Array"=[], "CircleArrayOUT"=[], "TPDetails"={"DistanceInfo"={"X"=0.0, "Y"=0.0, "X'"=0.0, "Y'"=0.0, "DX"=0.0, "DY"=0.0, "Distance Type"=""}, "Feature and Datum details"=[]}, "Value"=[], "Display Name"=0.0, "ROIArray"=[], "Update ROI "=FALSE} ("AlgoOut"), "VariableName"=w3140, "VariableType"="Value", "Value"=w3161) -> (w3160:T14)
        }
        frame "Circularity" {
          w3188 = T35 {"Point 1"={"X"=0.0, "Y"=0.0}, "Point 2"={"X"=0.0, "Y"=0.0}, "Center (Pixels)"={"X"=0.0, "Y"=0.0}, "Radius (Pixels)"=0.0}  # Circle
          n1169 = Index Array(array=w3208) -> (element=w3207:T42)  [unwired: 1 in]
          n1170 = Index Array(array=w3181) -> (element=w3176:T26)  [unwired: 1 in]
          n1171 = Unbundle By Name(w3207) -> ()  [unwired: 1 out]
          n1172 = Unbundle By Name(w3176) -> ("First Edges"=w3198:T15[], "CircleDetected.Center (Pixels)"=w3201:cluster{"X":sgl, "Y":sgl}, "Indexes of Points Used"=w3200:i32[])
          n1173 = Array Size(array=w3181) -> (size(s)=w3180:i32)
          n1174 = Equal?(x=w3180, y=1) -> (x = y?=w3178:bool)
          n1175 = for {
            tunnel: w3198 -> [w3226] mode=indexing
            tunnel: [w3225] -> w3199 mode=indexing
            n1176 = Unbundle By Name(w3226) -> ("Location (Pixel)"=w3225:cluster{"X":sgl, "Y":sgl})
          }
          n1177 = case shown="True" w3178 {
            tunnel: [w3214 w3224] -> w3211
            tunnel: w3210 -> [w3214 w3223]
            tunnel: w3209 -> [_ w3222]
            tunnel: [sgl nan ("Circularity") w3221] -> w3202
            tunnel: w3201 -> [_ w3220]
            tunnel: w3200 -> [_ w3219]
            tunnel: w3199 -> [_ w3218]
            tunnel: w3197 -> [_ w3217]
            tunnel: w3196 -> [_ w3216]
            tunnel: [w3212 w3215] -> w3177
            tunnel: w3176 -> [_ w3215]
            frame False {
              w3212 = T30 {"CircleDetected"={"Center (Pixels)"={"X"=nan, "Y"=nan}, "Radius (Pixels)"=nan}, "First Edges"=[], "Indexes of Points Used"=[], "Start Point"={"X"=0.0, "Y"=0.0}, "End Point"={"X"=0.0, "Y"=0.0}}  # Circle NaN Array
            }
            frame True {
              n1178 = call "circularity.vi"("Edge Points Array"=w3218, "Calibrated Image"=w3222, "Center"=w3220, "Indexes of Points Used"=w3219, "Converstion Factor 2"=w3217, "error in"=w3223, "Converstion Factor"=w3216) -> ("Circularity"=w3221:sgl, "error out"=w3224:errorcluster)  [unwired: 7 in]
            }
          }
          n1179 = Unbundle By Name(w3177) -> ("CircleDetected.Center (Pixels)"=w3190:cluster{"X":dbl, "Y":dbl}, "CircleDetected.Radius (Pixels)"=w3189:dbl)
          n1180 = Unbundle By Name(w3190) -> ("X"=w3193:dbl)
          n1181 = Add(x=w3193, y=w3189) -> (x+y=w3195:dbl)
          n1182 = Subtract(x=w3193, y=w3189) -> (x-y=w3194:dbl)
          n1183 = Bundle By Name(cluster=w3190, "X"=w3195) -> (w3192:cluster{"X":dbl, "Y":dbl})
          n1184 = Bundle By Name(cluster=w3190, "X"=w3194) -> (w3191:cluster{"X":dbl, "Y":dbl})
          n1185 = Bundle By Name(cluster=w3188, "Radius (Pixels)"=w3189, "Center (Pixels)"=w3190, "Point 1"=w3192, "Point 2"=w3191) -> (w3187:T35)
          n1186 = Build Array(w3187) -> (w3186:T28)
          n1187 = Bundle By Name(cluster=w3183, "PointForOverlays.Circle"=w3186, "Measurment Type"="Circularity", "Measurment Name"=w3184) -> (w3182:T12)
          n1188 = Build Array(w3202) -> (w3204:sgl[])
          n1189 = Bundle By Name(cluster=T14 {"VariableName"="", "VariableType"="", "Co-sys Reference"={"Base Co-sys Reference"={"Origin"={"X"=0.0, "Y"=0.0}, "Angle (deg)"=0.0, "Axis Reference"=0, "Scale"=0.0}, "New Co-sys Reference"={"Origin"={"X"=0.0, "Y"=0.0}, "Angle (deg)"=0.0, "Axis Reference"=0, "Scale"=0.0}}, "PointArray"=[], "Line Array"=[], "CircleArrayOUT"=[], "TPDetails"={"DistanceInfo"={"X"=0.0, "Y"=0.0, "X'"=0.0, "Y'"=0.0, "DX"=0.0, "DY"=0.0, "Distance Type"=""}, "Feature and Datum details"=[]}, "Value"=[], "Display Name"=0.0, "ROIArray"=[], "Update ROI "=FALSE} ("AlgoOut"), "VariableName"=w3184, "VariableType"="Value", "Value"=w3204) -> (w3203:T14)
        }
        frame "Perpendicularity" {
          n1190 = Index Array(array=w3254) -> (element=w3253:T42)  [unwired: 1 in]
          n1191 = Unbundle By Name(w3253) -> ()  [unwired: 2 out]
          n1192 = Array Size(array=w3257) -> (size(s)=w3256:i32)
          n1193 = Index Array(array=w3257) -> (element #1=w3238:T23, element #2=w3235:T23)  [unwired: 2 in]
          n1194 = Not Equal?(x=w3238, y=w3235) -> (x != y?=w3241:T67)
          n1195 = Unbundle By Name(w3238) -> ("Line"=w3237:T24)
          n1196 = Unbundle By Name(w3241) -> ("Line.Point 1"=w3240:cluster{"X":bool, "Y":bool}, "Line.Point 2"=w3239:cluster{"X":bool, "Y":bool})
          n1197 = Equal?(x=w3256, y=2) -> (x = y?=w3228:bool)
          n1198 = Unbundle By Name(w3235) -> ("Line"=w3236:T24)
          n1199 = Unbundle By Name(w3240) -> ("X"=w3233:bool, "Y"=w3232:bool)
          n1200 = Unbundle By Name(w3239) -> ("X"=w3231:bool, "Y"=w3230:bool)
          n1201 = Compound Arithmetic op=OR(w3233, w3232, w3231, w3230) -> (w3229:bool)
          n1202 = And(x=w3228, y=w3229) -> (x .and. y?=w3227:bool)
          n1203 = case shown="True" w3227 {
            tunnel: w3265 -> [w3268 w3277]
            tunnel: [w3268 w3276] -> w3264
            tunnel: w3263 -> [_ w3275]
            tunnel: [nan ("Perpendicularity") w3274] -> w3258
            tunnel: w3237 -> [_ w3273]
            tunnel: w3236 -> [_ w3272]
            tunnel: w3252 -> [_ w3271]
            tunnel: w3251 -> [_ w3270]
            tunnel: [T23 {"Line"={"Point 1"={"X"=nan, "Y"=nan}, "Point 2"={"X"=nan, "Y"=nan}}, "Straight Edges"=[], "Used Edges"=[]} ("Line") w3269] -> w3234
            tunnel: w3235 -> [_ w3269]
            frame False {
            }
            frame True {
              n1204 = call "perperndicularity.vi"("Converstion Factor"=w3271, "Conversion Factor"=w3270, "error in (no error)"=w3277, "Line 2"=w3272, "Line 1"=w3273, "Calib Image"=w3275) -> ("error out"=w3276:errorcluster, "Perpendicularity"=w3274:dbl)  [unwired: 4 in]
            }
          }
          n1205 = Unbundle By Name(w3234) -> ("Line.Point 1"=w3250:cluster{"X":sgl, "Y":sgl}, "Line.Point 2"=w3249:cluster{"X":sgl, "Y":sgl})
          n1206 = Bundle By Name(cluster=T24 {"Point 1"={"X"=0.0, "Y"=0.0}, "Point 2"={"X"=0.0, "Y"=0.0}} ("Line"), "Point 1"=w3250, "Point 2"=w3249) -> (w3247:T24)
          n1207 = Build Array(w3247) -> (w3246:T31)
          n1208 = Bundle By Name(cluster=w3243, "PointForOverlays.Line"=w3246, "Measurment Name"=w3244, "Measurment Type"="Perpendicularity") -> (w3242:T12)
          n1209 = Build Array(w3258) -> (w3260:dbl[])
          n1210 = Bundle By Name(cluster=T14 {"VariableName"="", "VariableType"="", "Co-sys Reference"={"Base Co-sys Reference"={"Origin"={"X"=0.0, "Y"=0.0}, "Angle (deg)"=0.0, "Axis Reference"=0, "Scale"=0.0}, "New Co-sys Reference"={"Origin"={"X"=0.0, "Y"=0.0}, "Angle (deg)"=0.0, "Axis Reference"=0, "Scale"=0.0}}, "PointArray"=[], "Line Array"=[], "CircleArrayOUT"=[], "TPDetails"={"DistanceInfo"={"X"=0.0, "Y"=0.0, "X'"=0.0, "Y'"=0.0, "DX"=0.0, "DY"=0.0, "Distance Type"=""}, "Feature and Datum details"=[]}, "Value"=[], "Display Name"=0.0, "ROIArray"=[], "Update ROI "=FALSE} ("AlgoOut"), "VariableName"=w3244, "VariableType"="Value", "Value"=w3260) -> (w3259:T14)
        }
        frame "Symmetry" {
          n1211 = Index Array(array=w3303) -> (element=w3302:T42)  [unwired: 1 in]
          n1212 = Unbundle By Name(w3302) -> ()  [unwired: 2 out]
          n1213 = Array Size(array=w3306) -> (size(s)=w3305:i32)
          n1214 = Index Array(array=w3306) -> (element #1=w3290:T23, element #2=w3282:T23)  [unwired: 2 in]
          n1215 = Equal?(x=w3305, y=2) -> (x = y?=w3279:bool)
          n1216 = Unbundle By Name(w3290) -> ("Line"=w3289:T24)
          n1217 = Unbundle By Name(w3282) -> ("Line"=w3288:T24)
          n1218 = Not Equal?(x=w3289, y=w3288) -> (x != y?=w3287:T49)
          n1219 = Unbundle By Name(w3287) -> ("Point 1.X"=w3283:bool, "Point 1.Y"=w3284:bool, "Point 2.X"=w3285:bool, "Point 2.Y"=w3286:bool)
          n1220 = Compound Arithmetic op=OR(w3283, w3284, w3285, w3286) -> (w3280:bool)
          n1221 = And(x=w3280, y=w3279) -> (x .and. y?=w3278:bool)
          n1222 = case shown="True" w3278 {
            tunnel: [sgl nan ("Symmetry") w3326] -> w3310
            tunnel: [w3316 w3325] -> w3309
            tunnel: w3308 -> [_ w3324]
            tunnel: w3307 -> [w3316 w3323]
            tunnel: w3289 -> [_ w3322]
            tunnel: w3288 -> [_ w3321]
            tunnel: w3301 -> [_ w3320]
            tunnel: w3300 -> [_ w3319]
            tunnel: w3282 -> [_ w3318]
            tunnel: [T23 {"Line"={"Point 1"={"X"=nan, "Y"=nan}, "Point 2"={"X"=nan, "Y"=nan}}, "Straight Edges"=[], "Used Edges"=[]} ("Line") w3318] -> w3281
            frame False {
            }
            frame True {
              n1223 = call "symmetry_int.vi"("Converstion Factor 2"=w3320, "Converstion Factor"=w3319, "error in"=w3323, "Line 2"=w3321, "Line 1"=w3322, "Calibrated Image"=w3324) -> ("error out"=w3325:errorcluster, "Symmetry"=w3326:sgl)  [unwired: 4 in]
            }
          }
          n1224 = Unbundle By Name(w3281) -> ("Line.Point 1"=w3299:cluster{"X":sgl, "Y":sgl}, "Line.Point 2"=w3298:cluster{"X":sgl, "Y":sgl})
          n1225 = Bundle By Name(cluster=T24 {"Point 1"={"X"=0.0, "Y"=0.0}, "Point 2"={"X"=0.0, "Y"=0.0}} ("Line"), "Point 1"=w3299, "Point 2"=w3298) -> (w3296:T24)
          n1226 = Build Array(w3296) -> (w3295:T31)
          n1227 = Bundle By Name(cluster=w3292, "PointForOverlays.Line"=w3295, "Measurment Name"=w3293, "Measurment Type"="Symmetricity") -> (w3291:T12)
          n1228 = Build Array(w3310) -> (w3312:sgl[])
          n1229 = Bundle By Name(cluster=T14 {"VariableName"="", "VariableType"="", "Co-sys Reference"={"Base Co-sys Reference"={"Origin"={"X"=0.0, "Y"=0.0}, "Angle (deg)"=0.0, "Axis Reference"=0, "Scale"=0.0}, "New Co-sys Reference"={"Origin"={"X"=0.0, "Y"=0.0}, "Angle (deg)"=0.0, "Axis Reference"=0, "Scale"=0.0}}, "PointArray"=[], "Line Array"=[], "CircleArrayOUT"=[], "TPDetails"={"DistanceInfo"={"X"=0.0, "Y"=0.0, "X'"=0.0, "Y'"=0.0, "DX"=0.0, "DY"=0.0, "Distance Type"=""}, "Feature and Datum details"=[]}, "Value"=[], "Display Name"=0.0, "ROIArray"=[], "Update ROI "=FALSE} ("AlgoOut"), "VariableName"=w3293, "VariableType"="Value", "Value"=w3312) -> (w3311:T14)
        }
        frame "TruePosition" {
          w3342 = "TPValue"  # VariableType
          w3357 = 0.0  # Position Tolerance
          w3365 = T35 {"Point 1"={"X"=0.0, "Y"=0.0}, "Point 2"={"X"=0.0, "Y"=0.0}, "Center (Pixels)"={"X"=0.0, "Y"=0.0}, "Radius (Pixels)"=0.0}  # Overlay Circle
          n1230 = Unbundle By Name(w3380) -> ("Nominal X/R"=w3379:dbl, "Nominal Y/A"=w3378:dbl, "Disatnce Type"=w3328:string)
          n1231 = Index Array(array=w3366) -> (element=w3374:T26)  [unwired: 1 in]
          n1232 = Unbundle By Name(w3374) -> ("CircleDetected.Radius (Pixels)"=w3359:dbl, "CircleDetected.Center (Pixels)"=w3360:cluster{"X":sgl, "Y":sgl})
          n1233 = case shown="\"Polar\"" w3328 {
            tunnel: w3379 -> [w3415 w3420]
            tunnel: w3378 -> [w3414 w3419]
            tunnel: [w3415 w3418] -> w3334
            tunnel: [w3414 w3417] -> w3333
            tunnel: [nan ("qv") w3416] -> w3373
            frame "Cartesian", Default {
              # "Input is in Cartesian form"
            }
            frame "Polar" {
              # "Input is in Polar form"
              n1234 = call "polar to cartesian conversion.vi"("Angle"=w3419, "Radius"=w3420) -> ("qv"=w3416:dbl, "Y"=w3417:dbl, "x"=w3418:dbl)  [unwired: 7 in]
            }
          }
          n1235 = call "TP.vi"("Reference"=w3376, "Feature Coordinates"=w3360, "Nominal distance along X axis"=w3334, "nominal distance along Y axis"=w3333, "Calibrated Image"=w3367, 5:"conversion factor"=w3375, 6:"conversion factor"=w3368, "error in"=w3377) -> ("TP"=w3335:dbl, "delX"=w3330:dbl, "delY"=w3329:dbl, "Measured distance along X axis"=w3372:dbl, "Measured distance along y axis"=w3371:dbl, "error out"=w3355:errorcluster)  [unwired: 14 in]
          n1236 = for {
            tunnel: w3327 -> [w3396] mode=indexing
            tunnel: [w3384] -> w3343 mode=indexing
            tunnel: [w3394] -> w3344 mode=indexing
            tunnel: [w3393] -> w3345 mode=indexing
            tunnel: [w3385] -> w3338 mode=indexing if=w3382
            n1237 = Unbundle By Name(w3396) -> ("Feature Type"=w3393:string, "Feature Name"=w3386:string, "Measurement Type"=w3392:string, "Measurement Position"=w3391:string, "Measurement Value"=w3390:dbl, "LSL"=w3389:dbl, "USL"=w3388:dbl, "Measurement Name"=w3383:string)
            n1238 = case shown="\"MMC\"" w3392 {
              selector: w3392 -> [_ w3400]
              tunnel: w3388 -> [_ w3405]
              tunnel: w3389 -> [_ w3404]
              tunnel: w3390 -> [_ w3403]
              tunnel: w3391 -> [_ w3402]
              tunnel: [w3398 w3401] -> w3384
              tunnel: [FALSE TRUE] -> w3382
              frame Default {
                w3398 = 0.0  # Bonus value
              }
              frame "MMC" {
                n1239 = call "Bonus calculator.vi"("MMC/RFS"=w3400, "INNER/OUTER"=w3402, "Measured value"=w3403, "LSL"=w3404, "USL"=w3405) -> ("Bonus value"=w3401:dbl)  [unwired: 10 in]
              }
            }
            n1240 = Bundle By Name(cluster=T40 {"Measurement name"="", "MMC"=FALSE, "Bonus"=0.0} ("Feature and Datum details"), "MMC"=w3382, "Bonus"=w3384, "Measurement name"=w3383) -> (w3385:T40)
            n1241 = Bundle By Name(cluster=T41 {"Measurement name"="", "Enable measurement"=FALSE} ("Feature and Datum details"), "Measurement name"=w3386, "Enable measurement"=w3382) -> (w3394:T41)
          }
          n1242 = Unbundle By Name(w3360) -> ("X"=w3362:sgl)
          n1243 = Add(x=w3362, y=w3359) -> (x+y=w3363:dbl)
          n1244 = case shown="\"Polar\"" w3328 {
            tunnel: w3373 -> [_ w3412]
            tunnel: w3372 -> [w3407 w3411]
            tunnel: w3371 -> [w3406 w3410]
            tunnel: [w3407 w3409] -> w3332
            tunnel: [w3406 w3408] -> w3331
            frame "Cartesian", Default {
            }
            frame "Polar" {
              n1245 = call "cartesian to polar conversion.vi"("qv"=w3412, "measured distance \nalong Y axis"=w3410, "measured distance \nalong X axis"=w3411) -> ("deta"=w3408:dbl, "R"=w3409:dbl)  [unwired: 7 in]
            }
          }
          n1246 = Bundle By Name(cluster=w3360, "X"=w3363) -> (w3361:cluster{"X":sgl, "Y":sgl})
          n1247 = Bundle By Name(cluster=w3365, "Center (Pixels)"=w3360, "Radius (Pixels)"=w3359, "Point 1"=w3361, "Point 2"=w3361) -> (w3364:T35)
          n1248 = Build Array(w3364) -> (w3358:T28)
          n1249 = Search 1D Array(1D array=w3345, element="Datum2") -> (index of element=w3350:i32)  [unwired: 1 in]
          n1250 = Search 1D Array(1D array=w3345, element="Feature") -> (index of element=w3353:i32)  [unwired: 1 in]
          n1251 = Search 1D Array(1D array=w3345, element="Datum1") -> (index of element=w3349:i32)  [unwired: 1 in]
          n1252 = Add Array Elements(numeric array=w3343) -> (sum=w3337:dbl)
          n1253 = Index Array "Datum1 Index Array"(array=w3343, index=w3349) -> (element=w3347:dbl)
          n1254 = Index Array "Datum2 Index Array"(array=w3343, index=w3350) -> (element=w3346:dbl)
          n1255 = Index Array "Feature Index Array"(array=w3343, index=w3353) -> (element=w3348:dbl)
          n1256 = Build Array(w3335, w3330, w3329, w3357, w3348, w3347, w3346) -> (w3356:dbl[])
          n1257 = Build Array(w3335, w3337) -> (w3341:dbl[])
          n1258 = Bundle By Name(cluster=w3381, "Measurment Name"=w3336, "Measurment Type"="TruePosition", "PointForOverlays.Circle"=w3358, "PointForOverlays.True position.Measurement details"=w3344, "Result"=w3356) -> (w3370:T12)
          n1259 = Bundle By Name(cluster=T14 {"VariableName"="", "VariableType"="", "Co-sys Reference"={"Base Co-sys Reference"={"Origin"={"X"=0.0, "Y"=0.0}, "Angle (deg)"=0.0, "Axis Reference"=0, "Scale"=0.0}, "New Co-sys Reference"={"Origin"={"X"=0.0, "Y"=0.0}, "Angle (deg)"=0.0, "Axis Reference"=0, "Scale"=0.0}}, "PointArray"=[], "Line Array"=[], "CircleArrayOUT"=[], "TPDetails"={"DistanceInfo"={"X"=0.0, "Y"=0.0, "X'"=0.0, "Y'"=0.0, "DX"=0.0, "DY"=0.0, "Distance Type"=""}, "Feature and Datum details"=[]}, "Value"=[], "Display Name"=0.0, "ROIArray"=[], "Update ROI "=FALSE} ("AlgoOut"), "VariableName"=w3336, "Value"=w3341, "TPDetails.DistanceInfo.X"=w3334, "TPDetails.DistanceInfo.Y"=w3333, "TPDetails.DistanceInfo.X'"=w3332, "TPDetails.DistanceInfo.Y'"=w3331, "TPDetails.DistanceInfo.DX"=w3330, "TPDetails.DistanceInfo.DY"=w3329, "TPDetails.DistanceInfo.Distance Type"=w3328, "TPDetails.Feature and Datum details"=w3338, "VariableType"=w3342) -> (w3339:T14)
        }
        frame "----3D----" {
        }
        frame "DepthfromReference" {
          w3433 = T14 {"VariableName"="", "VariableType"="", "Co-sys Reference"={"Base Co-sys Reference"={"Origin"={"X"=0.0, "Y"=0.0}, "Angle (deg)"=0.0, "Axis Reference"=0, "Scale"=0.0}, "New Co-sys Reference"={"Origin"={"X"=0.0, "Y"=0.0}, "Angle (deg)"=0.0, "Axis Reference"=0, "Scale"=0.0}}, "PointArray"=[], "Line Array"=[], "CircleArrayOUT"=[], "TPDetails"={"DistanceInfo"={"X"=0.0, "Y"=0.0, "X'"=0.0, "Y'"=0.0, "DX"=0.0, "DY"=0.0, "Distance Type"=""}, "Feature and Datum details"=[]}, "Value"=[], "Display Name"=0.0, "ROIArray"=[], "Update ROI "=FALSE}  # AlgoOut
          n1260 = Index Array(array=w3436) -> (element=w3429:cluster{"X":sgl, "Y":sgl})  [unwired: 1 in]
          n1261 = call "Interpolate.vi"("error in (no error)"=w3435, "Point"=w3429) -> ("error IO"=w3434:errorcluster, "Z value"=w3427:dbl)  [unwired: 8 in]
          n1262 = Build Array(w3429) -> (w3428:cluster{"X":sgl, "Y":sgl}[])
          n1263 = Build Array(w3427) -> (w3426:dbl[])
          n1264 = Bundle By Name(cluster=w3430, "Measurment Type"="Depth", "Measurment Name"=w3425, "PointForOverlays.Points.Points"=w3428) -> (w3424:T12)
          n1265 = Bundle By Name(cluster=w3433, "VariableName"=w3425, "VariableType"="Value", "Value"=w3426) -> (w3423:T14)
        }
      }
      n1266 = flat-sequence {
        tunnel: [w147] -> w124
        tunnel: w123 -> [w147]
        frame #0 {
          n1267 = Request Deallocation(TRUE ("flag")) -> ()
        }
      }
    }
    frame Error {
      n1268 = Index Array(array=w3437) -> (element=w3438:T42)  [unwired: 1 in]
      n1269 = Unbundle By Name(w3438) -> ()  [unwired: 2 out]
    }
  }
  "error out" <- w27
  "AlgoOut Array out" <- w26
  "overlayDetails Out" <- w16
